vi "SubVgDummi.vi"(0 "Target Voltage, V":dbl=1.0 min=-4.0 max=4.0 step=0.1 format="%.4f", 2 "Sweep rate, V/min":dbl=0.1 min=0.0 max=1.0 step=0.01 format="%.4f", 3 "Custom Folder":string, 5 "optional Bias (V)":dbl=1e-08) -> ()   [LabVIEW 2013]
uses:
  <vilib>/Utility/file.llb/Write To Spreadsheet File (DBL).vi
panel:
  out "Numeric 4":i32
  in  "Commutator":bool
  in  "Commute SorceMeter":enum32{"Radio Selection 1", "Radio Selection 2"}(radio)
  out "Numeric 3":i32
  in  "Channel 2 (Vnano3b)":bool
  in  "Channel 1 (Vnano3)":bool
  out "Numeric":i32
  in  "Capacitance (C) and Loss (L)":bool
  in  "Magnetic Field (B)":bool
  in  "Current (Ik3)":bool
  in  "Voltage (Vk3)":bool
  in  "Current (Ik2)":bool
  in  "Voltage (Vk2)":bool
  in  "Channel 2 (Vnano2b)":bool
  in  "Channel 1 (Vnano2)":bool
  in  "Thermometer 1 (T1)":bool=TRUE
  in  "Channel 2 (Vnano1b)":bool
  in  "Channel 1 (Vnano1)":bool
  in  "Current (Ik1)":bool=TRUE
  in  "Voltage (Vk1)":bool
  out "Numeric Current":dbl
  out "Main Keithly2400 address":string="12"
  out "Delib Time delay":i32
  in  "points at each Vg":i32=1
  out "XY Graph":cluster{dbl[], dbl[]}(graph)={[1.0, 0.8, 0.6000000000000001, 0.4000000000000001, 0.20000000000000007, 5.551115123125783e-17, -0.19999999999999996, -0.39999999999999997, -0.6, -0.8, -1.0], [0.03352775, 0.056811, 0.03911575, 0.04330675, -0.02468015, 0.011641600000000002, 0.10151450000000001, 0.12386675000000001, 0.08288825000000001, -0.00186266, -0.038650000000000004]}
  in  "Time btw \npoints, sec":dbl=1.0 format="%.2f"
  out "Array 2":dbl[][](array[numeric])
  out "array for data":dbl[](array[numeric])
  out "Numeric 2":dbl
  out "Array":string[](array[string])
  in  "Addr 1 lock-in oop":bool
  in  "Ring":u16(ring) caption="Y-axis:" items=["Vg", "I", "R1", "R1oop", "R2", "R2oop", "R3", "R3oop", "Ik1", "T1", "B"]
  out "String":string
  out "Data file:":path
  in  "Set compliance limit, mkA":dbl=0.05 min=0.0 max=1.0 step=0.01 format="%.3f"
  in  "error in (no error)":errorcluster
  in  "Ring 3":u16(ring)=1 items=["1 kOhm", "10 kOhm", "100 kOhm", "1 Mohm", "10 mOhm"]
  in  "Ring 2":u16(ring)=3 items=["1 kOhm", "10 kOhm", "100 kOhm", "1 Mohm", "10 mOhm"]
  in  "Fixed Current mkA":dbl=1.0
  in  "Current is:":T1(radio)
  in  "Ressitance measurements?":bool=TRUE
  in  "Addr 5 lock-in oop":bool
  in  "Addr 4 lock-in oop":bool
  in  "Addr 3 lock-in oop":bool
  in  "Addr 2 lock-in oop":bool
  in  "Addr 5 lock-in":bool
  in  "Addr 4 lock-in":bool
  in  "Addr 3 lock-in":bool=TRUE
  in  "Addr 2 lock-in":bool=TRUE
  in  "Addr 1 lock-in":bool=TRUE
  # "Keithley 2400: address 12"
  # "SourceMeters"
  # "Nanovoltmeters"
  # "Temperature"
  # "Main"
  # "Magnetic Field"
  # "(not recommended, too slow)"
  # "Capacitance & Loss"
  # "(not recommended, too slow)"
  # "(not recommended, too slow)"
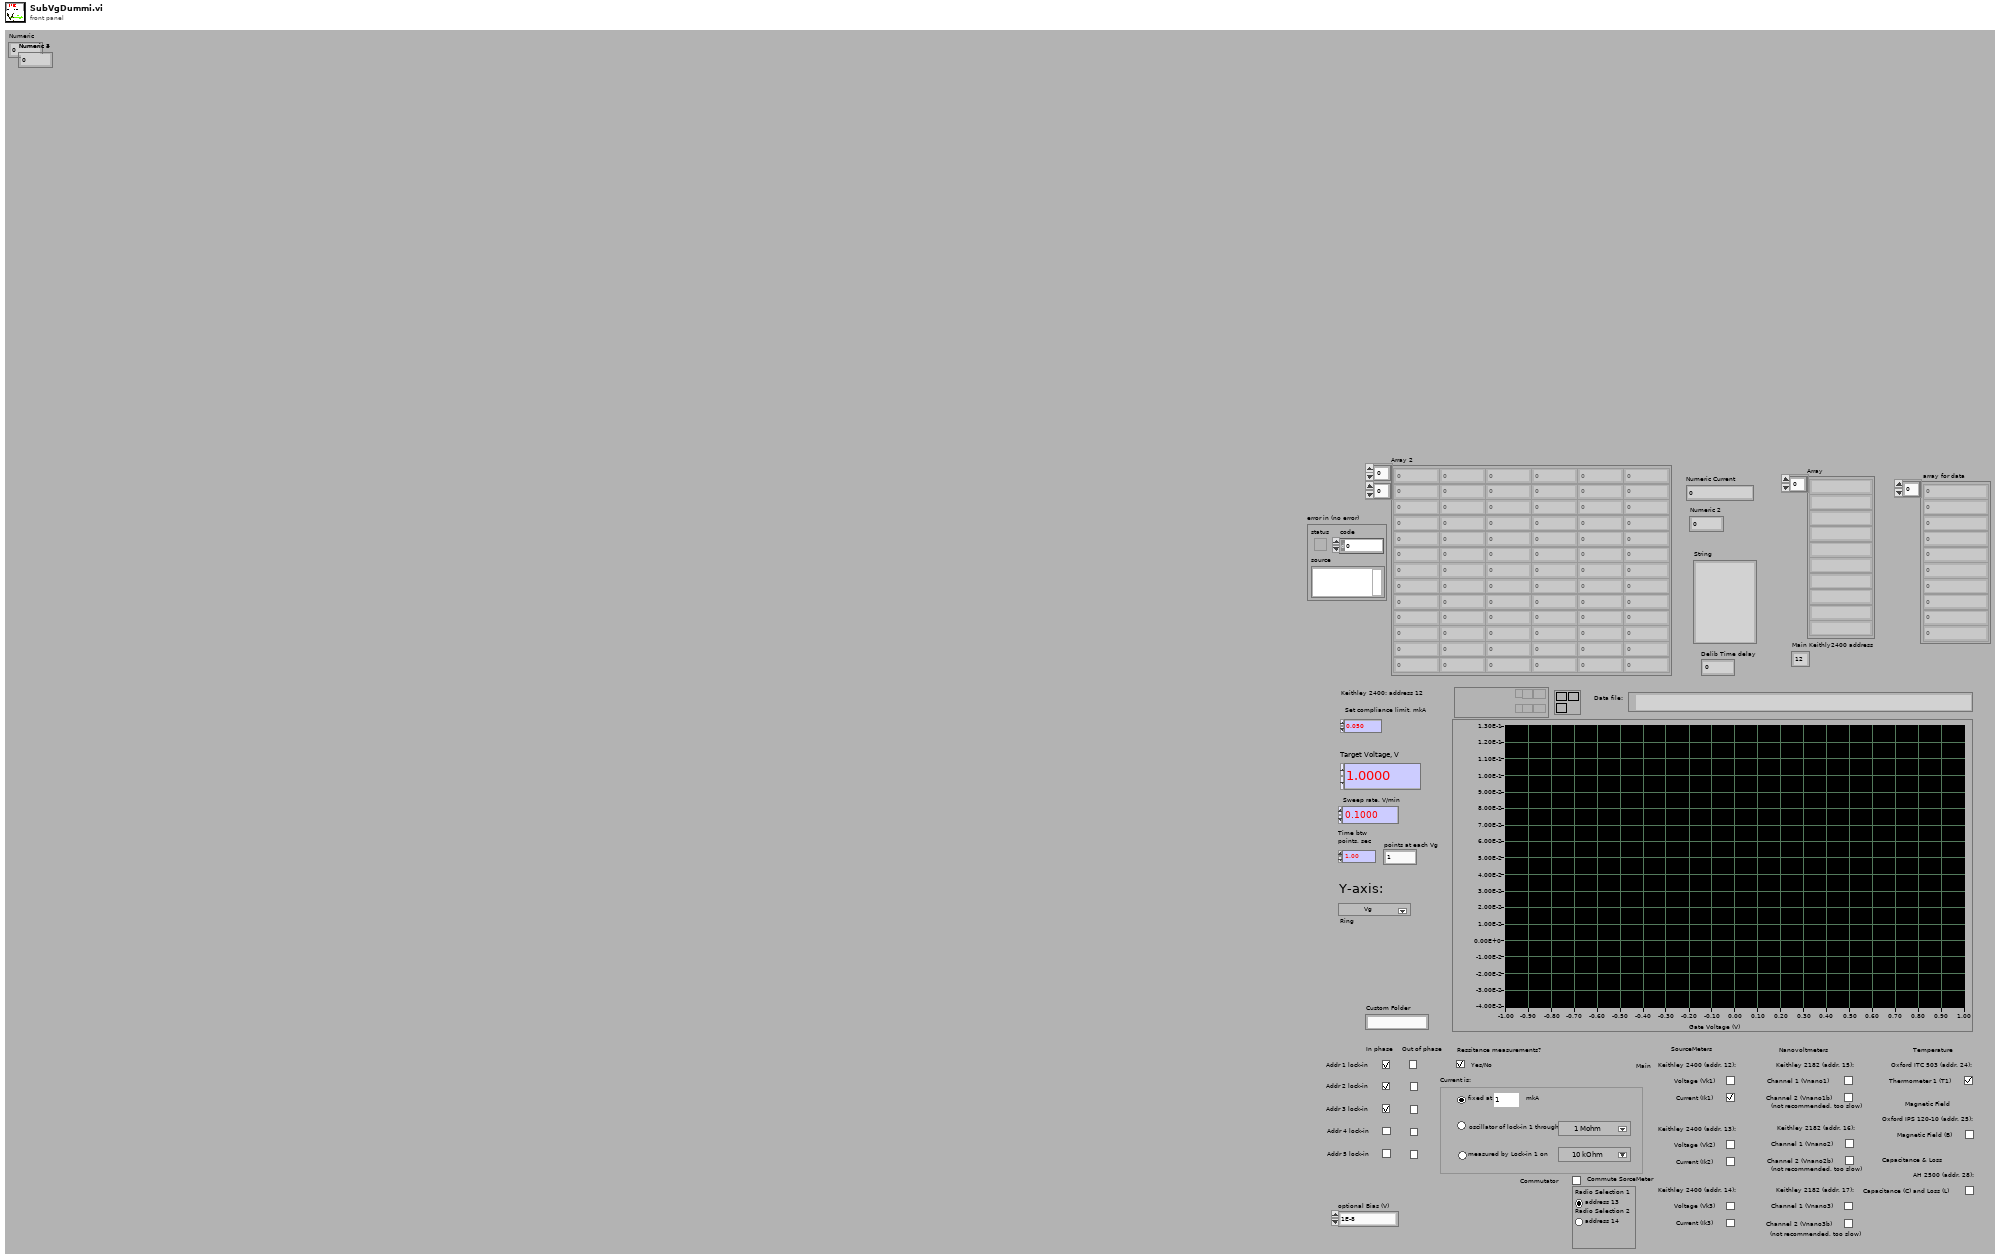
[diagram p1: front panel]
types:
  T1 = enum32{"Radio Selection 1", "Radio Selection 2", "Radio Selection 3"}
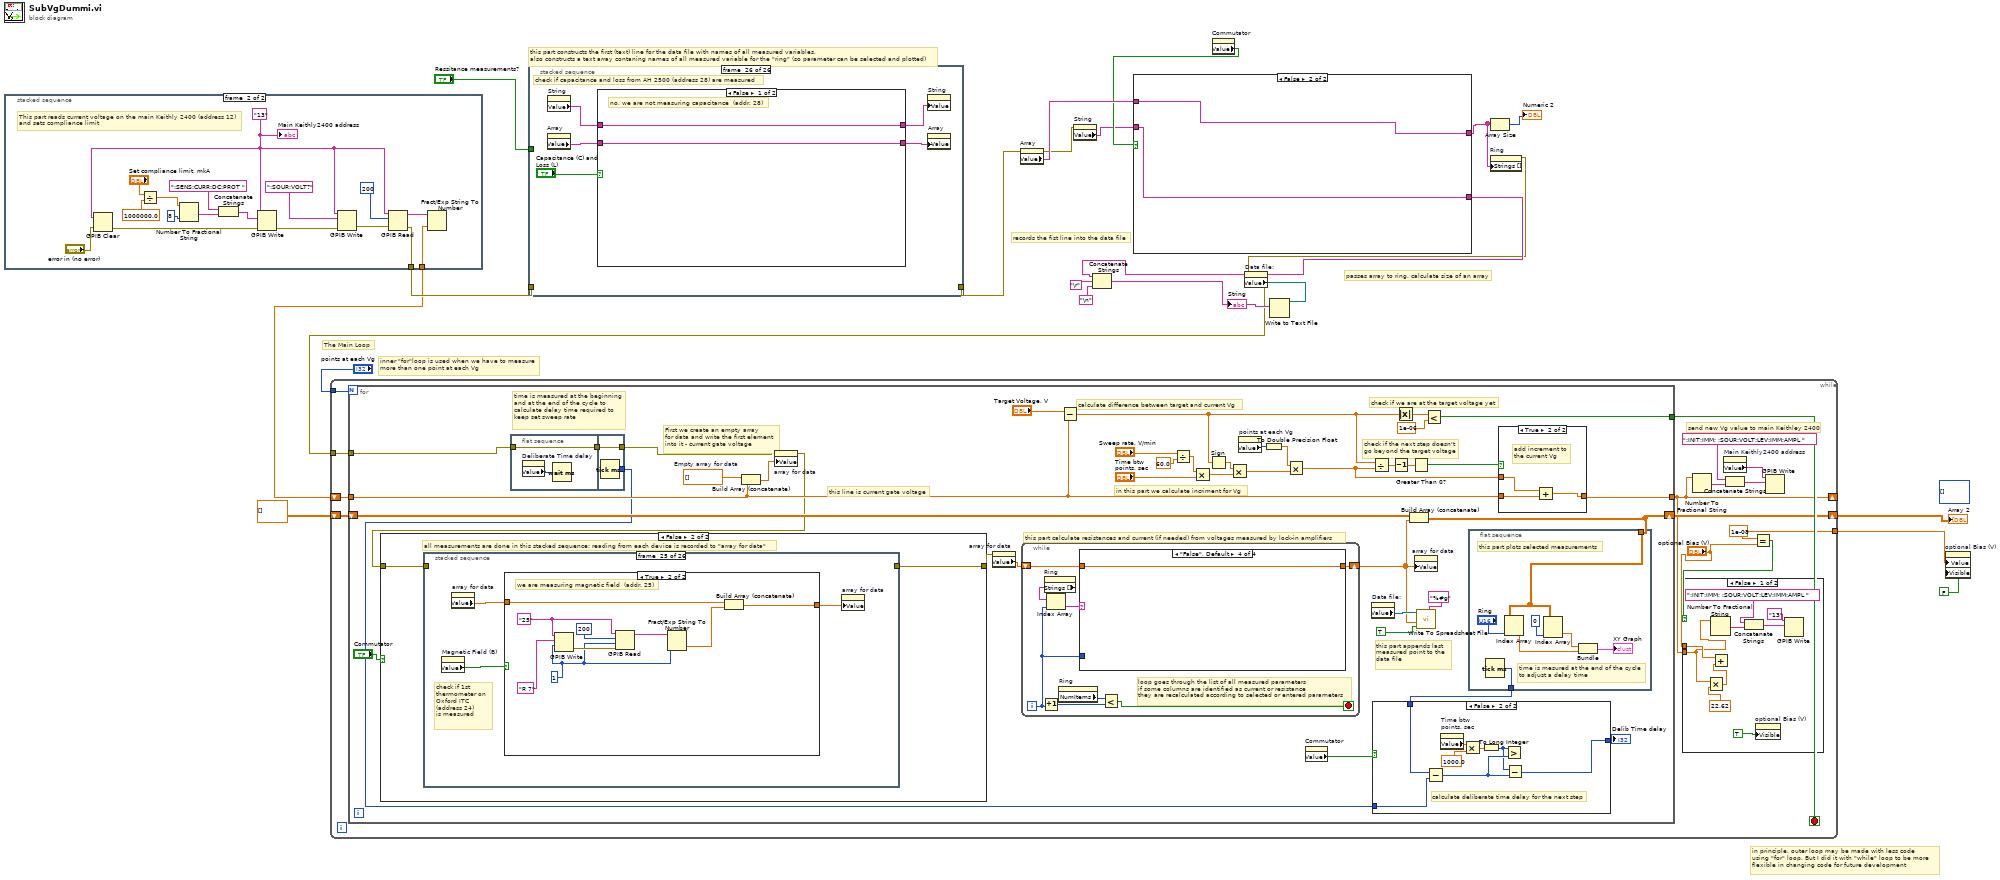
[diagram p0: block diagram]
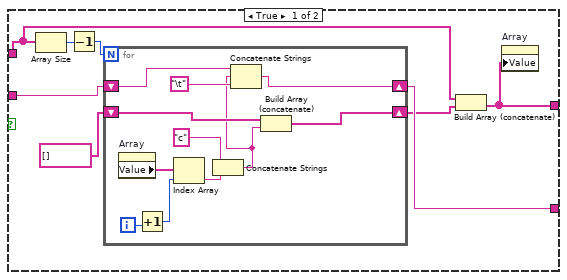
[diagram p2: hidden frame]
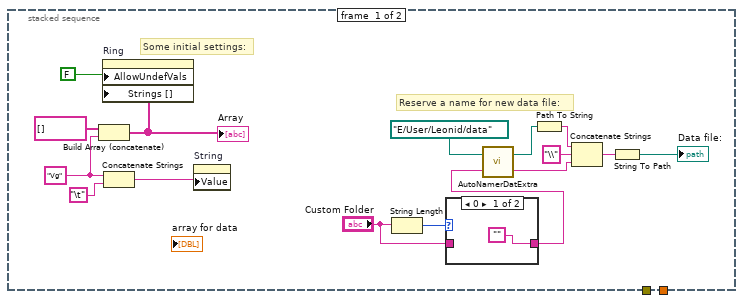
[diagram p3: hidden frame]
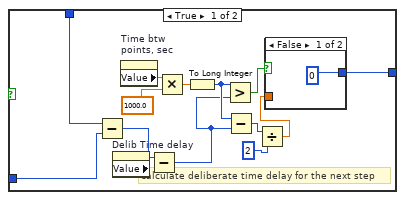
[diagram p6: hidden frame]
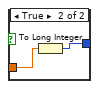
[diagram p7: hidden frame]
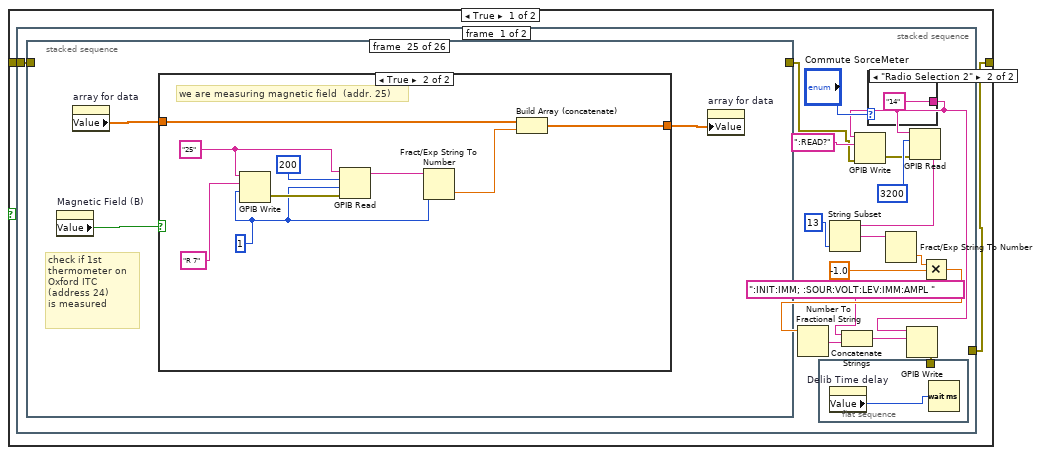
[diagram p8: hidden frame]
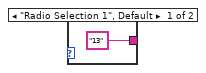
[diagram p9: hidden frame]
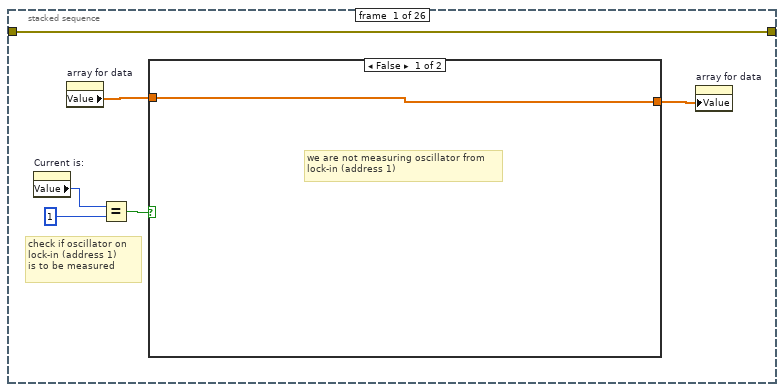
[diagram p10: hidden frame]
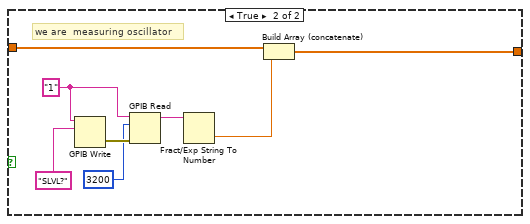
[diagram p11: hidden frame]
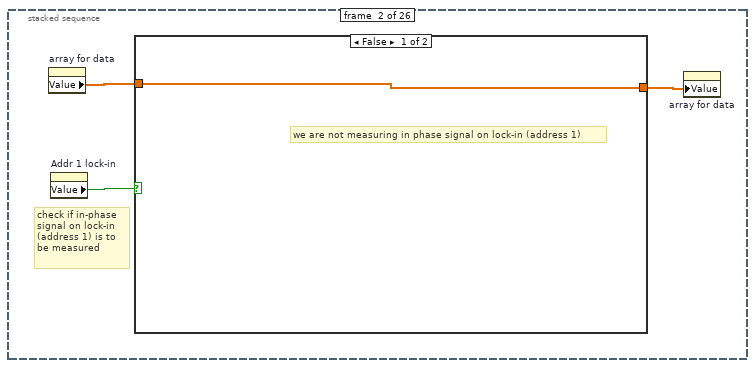
[diagram p12: hidden frame]
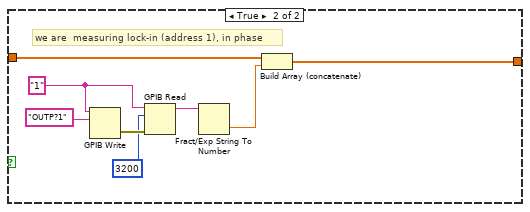
[diagram p13: hidden frame]
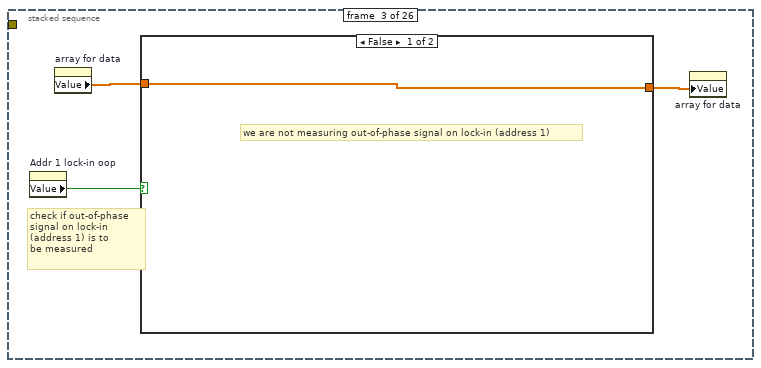
[diagram p14: hidden frame]
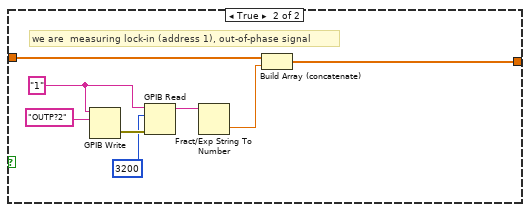
[diagram p15: hidden frame]
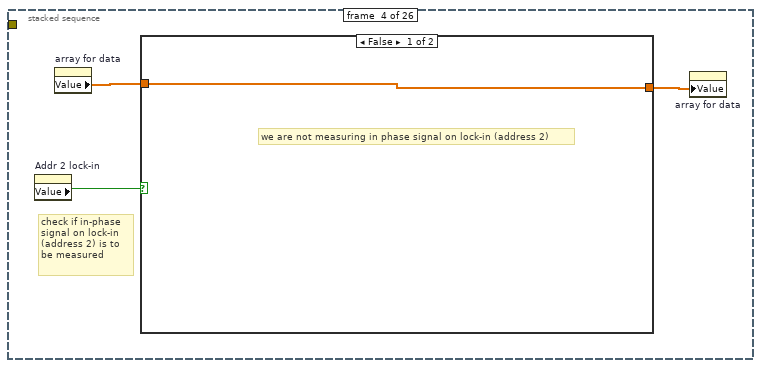
[diagram p16: hidden frame]
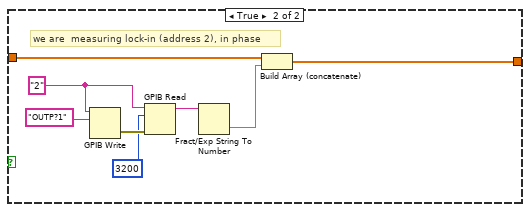
[diagram p17: hidden frame]
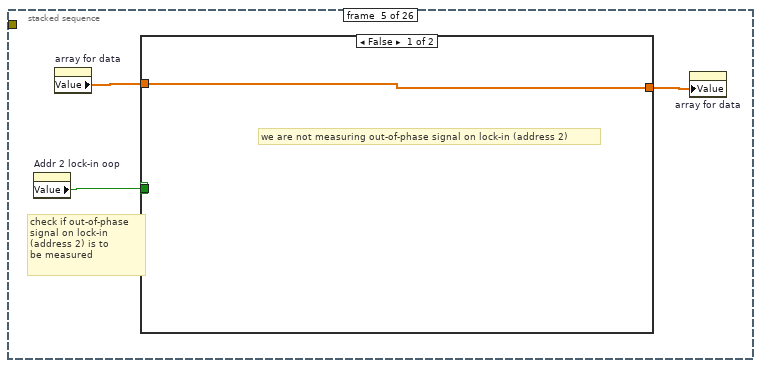
[diagram p18: hidden frame]
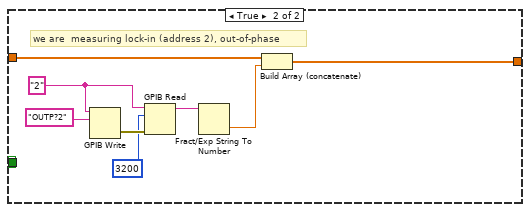
[diagram p19: hidden frame]
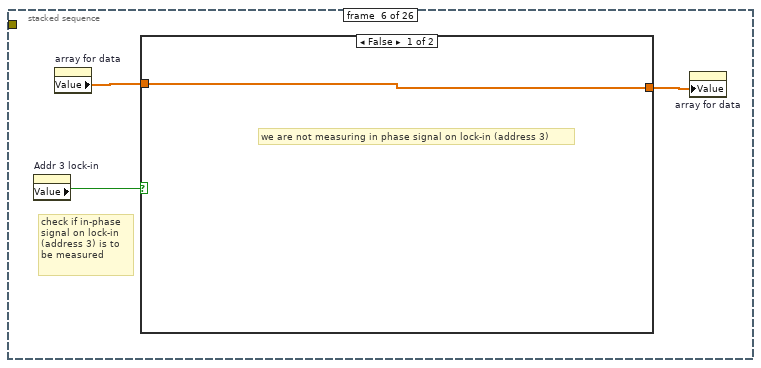
[diagram p20: hidden frame]
diagram:
  (unwired) i32[][] []
  # "passes array to ring, calculate size of an array"
  # "in principle, outer loop may be made with less code\nusing \"for\" loop. But I did it with \"while\" loop to be more \nflexible in changing code for future development"
  # "inner \"for\"loop is used when we have to measure\nmore than one point at each Vg"
  # "The Main Loop"
  # "records the fist line into the data file"
  # "this part constructs the first (text) line for the data file with names of all measured variables,\nalso constructs a text array contaning names of all measured variable for the \"ring\" (so parameter can be selected and plotted)"
  n1 = stacked-sequence {
    tunnel: [_ w43] -> w22
    tunnel: [_ w42] -> w9
    frame #0 {
      w28 = "Vg"
      # "Some initial settings:"
      # "Reserve a name for new data file:"
      n2 = Build Array (concatenate)(string[] [], w28) -> (w30:string[])
      "Array" <- w30
      n3 = property on="Ring" class="Ring (strict)"("AllowUndefVals"=FALSE, "Strings []"=w30) -> ()  [unwired: 2 in, 2 out]
      n4 = Concatenate Strings(w28, "\t") -> (w29:string)
      n5 = property on="String" class="Str"("Value"=w29) -> ()  [unwired: 2 in, 2 out]
      n6 = String Length(string="Custom Folder") -> (length=w25:i32)
      n7 = case shown="0" w25 {
        tunnel: "Custom Folder" -> [_ w40]
        tunnel: ["" w40] -> w23
        frame 0 {
        }
        frame 1, Default {
        }
      }
      n8 = call "AutoNamerDatExtra.vi"("ExtraString"=w23, "Custom User Path"=path "E:/User/Leonid/data") -> ("String"=w38:string, "Path"=w37:path)
      n9 = Path To String(path=w37) -> (string=w32:string)
      n10 = Concatenate Strings(w32, "\\", w38) -> (w34:string)
      n11 = String To Path(string=w34) -> (path=→"Data file:":path)
    }
    frame #1 {
      w41 = "13"
      # "This part reads current voltage on the main Keithly 2400 (address 12)\nand sets compliance limit"
      n12 = GPIB Clear(2:"error in (no error)", 3:w41) -> (0:w50:errorcluster)  [unwired: 1 out]
      n13 = Divide(x="Set compliance limit, mkA", y=1000000.0) -> (x/y=w56:dbl)
      n14 = Number To Fractional String(number=w56, precision (6)=i16 8) -> (F-format string=w52:string)  [unwired: 2 in]
      n15 = Concatenate Strings(":SENS:CURR:DC:PROT " ("data"), w52) -> (w51:string)
      n16 = GPIB Write(0:w41, 1:w51, 3:w50) -> (6:w45:errorcluster)  [unwired: 2 in, 1 out]
      n17 = GPIB Write(0:w41, 1:":SOUR:VOLT?" ("data"), 3:w45) -> (6:w49:errorcluster)  [unwired: 2 in, 1 out]
      n18 = GPIB Read(0:w41, 1:200 ("byte count"), 3:w49) -> (5:w47:string, 7:w43:errorcluster)  [unwired: 2 in, 1 out]
      n19 = Fract/Exp String To Number(string=w47) -> (number=w42:dbl)  [unwired: 3 in, 1 out]
      "Main Keithly2400 address" <- w41
    }
  }
  n20 = stacked-sequence {
    tunnel: "Ressitance measurements?" -> [w65 w80 w104 w127 w145 w163 w181 w199 w217 w235 w253 _ _ _ _ _ _ _ _ _ _ _ _ _ _ _]
    tunnel: w22 -> [_ w77 _ _ _ _ _ _ _ _ _ _ _ _ _ _ _ _ _ _ _ _ _ _ _ _]
    tunnel: [_ w77 _ _ _ _ _ _ _ _ _ _ _ _ _ _ _ _ _ _ _ _ _ _ _ _] -> w19
    frame #0 {
      # "check if oscillator of  lock-in (address 1) is to be measured"
      n21 = property on="Array" class="Arr (strict)"() -> ("Value"=w60:string[])  [unwired: 2 in, 2 out]
      n22 = property on="String" class="Str"() -> ("Value"=w64:string)  [unwired: 2 in, 2 out]
      n23 = Equal?(x="Current is:", y=1) -> (x = y?=w61:bool)
      n24 = case shown="False" w61 {
        tunnel: w65 -> [_ _]
        tunnel: [w67 w68] -> w63
        tunnel: w64 -> [w67 w71]
        tunnel: w60 -> [w66 w70]
        tunnel: [w66 w69] -> w59
        frame False {
          # "we are not measuring oscillator from\nlock-in (address 1)"
        }
        frame True {
          w72 = "I"
          # "we are  measuring oscillator"
          n25 = GPIB Clear(3:"1") -> ()  [unwired: 1 in, 2 out]
          n26 = Concatenate Strings(w71, w72, "\t") -> (w68:string)
          n27 = Build Array (concatenate)(w70, w72) -> (w69:string[])
        }
      }
      n28 = property on="Array" class="Arr (strict)"("Value"=w59) -> ()  [unwired: 2 in, 2 out]
      n29 = property on="String" class="Str"("Value"=w63) -> ()  [unwired: 2 in, 2 out]
    }
    frame #1 {
      # "check if lock-in (address 1) is to be measured"
      n30 = property on="Array" class="Arr (strict)"() -> ("Value"=w76:string[])  [unwired: 2 in, 2 out]
      n31 = property on="String" class="Str"() -> ("Value"=w79:string)  [unwired: 2 in, 2 out]
      n32 = case shown="False" "Addr 1 lock-in" {
        tunnel: w80 -> [_ w91]
        tunnel: [w83 w87] -> w78
        tunnel: w79 -> [w83 w86]
        tunnel: w76 -> [w82 w88]
        tunnel: [w82 w89] -> w75
        frame False {
          # "we are not measuring in phase signal from\nlock-in (address 1)"
        }
        frame True {
          # "are we measuring resistance?"
          n33 = GPIB Clear(3:"1") -> ()  [unwired: 1 in, 2 out]
          n34 = case shown="True" w91 {
            tunnel: ["V1" w93] -> w84
            frame False {
              # "no, we are not measuring resistanse;\nall lock-ins are measuring voltage"
            }
            frame True {
              # "are we measuring current as well?"
              n35 = property on="Current is:" class="RadioBtnsControl (strict)"() -> ("Value"=w95:T1)  [unwired: 2 in, 2 out]
              n36 = Equal?(x=w95, y=2) -> (x = y?=w96:bool)
              n37 = case shown="False" w96 {
                tunnel: ["R1" "I"] -> w93
                frame False {
                  # "no, we are not \nmeasuring current\nby lock-in \n(address 1); \nso this lock-in is \nmeasuring resistance"
                }
                frame True {
                  # "yes, we are measuring \ncurrent by lock-in \n(address 1) as \nvoltage drop on \nknown resistance"
                }
              }
            }
          }
          n38 = Concatenate Strings(w86, w84, "\t") -> (w87:string)
          n39 = Build Array (concatenate)(w88, w84) -> (w89:string[])
        }
      }
      n40 = property on="Array" class="Arr (strict)"("Value"=w75) -> ()  [unwired: 2 in, 2 out]
      n41 = property on="String" class="Str"("Value"=w78) -> ()  [unwired: 2 in, 2 out]
    }
    frame #2 {
      # "check if out-of-phase signal on  lock-in (address 1) is to be measured"
      n42 = property on="Array" class="Arr (strict)"() -> ("Value"=w101:string[])  [unwired: 2 in, 2 out]
      n43 = property on="String" class="Str"() -> ("Value"=w103:string)  [unwired: 2 in, 2 out]
      n44 = case shown="False" "Addr 1 lock-in oop" {
        tunnel: w104 -> [_ w114]
        tunnel: [w106 w110] -> w102
        tunnel: w103 -> [w106 w109]
        tunnel: w101 -> [w105 w111]
        tunnel: [w105 w112] -> w100
        frame False {
          # "we are not measuring iout-of-phase signal from\nlock-in (address 1)"
        }
        frame True {
          # "are we measuring resistance?"
          n45 = GPIB Clear(3:"1") -> ()  [unwired: 1 in, 2 out]
          n46 = case shown="True" w114 {
            tunnel: ["V1oop" w116] -> w107
            frame False {
              # "no, we are not measuring resistance;\nall lock-ins are measuring voltage"
            }
            frame True {
              # "are we measuring out-of-phase current as well?"
              n47 = property on="Current is:" class="RadioBtnsControl (strict)"() -> ("Value"=w118:T1)  [unwired: 2 in, 2 out]
              n48 = Equal?(x=w118, y=2) -> (x = y?=w119:bool)
              n49 = case shown="False" w119 {
                tunnel: ["R1oop" "Ioop"] -> w116
                frame False {
                  # "no, we are not \nmeasuring current\nby lock-in \n(address 1); so this \nlock-in is measuring\nout-of-phase resistance"
                }
                frame True {
                  # "yes, we are measuring \nout-of phase current \nby lock-in (address 1) \nas voltage drop on \nknown resistance"
                }
              }
            }
          }
          n50 = Concatenate Strings(w109, w107, "\t") -> (w110:string)
          n51 = Build Array (concatenate)(w111, w107) -> (w112:string[])
        }
      }
      n52 = property on="Array" class="Arr (strict)"("Value"=w100) -> ()  [unwired: 2 in, 2 out]
      n53 = property on="String" class="Str"("Value"=w102) -> ()  [unwired: 2 in, 2 out]
    }
    frame #3 {
      # "check if in-phase signal on  lock-in (address 2) is to be measured"
      n54 = property on="Array" class="Arr (strict)"() -> ("Value"=w124:string[])  [unwired: 2 in, 2 out]
      n55 = property on="String" class="Str"() -> ("Value"=w126:string)  [unwired: 2 in, 2 out]
      n56 = case shown="False" "Addr 2 lock-in" {
        tunnel: w127 -> [_ w137]
        tunnel: [w129 w133] -> w125
        tunnel: w126 -> [w129 w132]
        tunnel: w124 -> [w128 w134]
        tunnel: [w128 w135] -> w123
        frame False {
          # "we are not measuring in-phase signal from\nlock-in (address 2)"
        }
        frame True {
          # "are we measuring resistance?"
          n57 = GPIB Clear(3:"2") -> ()  [unwired: 1 in, 2 out]
          n58 = case shown="True" w137 {
            tunnel: ["R2" "V2"] -> w130
            frame True {
              # "we are measuring \nresistance by lock-in \n(address 2)"
            }
            frame False, Default {
              # "no, we are not measuring resistance;\nall lock-ins are measuring voltage"
            }
          }
          n59 = Concatenate Strings(w132, w130, "\t") -> (w133:string)
          n60 = Build Array (concatenate)(w134, w130) -> (w135:string[])
        }
      }
      n61 = property on="Array" class="Arr (strict)"("Value"=w123) -> ()  [unwired: 2 in, 2 out]
      n62 = property on="String" class="Str"("Value"=w125) -> ()  [unwired: 2 in, 2 out]
    }
    frame #4 {
      # "check if out-of-phase signal on  lock-in (address 2) is to be measured"
      n63 = property on="Array" class="Arr (strict)"() -> ("Value"=w142:string[])  [unwired: 2 in, 2 out]
      n64 = property on="String" class="Str"() -> ("Value"=w144:string)  [unwired: 2 in, 2 out]
      n65 = case shown="False" "Addr 2 lock-in oop" {
        tunnel: w145 -> [_ w155]
        tunnel: [w147 w151] -> w143
        tunnel: w144 -> [w147 w150]
        tunnel: w142 -> [w146 w152]
        tunnel: [w146 w153] -> w141
        frame False {
          # "we are not measuring out-of-phase signal from\nlock-in (address 2)"
        }
        frame True {
          # "are we measuring resistance?"
          n66 = GPIB Clear(3:"2") -> ()  [unwired: 1 in, 2 out]
          n67 = case shown="True" w155 {
            tunnel: ["R2oop" "V2oop"] -> w148
            frame True {
              # "we are measuring out-of-phase resistance by lock-in (address 2)\n(address 2)"
            }
            frame False, Default {
              # "no, we are not measuring resistance;\nall lock-ins are measuring voltage"
            }
          }
          n68 = Concatenate Strings(w150, w148, "\t") -> (w151:string)
          n69 = Build Array (concatenate)(w152, w148) -> (w153:string[])
        }
      }
      n70 = property on="Array" class="Arr (strict)"("Value"=w141) -> ()  [unwired: 2 in, 2 out]
      n71 = property on="String" class="Str"("Value"=w143) -> ()  [unwired: 2 in, 2 out]
    }
    frame #5 {
      # "check if in-phase signal on  lock-in (address 3) is to be measured"
      n72 = property on="Array" class="Arr (strict)"() -> ("Value"=w160:string[])  [unwired: 2 in, 2 out]
      n73 = property on="String" class="Str"() -> ("Value"=w162:string)  [unwired: 2 in, 2 out]
      n74 = case shown="False" "Addr 3 lock-in" {
        tunnel: w163 -> [_ w173]
        tunnel: [w165 w169] -> w161
        tunnel: w162 -> [w165 w168]
        tunnel: w160 -> [w164 w170]
        tunnel: [w164 w171] -> w159
        frame False {
          # "we are not measuring in-phase signal from\nlock-in (address 3)"
        }
        frame True {
          # "are we measuring resistance?"
          n75 = GPIB Clear(3:"3") -> ()  [unwired: 1 in, 2 out]
          n76 = case shown="True" w173 {
            tunnel: ["R3" "V3"] -> w166
            frame True {
              # "we are measuring \nresistance by lock-in \n(address 3)"
            }
            frame False, Default {
              # "no, we are not measuring resistance;\nall lock-ins are measuring voltage"
            }
          }
          n77 = Concatenate Strings(w168, w166, "\t") -> (w169:string)
          n78 = Build Array (concatenate)(w170, w166) -> (w171:string[])
        }
      }
      n79 = property on="Array" class="Arr (strict)"("Value"=w159) -> ()  [unwired: 2 in, 2 out]
      n80 = property on="String" class="Str"("Value"=w161) -> ()  [unwired: 2 in, 2 out]
    }
    frame #6 {
      # "check if out-of-phase signal on  lock-in (address 3) is to be measured"
      n81 = property on="Array" class="Arr (strict)"() -> ("Value"=w178:string[])  [unwired: 2 in, 2 out]
      n82 = property on="String" class="Str"() -> ("Value"=w180:string)  [unwired: 2 in, 2 out]
      n83 = case shown="False" "Addr 3 lock-in oop" {
        tunnel: w181 -> [_ w191]
        tunnel: [w183 w187] -> w179
        tunnel: w180 -> [w183 w186]
        tunnel: w178 -> [w182 w188]
        tunnel: [w182 w189] -> w177
        frame False {
          # "we are not measuring out-of-phase signal from\nlock-in (address 3)"
        }
        frame True {
          # "are we measuring resistance?"
          n84 = GPIB Clear(3:"3") -> ()  [unwired: 1 in, 2 out]
          n85 = case shown="True" w191 {
            tunnel: ["R3oop" "V3oop"] -> w184
            frame True {
              # "we are measuring out-of-phase resistance by lock-in (address 3)\n(address 2)"
            }
            frame False, Default {
              # "no, we are not measuring resistance;\nall lock-ins are measuring voltage"
            }
          }
          n86 = Concatenate Strings(w186, w184, "\t") -> (w187:string)
          n87 = Build Array (concatenate)(w188, w184) -> (w189:string[])
        }
      }
      n88 = property on="Array" class="Arr (strict)"("Value"=w177) -> ()  [unwired: 2 in, 2 out]
      n89 = property on="String" class="Str"("Value"=w179) -> ()  [unwired: 2 in, 2 out]
    }
    frame #7 {
      # "check if in-phase signal on  lock-in (address 4) is to be measured"
      n90 = property on="Array" class="Arr (strict)"() -> ("Value"=w196:string[])  [unwired: 2 in, 2 out]
      n91 = property on="String" class="Str"() -> ("Value"=w198:string)  [unwired: 2 in, 2 out]
      n92 = case shown="False" "Addr 4 lock-in" {
        tunnel: w199 -> [_ w209]
        tunnel: [w201 w205] -> w197
        tunnel: w198 -> [w201 w204]
        tunnel: w196 -> [w200 w206]
        tunnel: [w200 w207] -> w195
        frame False {
          # "we are not measuring in-phase signal from\nlock-in (address 4)"
        }
        frame True {
          # "are we measuring resistance?"
          n93 = GPIB Clear(3:"4") -> ()  [unwired: 1 in, 2 out]
          n94 = case shown="True" w209 {
            tunnel: ["R4" "V4"] -> w202
            frame True {
              # "we are measuring \nresistance by lock-in \n(address 4)"
            }
            frame False, Default {
              # "no, we are not measuring resistance;\nall lock-ins are measuring voltage"
            }
          }
          n95 = Concatenate Strings(w204, w202, "\t") -> (w205:string)
          n96 = Build Array (concatenate)(w206, w202) -> (w207:string[])
        }
      }
      n97 = property on="Array" class="Arr (strict)"("Value"=w195) -> ()  [unwired: 2 in, 2 out]
      n98 = property on="String" class="Str"("Value"=w197) -> ()  [unwired: 2 in, 2 out]
    }
    frame #8 {
      # "check if out-of-phase signal on  lock-in (address 4) is to be measured"
      n99 = property on="Array" class="Arr (strict)"() -> ("Value"=w214:string[])  [unwired: 2 in, 2 out]
      n100 = property on="String" class="Str"() -> ("Value"=w216:string)  [unwired: 2 in, 2 out]
      n101 = case shown="False" "Addr 4 lock-in oop" {
        tunnel: w217 -> [_ w227]
        tunnel: [w219 w223] -> w215
        tunnel: w216 -> [w219 w222]
        tunnel: w214 -> [w218 w224]
        tunnel: [w218 w225] -> w213
        frame False {
          # "we are not measuring out-of-phase signal from\nlock-in (address 4)"
        }
        frame True {
          # "are we measuring resistance?"
          n102 = GPIB Clear(3:"4") -> ()  [unwired: 1 in, 2 out]
          n103 = case shown="True" w227 {
            tunnel: ["R4oop" "V4oop"] -> w220
            frame True {
              # "we are measuring out-of-phase resistance by lock-in (address 4)\n(address 2)"
            }
            frame False, Default {
              # "no, we are not measuring resistance;\nall lock-ins are measuring voltage"
            }
          }
          n104 = Concatenate Strings(w222, w220, "\t") -> (w223:string)
          n105 = Build Array (concatenate)(w224, w220) -> (w225:string[])
        }
      }
      n106 = property on="Array" class="Arr (strict)"("Value"=w213) -> ()  [unwired: 2 in, 2 out]
      n107 = property on="String" class="Str"("Value"=w215) -> ()  [unwired: 2 in, 2 out]
    }
    frame #9 {
      # "check if in-phase signal on  lock-in (address 5) is to be measured"
      n108 = property on="Array" class="Arr (strict)"() -> ("Value"=w232:string[])  [unwired: 2 in, 2 out]
      n109 = property on="String" class="Str"() -> ("Value"=w234:string)  [unwired: 2 in, 2 out]
      n110 = case shown="False" "Addr 5 lock-in" {
        tunnel: w235 -> [_ w245]
        tunnel: [w237 w241] -> w233
        tunnel: w234 -> [w237 w240]
        tunnel: w232 -> [w236 w242]
        tunnel: [w236 w243] -> w231
        frame False {
          # "we are not measuring in-phase signal from\nlock-in (address 5)"
        }
        frame True {
          # "are we measuring resistance?"
          n111 = GPIB Clear(3:"5") -> ()  [unwired: 1 in, 2 out]
          n112 = case shown="True" w245 {
            tunnel: ["R5" "V5"] -> w238
            frame True {
              # "we are measuring \nresistance by lock-in \n(address 5)"
            }
            frame False, Default {
              # "no, we are not measuring resistance;\nall lock-ins are measuring voltage"
            }
          }
          n113 = Concatenate Strings(w240, w238, "\t") -> (w241:string)
          n114 = Build Array (concatenate)(w242, w238) -> (w243:string[])
        }
      }
      n115 = property on="Array" class="Arr (strict)"("Value"=w231) -> ()  [unwired: 2 in, 2 out]
      n116 = property on="String" class="Str"("Value"=w233) -> ()  [unwired: 2 in, 2 out]
    }
    frame #10 {
      # "check if out-of-phase signal on  lock-in (address 5) is to be measured"
      n117 = property on="Array" class="Arr (strict)"() -> ("Value"=w250:string[])  [unwired: 2 in, 2 out]
      n118 = property on="String" class="Str"() -> ("Value"=w252:string)  [unwired: 2 in, 2 out]
      n119 = case shown="False" "Addr 5 lock-in oop" {
        tunnel: w253 -> [_ w263]
        tunnel: [w255 w259] -> w251
        tunnel: w252 -> [w255 w258]
        tunnel: w250 -> [w254 w260]
        tunnel: [w254 w261] -> w249
        frame False {
          # "we are not measuring out-of-phase signal from\nlock-in (address 5)"
        }
        frame True {
          # "are we measuring resistance?"
          n120 = GPIB Clear(3:"5") -> ()  [unwired: 1 in, 2 out]
          n121 = case shown="True" w263 {
            tunnel: ["R5oop" "V5oop"] -> w256
            frame True {
              # "we are measuring out-of-phase resistance by lock-in (address 5)\n(address 2)"
            }
            frame False, Default {
              # "no, we are not measuring resistance;\nall lock-ins are measuring voltage"
            }
          }
          n122 = Concatenate Strings(w258, w256, "\t") -> (w259:string)
          n123 = Build Array (concatenate)(w260, w256) -> (w261:string[])
        }
      }
      n124 = property on="Array" class="Arr (strict)"("Value"=w249) -> ()  [unwired: 2 in, 2 out]
      n125 = property on="String" class="Str"("Value"=w251) -> ()  [unwired: 2 in, 2 out]
    }
    frame #11 {
      # "check if voltage on main Keithley 2400 (addr. 12) is measured"
      n126 = property on="Array" class="Arr (strict)"() -> ("Value"=w268:string[])  [unwired: 2 in, 2 out]
      n127 = property on="String" class="Str"() -> ("Value"=w270:string)  [unwired: 2 in, 2 out]
      n128 = case shown="False" "Voltage (Vk1)" {
        tunnel: [w272 w276] -> w269
        tunnel: w270 -> [w272 w275]
        tunnel: w268 -> [w271 w277]
        tunnel: [w271 w278] -> w267
        frame False {
          # "no , we aren't measuring voltage \non main Keithley 2400 (addr. 12)"
        }
        frame True {
          w273 = "Vk1"
          # "yes , we are measuring voltage \non main Keithley 2400 (addr. 12)"
          n129 = GPIB Clear(3:"12") -> ()  [unwired: 1 in, 2 out]
          n130 = Concatenate Strings(w275, w273, "\t") -> (w276:string)
          n131 = Build Array (concatenate)(w277, w273) -> (w278:string[])
        }
      }
      n132 = property on="String" class="Str"("Value"=w269) -> ()  [unwired: 2 in, 2 out]
      n133 = property on="Array" class="Arr (strict)"("Value"=w267) -> ()  [unwired: 2 in, 2 out]
    }
    frame #12 {
      # "check if current on main Keithley 2400 (addr. 12) is measured"
      n134 = property on="Array" class="Arr (strict)"() -> ("Value"=w282:string[])  [unwired: 2 in, 2 out]
      n135 = property on="String" class="Str"() -> ("Value"=w284:string)  [unwired: 2 in, 2 out]
      n136 = case shown="True" "Current (Ik1)" {
        tunnel: [w286 w290] -> w283
        tunnel: w284 -> [w286 w289]
        tunnel: w282 -> [w285 w291]
        tunnel: [w285 w292] -> w281
        frame False {
          # "no , we aren't measuring current\non main Keithley 2400 (addr. 12)"
        }
        frame True {
          w287 = "Ik1"
          # "yes , we are measuring current \non main Keithley 2400 (addr. 12)"
          n137 = GPIB Clear(3:"12") -> ()  [unwired: 1 in, 2 out]
          n138 = Concatenate Strings(w289, w287, "\t") -> (w290:string)
          n139 = Build Array (concatenate)(w291, w287) -> (w292:string[])
        }
      }
      n140 = property on="String" class="Str"("Value"=w283) -> ()  [unwired: 2 in, 2 out]
      n141 = property on="Array" class="Arr (strict)"("Value"=w281) -> ()  [unwired: 2 in, 2 out]
    }
    frame #13 {
      # "check if voltage on additional Keithley 2400 (addr. 13) is measured"
      n142 = property on="Array" class="Arr (strict)"() -> ("Value"=w296:string[])  [unwired: 2 in, 2 out]
      n143 = property on="String" class="Str"() -> ("Value"=w298:string)  [unwired: 2 in, 2 out]
      n144 = case shown="False" "Voltage (Vk2)" {
        tunnel: [w300 w304] -> w297
        tunnel: w298 -> [w300 w303]
        tunnel: w296 -> [w299 w305]
        tunnel: [w299 w306] -> w295
        frame False {
          # "no , we aren't measuring voltage \non Keithley 2400 (addr. 13)"
        }
        frame True {
          w301 = "Vk2"
          # "yes , we are measuring voltage \non Keithley 2400 (addr. 13)"
          n145 = GPIB Clear(3:"13") -> ()  [unwired: 1 in, 2 out]
          n146 = Concatenate Strings(w303, w301, "\t") -> (w304:string)
          n147 = Build Array (concatenate)(w305, w301) -> (w306:string[])
        }
      }
      n148 = property on="String" class="Str"("Value"=w297) -> ()  [unwired: 2 in, 2 out]
      n149 = property on="Array" class="Arr (strict)"("Value"=w295) -> ()  [unwired: 2 in, 2 out]
    }
    frame #14 {
      # "check if current on additional Keithley 2400 (addr. 13) is measured"
      n150 = property on="Array" class="Arr (strict)"() -> ("Value"=w310:string[])  [unwired: 2 in, 2 out]
      n151 = property on="String" class="Str"() -> ("Value"=w312:string)  [unwired: 2 in, 2 out]
      n152 = case shown="False" "Current (Ik2)" {
        tunnel: [w314 w318] -> w311
        tunnel: w312 -> [w314 w317]
        tunnel: w310 -> [w313 w319]
        tunnel: [w313 w320] -> w309
        frame False {
          # "no , we aren't measuring current\non Keithley 2400 (addr. 13)"
        }
        frame True {
          w315 = "Ik2"
          # "yes , we are measuring current \non Keithley 2400 (addr. 13)"
          n153 = GPIB Clear(3:"13") -> ()  [unwired: 1 in, 2 out]
          n154 = Concatenate Strings(w317, w315, "\t") -> (w318:string)
          n155 = Build Array (concatenate)(w319, w315) -> (w320:string[])
        }
      }
      n156 = property on="String" class="Str"("Value"=w311) -> ()  [unwired: 2 in, 2 out]
      n157 = property on="Array" class="Arr (strict)"("Value"=w309) -> ()  [unwired: 2 in, 2 out]
    }
    frame #15 {
      # "check if voltage on additional Keithley 2400 (addr. 14) is measured"
      n158 = property on="Array" class="Arr (strict)"() -> ("Value"=w324:string[])  [unwired: 2 in, 2 out]
      n159 = property on="String" class="Str"() -> ("Value"=w326:string)  [unwired: 2 in, 2 out]
      n160 = case shown="False" "Voltage (Vk3)" {
        tunnel: [w328 w332] -> w325
        tunnel: w326 -> [w328 w331]
        tunnel: w324 -> [w327 w333]
        tunnel: [w327 w334] -> w323
        frame False {
          # "no , we aren't measuring voltage \non Keithley 2400 (addr. 14)"
        }
        frame True {
          w329 = "Vk3"
          # "yes , we are measuring voltage \non Keithley 2400 (addr. 14)"
          n161 = GPIB Clear(3:"14") -> ()  [unwired: 1 in, 2 out]
          n162 = Concatenate Strings(w331, w329, "\t") -> (w332:string)
          n163 = Build Array (concatenate)(w333, w329) -> (w334:string[])
        }
      }
      n164 = property on="String" class="Str"("Value"=w325) -> ()  [unwired: 2 in, 2 out]
      n165 = property on="Array" class="Arr (strict)"("Value"=w323) -> ()  [unwired: 2 in, 2 out]
    }
    frame #16 {
      # "check if current on additional Keithley 2400 (addr. 14) is measured"
      n166 = property on="Array" class="Arr (strict)"() -> ("Value"=w338:string[])  [unwired: 2 in, 2 out]
      n167 = property on="String" class="Str"() -> ("Value"=w340:string)  [unwired: 2 in, 2 out]
      n168 = case shown="False" "Current (Ik3)" {
        tunnel: [w342 w346] -> w339
        tunnel: w340 -> [w342 w345]
        tunnel: w338 -> [w341 w347]
        tunnel: [w341 w348] -> w337
        frame False {
          # "no , we aren't measuring current\non Keithley 2400 (addr. 14)"
        }
        frame True {
          w343 = "Ik3"
          # "yes , we are measuring current \non Keithley 2400 (addr. 14)"
          n169 = GPIB Clear(3:"14") -> ()  [unwired: 1 in, 2 out]
          n170 = Concatenate Strings(w345, w343, "\t") -> (w346:string)
          n171 = Build Array (concatenate)(w347, w343) -> (w348:string[])
        }
      }
      n172 = property on="String" class="Str"("Value"=w339) -> ()  [unwired: 2 in, 2 out]
      n173 = property on="Array" class="Arr (strict)"("Value"=w337) -> ()  [unwired: 2 in, 2 out]
    }
    frame #17 {
      # "check if 1st channel of nanovoltmeter Keithley 2182 (addr. 15) is measured"
      n174 = property on="Array" class="Arr (strict)"() -> ("Value"=w352:string[])  [unwired: 2 in, 2 out]
      n175 = property on="String" class="Str"() -> ("Value"=w354:string)  [unwired: 2 in, 2 out]
      n176 = case shown="True" "Channel 1 (Vnano1)" {
        tunnel: [w356 w361] -> w353
        tunnel: w354 -> [w356 w360]
        tunnel: w352 -> [w355 w362]
        tunnel: [w355 w363] -> w351
        frame False {
          # "no , we are not measuring 1st channel\non Keithley 2182 (addr. 15)"
        }
        frame True {
          w358 = "Vnano1"
          # "yes , we are measuring 1st channel\non Keithley 2182 (addr. 15)"
          n177 = GPIB Clear(3:"15") -> ()  [unwired: 1 in, 2 out]
          n178 = Concatenate Strings(w360, w358, "\t") -> (w361:string)
          n179 = Build Array (concatenate)(w362, w358) -> (w363:string[])
        }
      }
      n180 = property on="String" class="Str"("Value"=w353) -> ()  [unwired: 2 in, 2 out]
      n181 = property on="Array" class="Arr (strict)"("Value"=w351) -> ()  [unwired: 2 in, 2 out]
    }
    frame #18 {
      # "check if 2nd channel of nanovoltmeter Keithley 2182 (addr. 15) is measured"
      n182 = property on="Array" class="Arr (strict)"() -> ("Value"=w366:string[])  [unwired: 2 in, 2 out]
      n183 = property on="String" class="Str"() -> ("Value"=w368:string)  [unwired: 2 in, 2 out]
      n184 = case shown="False" "Channel 2 (Vnano1b)" {
        tunnel: [w370 w374] -> w367
        tunnel: w368 -> [w370 w373]
        tunnel: w366 -> [w369 w375]
        tunnel: [w369 w376] -> w365
        frame False {
          # "no , we are not measuring 2nd channel\non Keithley 2182 (addr. 15)"
        }
        frame True {
          w371 = "Vnano1b"
          # "yes , we are measuring 2nd channel\non Keithley 2182 (addr. 15)"
          n185 = GPIB Clear(3:"15") -> ()  [unwired: 1 in, 2 out]
          n186 = Concatenate Strings(w373, w371, "\t") -> (w374:string)
          n187 = Build Array (concatenate)(w375, w371) -> (w376:string[])
        }
      }
      n188 = property on="String" class="Str"("Value"=w367) -> ()  [unwired: 2 in, 2 out]
      n189 = property on="Array" class="Arr (strict)"("Value"=w365) -> ()  [unwired: 2 in, 2 out]
    }
    frame #19 {
      # "check if 1st channel of nanovoltmeter Keithley 2182 (addr. 16) is measured"
      n190 = property on="Array" class="Arr (strict)"() -> ("Value"=w380:string[])  [unwired: 2 in, 2 out]
      n191 = property on="String" class="Str"() -> ("Value"=w382:string)  [unwired: 2 in, 2 out]
      n192 = case shown="True" "Channel 1 (Vnano2)" {
        tunnel: [w384 w389] -> w381
        tunnel: w382 -> [w384 w388]
        tunnel: w380 -> [w383 w390]
        tunnel: [w383 w391] -> w379
        frame False {
          # "no , we are not measuring 1st channel\non Keithley 2182 (addr. 16)"
        }
        frame True {
          w386 = "Vnano2"
          # "yes , we are measuring 1st channel\non Keithley 2182 (addr. 16)"
          n193 = GPIB Clear(3:"16") -> ()  [unwired: 1 in, 2 out]
          n194 = Concatenate Strings(w388, w386, "\t") -> (w389:string)
          n195 = Build Array (concatenate)(w390, w386) -> (w391:string[])
        }
      }
      n196 = property on="String" class="Str"("Value"=w381) -> ()  [unwired: 2 in, 2 out]
      n197 = property on="Array" class="Arr (strict)"("Value"=w379) -> ()  [unwired: 2 in, 2 out]
    }
    frame #20 {
      # "check if 2nd channel of nanovoltmeter Keithley 2182 (addr. 16) is measured"
      n198 = property on="Array" class="Arr (strict)"() -> ("Value"=w394:string[])  [unwired: 2 in, 2 out]
      n199 = property on="String" class="Str"() -> ("Value"=w396:string)  [unwired: 2 in, 2 out]
      n200 = case shown="False" "Channel 2 (Vnano2b)" {
        tunnel: [w398 w402] -> w395
        tunnel: w396 -> [w398 w401]
        tunnel: w394 -> [w397 w403]
        tunnel: [w397 w404] -> w393
        frame False {
          # "no , we are not measuring 2nd channel\non Keithley 2182 (addr. 16)"
        }
        frame True {
          w399 = "Vnano2b"
          # "yes , we are measuring 2nd channel\non Keithley 2182 (addr. 16)"
          n201 = GPIB Clear(3:"16") -> ()  [unwired: 1 in, 2 out]
          n202 = Concatenate Strings(w401, w399, "\t") -> (w402:string)
          n203 = Build Array (concatenate)(w403, w399) -> (w404:string[])
        }
      }
      n204 = property on="String" class="Str"("Value"=w395) -> ()  [unwired: 2 in, 2 out]
      n205 = property on="Array" class="Arr (strict)"("Value"=w393) -> ()  [unwired: 2 in, 2 out]
    }
    frame #21 {
      # "check if 1st channel of nanovoltmeter Keithley 2182 (addr. 17) is measured"
      n206 = property on="Array" class="Arr (strict)"() -> ("Value"=w408:string[])  [unwired: 2 in, 2 out]
      n207 = property on="String" class="Str"() -> ("Value"=w410:string)  [unwired: 2 in, 2 out]
      n208 = case shown="False" "Channel 1 (Vnano3)" {
        tunnel: [w412 w416] -> w409
        tunnel: w410 -> [w412 w415]
        tunnel: w408 -> [w411 w417]
        tunnel: [w411 w418] -> w407
        frame False {
          # "no , we are not measuring 1st channel\non Keithley 2182 (addr. 17)"
        }
        frame True {
          w413 = "Vnano3"
          # "yes , we are measuring 1st channel\non Keithley 2182 (addr. 17)"
          n209 = GPIB Clear(3:"17") -> ()  [unwired: 1 in, 2 out]
          n210 = Concatenate Strings(w415, w413, "\t") -> (w416:string)
          n211 = Build Array (concatenate)(w417, w413) -> (w418:string[])
        }
      }
      n212 = property on="String" class="Str"("Value"=w409) -> ()  [unwired: 2 in, 2 out]
      n213 = property on="Array" class="Arr (strict)"("Value"=w407) -> ()  [unwired: 2 in, 2 out]
    }
    frame #22 {
      # "check if 2nd channel of nanovoltmeter Keithley 2182 (addr. 16) is measured"
      n214 = property on="Array" class="Arr (strict)"() -> ("Value"=w422:string[])  [unwired: 2 in, 2 out]
      n215 = property on="String" class="Str"() -> ("Value"=w424:string)  [unwired: 2 in, 2 out]
      n216 = case shown="False" "Channel 2 (Vnano3b)" {
        tunnel: [w426 w430] -> w423
        tunnel: w424 -> [w426 w429]
        tunnel: w422 -> [w425 w431]
        tunnel: [w425 w432] -> w421
        frame False {
          # "no , we are not measuring 2nd channel\non Keithley 2182 (addr. 17)"
        }
        frame True {
          w427 = "Vnano3b"
          # "yes , we are measuring 2nd channel\non Keithley 2182 (addr. 17)"
          n217 = GPIB Clear(3:"17") -> ()  [unwired: 1 in, 2 out]
          n218 = Concatenate Strings(w429, w427, "\t") -> (w430:string)
          n219 = Build Array (concatenate)(w431, w427) -> (w432:string[])
        }
      }
      n220 = property on="String" class="Str"("Value"=w423) -> ()  [unwired: 2 in, 2 out]
      n221 = property on="Array" class="Arr (strict)"("Value"=w421) -> ()  [unwired: 2 in, 2 out]
    }
    frame #23 {
      # "check if 1st thermometer on Oxford ITC (address 24) is measured"
      n222 = property on="Array" class="Arr (strict)"() -> ("Value"=w436:string[])  [unwired: 2 in, 2 out]
      n223 = property on="String" class="Str"() -> ("Value"=w438:string)  [unwired: 2 in, 2 out]
      n224 = case shown="True" "Thermometer 1 (T1)" {
        tunnel: [w440 w444] -> w437
        tunnel: w438 -> [w440 w443]
        tunnel: w436 -> [w439 w445]
        tunnel: [w439 w446] -> w435
        frame False {
          # "no, we are not measuring temperature\non thermometer 1 (addr. 24)"
        }
        frame True {
          w441 = "T1"
          # "yes, we are measuring temperature,\nthermometer 1 (addr. 24)"
          n225 = GPIB Clear(3:"24") -> ()  [unwired: 1 in, 2 out]
          n226 = Concatenate Strings(w443, w441, "\t") -> (w444:string)
          n227 = Build Array (concatenate)(w445, w441) -> (w446:string[])
        }
      }
      n228 = property on="String" class="Str"("Value"=w437) -> ()  [unwired: 2 in, 2 out]
      n229 = property on="Array" class="Arr (strict)"("Value"=w435) -> ()  [unwired: 2 in, 2 out]
    }
    frame #24 {
      # "check if magnetic field from Oxford IPS 120 (address 25) is measured"
      n230 = property on="Array" class="Arr (strict)"() -> ("Value"=w450:string[])  [unwired: 2 in, 2 out]
      n231 = property on="String" class="Str"() -> ("Value"=w452:string)  [unwired: 2 in, 2 out]
      n232 = case shown="True" "Magnetic Field (B)" {
        tunnel: [w454 w458] -> w451
        tunnel: w452 -> [w454 w457]
        tunnel: w450 -> [w453 w459]
        tunnel: [w453 w460] -> w449
        frame False {
          # "no, we are not measuring magnetic field  (addr. 25)"
        }
        frame True {
          w455 = "B"
          # "yes, we are measuring magnetic field  (addr. 25)"
          n233 = GPIB Clear(3:"25") -> ()  [unwired: 1 in, 2 out]
          n234 = Concatenate Strings(w457, w455, "\t") -> (w458:string)
          n235 = Build Array (concatenate)(w459, w455) -> (w460:string[])
        }
      }
      n236 = property on="String" class="Str"("Value"=w451) -> ()  [unwired: 2 in, 2 out]
      n237 = property on="Array" class="Arr (strict)"("Value"=w449) -> ()  [unwired: 2 in, 2 out]
    }
    frame #25 {
      # "check if capacitance and loss from AH 2500 (address 28) are measured"
      n238 = property on="Array" class="Arr (strict)"() -> ("Value"=w464:string[])  [unwired: 2 in, 2 out]
      n239 = property on="String" class="Str"() -> ("Value"=w466:string)  [unwired: 2 in, 2 out]
      n240 = case shown="False" "Capacitance (C) and Loss (L)" {
        tunnel: [w468 w477] -> w465
        tunnel: w466 -> [w468 w470]
        tunnel: w464 -> [w467 w472]
        tunnel: [w467 w478] -> w463
        frame False {
          # "no, we are not measuring capacitance  (addr. 28)"
        }
        frame True {
          w473 = "C"
          w475 = "L"
          # "yes, we are measuring capacitance and loss  (addr. 28)"
          n241 = GPIB Clear(3:"28") -> ()  [unwired: 1 in, 2 out]
          n242 = Concatenate Strings(w470, w473, "\t") -> (w469:string)
          n243 = Build Array (concatenate)(w472, w473) -> (w471:string[])
          n244 = Concatenate Strings(w469, w475, "\t") -> (w477:string)
          n245 = Build Array (concatenate)(w471, w475) -> (w478:string[])
        }
      }
      n246 = property on="String" class="Str"("Value"=w465) -> ()  [unwired: 2 in, 2 out]
      n247 = property on="Array" class="Arr (strict)"("Value"=w463) -> ()  [unwired: 2 in, 2 out]
    }
  }
  n248 = property on="Array" class="Arr (strict)"(error in=w19) -> (error out=w1:errorcluster, "Value"=w8:string[])  [unwired: 1 in, 1 out]
  n249 = property on="String" class="Str"(error in=w1) -> ("Value"=w4:string)  [unwired: 1 in, 2 out]
  n250 = property on="Commutator" class="Bool (strict)"() -> ("Value"=w7:bool)  [unwired: 2 in, 2 out]
  n251 = case shown="False" w7 {
    tunnel: w8 -> [w482 w500]
    tunnel: [w480 w500] -> w5
    tunnel: w4 -> [w484 w499]
    tunnel: [w483 w499] -> w3
    frame True {
      n252 = Array Size(array=w482) -> (size(s)=w486:i32)
      n253 = Decrement(x=w486) -> (x-1=w485:i32)
      n254 = for {
        N: w485 -> [_]
        shift-right: [w497] -> w481
        shift-left: string[] [] -> [w498]
        shift-right: [w489] -> w483
        shift-left: w484 -> [w490]
        i -> [w494]
        n255 = property on="Array" class="Arr (strict)"() -> ("Value"=w492:string[])  [unwired: 2 in, 2 out]
        n256 = Increment(x=w494) -> (x+1=w493:i32)
        n257 = Index Array(array=w492, index=w493) -> (element=w496:string)
        n258 = Concatenate Strings("c", w496) -> (w488:string)
        n259 = Concatenate Strings(w490, w488, "\t") -> (w489:string)
        n260 = Build Array (concatenate)(w498, w488) -> (w497:string[])
      }
      n261 = Build Array (concatenate)(w482, w481) -> (w480:string[])
      n262 = property on="Array" class="Arr (strict)"("Value"=w480) -> ()  [unwired: 2 in, 2 out]
    }
    frame False {
    }
  }
  n263 = Concatenate Strings(w3, "\r", "\n") -> (w15:string)
  "String" <- w15
  n264 = property on="Ring" class="Ring (strict)"("Strings []"=w5) -> (error out=w2:errorcluster)  [unwired: 2 in, 1 out]
  n265 = property on="Data file:" class="Path"(error in=w2) -> (error out=w14:errorcluster, "Value"=w16:path)  [unwired: 1 in, 1 out]
  n266 = while {
    tunnel: w14 -> [w514]
    shift-right: [w511] -> w13
    shift-left: dbl[][] [] -> [w513]
    shift-right: [w503] -> _
    shift-left: w9 -> [w510]
    tunnel: "points at each Vg" -> [w505]
    tunnel: [w501] -> w11
    stop <- w512 stop-if-true
    w501 = 1e-08
    # "send new Vg value to main Keithley 2400"
    n267 = for {
      N: w505 -> [_]
      tunnel: w514 -> [w530]
      tunnel: [w548] -> w512
      shift-right: [w535] -> w511
      shift-left: w513 -> [w561]
      tunnel: w510 -> [w546]
      tunnel: [w553] -> w503
      w547 = dbl[] []  # Empty array for data
      # "this part appends last\nmeasured point to the \ndata file"
      # "this line is current gate voltage"
      # "First we create an empty array \nfor data and write the first element \ninto it - current gate voltage"
      # "time is measured at the beginning\nand at the end of the cycle to\ncalculate delay time required to\nkeep set sweep rate"
      # "this part calculate resistances and current (if needed) from voltages measured by lock-in amplifiers"
      # "check if the next step doesn't\ngo beyond the target voltage"
      # "calculate difference between target and current Vg"
      # "check if we are at the target voltage yet"
      # "in this part we calculate incriment for Vg"
      n268 = flat-sequence {
        tunnel: w530 -> [w1739]
        tunnel: [w1739] -> w528
        tunnel: [w1741] -> w529
        tunnel: w528 -> [w1741]
        tunnel: [w1740] -> w527
        frame #0 {
          n269 = property on="Deliberate Time delay" class="DigNum (strict)"() -> ("Value"=w1738:i32)  [unwired: 2 in, 2 out]
          n270 = Wait (ms)(milliseconds to wait=w1738) -> ()  [unwired: 1 out]
        }
        frame #1 {
          n271 = Tick Count (ms)() -> (millisecond timer value=w1740:u32)
        }
      }
      n272 = Build Array (concatenate)(w547, w546) -> (w545:dbl[])
      n273 = property on="array for data" class="Arr (strict)"(error in=w529, "Value"=w545) -> (error out=w544:errorcluster)  [unwired: 1 in, 1 out]
      n274 = case shown="False" "Commutator" {
        tunnel: [w588 w1368] -> w562
        tunnel: w544 -> [w589 w1367]
        frame True {
          n275 = stacked-sequence {
            tunnel: w589 -> [w606 w995]
            tunnel: [_ w980] -> w588
            frame #0 {
              n276 = stacked-sequence {
                tunnel: w606 -> [w610 _ _ _ _ _ _ _ _ _ _ _ _ _ _ _ _ _ _ _ _ _ _ _ _ _]
                tunnel: [w610 _ _ _ _ _ _ _ _ _ _ _ _ _ _ _ _ _ _ _ _ _ _ _ _ _] -> w590
                frame #0 {
                  # "check if oscillator on \nlock-in (address 1)\nis to be measured"
                  n277 = property on="Current is:" class="RadioBtnsControl (strict)"() -> ("Value"=w613:T1)  [unwired: 2 in, 2 out]
                  n278 = property on="array for data" class="Arr (strict)"() -> ("Value"=w612:dbl[])  [unwired: 2 in, 2 out]
                  n279 = Equal?(x=w613, y=1) -> (x = y?=w614:bool)
                  n280 = case shown="False" w614 {
                    tunnel: w612 -> [w616 w624]
                    tunnel: [w616 w623] -> w611
                    frame False {
                      # "we are not measuring oscillator from\nlock-in (address 1)"
                    }
                    frame True {
                      w620 = "1"
                      # "we are  measuring oscillator"
                      n281 = GPIB Write(0:w620, 1:"SLVL?") -> (6:w621:errorcluster)  [unwired: 3 in, 1 out]
                      n282 = GPIB Read(0:w620, 1:3200, 3:w621) -> (5:w618:string)  [unwired: 2 in, 2 out]
                      n283 = Fract/Exp String To Number(string=w618) -> (number=w617:dbl)  [unwired: 3 in, 1 out]
                      n284 = Build Array (concatenate)(w624, w617) -> (w623:dbl[])
                    }
                  }
                  n285 = property on="array for data" class="Arr (strict)"("Value"=w611) -> ()  [unwired: 2 in, 2 out]
                }
                frame #1 {
                  # "check if in-phase\nsignal on lock-in \n(address 1) is to\nbe measured"
                  n286 = property on="array for data" class="Arr (strict)"() -> ("Value"=w627:dbl[])  [unwired: 2 in, 2 out]
                  n287 = property on="Addr 1 lock-in" class="Bool (strict)"() -> ("Value"=w625:bool)  [unwired: 2 in, 2 out]
                  n288 = case shown="False" w625 {
                    tunnel: w627 -> [w628 w636]
                    tunnel: [w628 w635] -> w626
                    frame False {
                      # "we are not measuring in phase signal on lock-in (address 1)"
                    }
                    frame True {
                      w633 = "1"
                      # "we are  measuring lock-in (address 1), in phase"
                      n289 = GPIB Write(0:w633, 1:"OUTP?1") -> (6:w634:errorcluster)  [unwired: 3 in, 1 out]
                      n290 = GPIB Read(0:w633, 1:3200, 3:w634) -> (5:w631:string)  [unwired: 2 in, 2 out]
                      n291 = Fract/Exp String To Number(string=w631) -> (number=w630:dbl)  [unwired: 3 in, 1 out]
                      n292 = Build Array (concatenate)(w636, w630) -> (w635:dbl[])
                    }
                  }
                  n293 = property on="array for data" class="Arr (strict)"("Value"=w626) -> ()  [unwired: 2 in, 2 out]
                }
                frame #2 {
                  # "check if out-of-phase\nsignal on lock-in \n(address 1) is to\nbe measured"
                  n294 = property on="Addr 1 lock-in oop" class="Bool (strict)"() -> ("Value"=w637:bool)  [unwired: 2 in, 2 out]
                  n295 = property on="array for data" class="Arr (strict)"() -> ("Value"=w639:dbl[])  [unwired: 2 in, 2 out]
                  n296 = case shown="False" w637 {
                    tunnel: w639 -> [w640 w648]
                    tunnel: [w640 w647] -> w638
                    frame False {
                      # "we are not measuring out-of-phase signal on lock-in (address 1)"
                    }
                    frame True {
                      w645 = "1"
                      # "we are  measuring lock-in (address 1), out-of-phase signal"
                      n297 = GPIB Write(0:w645, 1:"OUTP?2") -> (6:w646:errorcluster)  [unwired: 3 in, 1 out]
                      n298 = GPIB Read(0:w645, 1:3200, 3:w646) -> (5:w643:string)  [unwired: 2 in, 2 out]
                      n299 = Fract/Exp String To Number(string=w643) -> (number=w642:dbl)  [unwired: 3 in, 1 out]
                      n300 = Build Array (concatenate)(w648, w642) -> (w647:dbl[])
                    }
                  }
                  n301 = property on="array for data" class="Arr (strict)"("Value"=w638) -> ()  [unwired: 2 in, 2 out]
                }
                frame #3 {
                  # "check if in-phase\nsignal on lock-in \n(address 2) is to\nbe measured"
                  n302 = property on="Addr 2 lock-in" class="Bool (strict)"() -> ("Value"=w649:bool)  [unwired: 2 in, 2 out]
                  n303 = property on="array for data" class="Arr (strict)"() -> ("Value"=w651:dbl[])  [unwired: 2 in, 2 out]
                  n304 = case shown="False" w649 {
                    tunnel: w651 -> [w652 w660]
                    tunnel: [w652 w659] -> w650
                    frame False {
                      # "we are not measuring in phase signal on lock-in (address 2)"
                    }
                    frame True {
                      w657 = "2"
                      # "we are  measuring lock-in (address 2), in phase"
                      n305 = GPIB Write(0:w657, 1:"OUTP?1") -> (6:w658:errorcluster)  [unwired: 3 in, 1 out]
                      n306 = GPIB Read(0:w657, 1:3200, 3:w658) -> (5:w655:string)  [unwired: 2 in, 2 out]
                      n307 = Fract/Exp String To Number(string=w655) -> (number=w654:dbl)  [unwired: 3 in, 1 out]
                      n308 = Build Array (concatenate)(w660, w654) -> (w659:dbl[])
                    }
                  }
                  n309 = property on="array for data" class="Arr (strict)"("Value"=w650) -> ()  [unwired: 2 in, 2 out]
                }
                frame #4 {
                  # "check if out-of-phase\nsignal on lock-in \n(address 2) is to\nbe measured"
                  n310 = property on="Addr 2 lock-in oop" class="Bool (strict)"() -> ("Value"=w661:bool)  [unwired: 2 in, 2 out]
                  n311 = property on="array for data" class="Arr (strict)"() -> ("Value"=w663:dbl[])  [unwired: 2 in, 2 out]
                  n312 = case shown="False" w661 {
                    tunnel: w663 -> [w664 w672]
                    tunnel: [w664 w671] -> w662
                    tunnel: w661 -> [_ _]
                    frame False {
                      # "we are not measuring out-of-phase signal on lock-in (address 2)"
                    }
                    frame True {
                      w669 = "2"
                      # "we are  measuring lock-in (address 2), out-of-phase"
                      n313 = GPIB Write(0:w669, 1:"OUTP?2") -> (6:w670:errorcluster)  [unwired: 3 in, 1 out]
                      n314 = GPIB Read(0:w669, 1:3200, 3:w670) -> (5:w667:string)  [unwired: 2 in, 2 out]
                      n315 = Fract/Exp String To Number(string=w667) -> (number=w666:dbl)  [unwired: 3 in, 1 out]
                      n316 = Build Array (concatenate)(w672, w666) -> (w671:dbl[])
                    }
                  }
                  n317 = property on="array for data" class="Arr (strict)"("Value"=w662) -> ()  [unwired: 2 in, 2 out]
                }
                frame #5 {
                  # "check if in-phase\nsignal on lock-in \n(address 3) is to\nbe measured"
                  n318 = property on="Addr 3 lock-in" class="Bool (strict)"() -> ("Value"=w673:bool)  [unwired: 2 in, 2 out]
                  n319 = property on="array for data" class="Arr (strict)"() -> ("Value"=w675:dbl[])  [unwired: 2 in, 2 out]
                  n320 = case shown="False" w673 {
                    tunnel: w675 -> [w676 w684]
                    tunnel: [w676 w683] -> w674
                    frame False {
                      # "we are not measuring in phase signal on lock-in (address 3)"
                    }
                    frame True {
                      w681 = "3"
                      # "we are  measuring lock-in (address 3), in phase"
                      n321 = GPIB Write(0:w681, 1:"OUTP?1") -> (6:w682:errorcluster)  [unwired: 3 in, 1 out]
                      n322 = GPIB Read(0:w681, 1:3200, 3:w682) -> (5:w679:string)  [unwired: 2 in, 2 out]
                      n323 = Fract/Exp String To Number(string=w679) -> (number=w678:dbl)  [unwired: 3 in, 1 out]
                      n324 = Build Array (concatenate)(w684, w678) -> (w683:dbl[])
                    }
                  }
                  n325 = property on="array for data" class="Arr (strict)"("Value"=w674) -> ()  [unwired: 2 in, 2 out]
                }
                frame #6 {
                  # "check if out-of-phase\nsignal on lock-in \n(address 3) is to\nbe measured"
                  n326 = property on="Addr 3 lock-in oop" class="Bool (strict)"() -> ("Value"=w685:bool)  [unwired: 2 in, 2 out]
                  n327 = property on="array for data" class="Arr (strict)"() -> ("Value"=w687:dbl[])  [unwired: 2 in, 2 out]
                  n328 = case shown="False" w685 {
                    tunnel: w687 -> [w688 w696]
                    tunnel: [w688 w695] -> w686
                    frame False {
                      # "we are not measuring out-of-phase signal on lock-in (address 3)"
                    }
                    frame True {
                      w693 = "3"
                      # "we are  measuring lock-in (address 3), out-of-phase"
                      n329 = GPIB Write(0:w693, 1:"OUTP?2") -> (6:w694:errorcluster)  [unwired: 3 in, 1 out]
                      n330 = GPIB Read(0:w693, 1:3200, 3:w694) -> (5:w691:string)  [unwired: 2 in, 2 out]
                      n331 = Fract/Exp String To Number(string=w691) -> (number=w690:dbl)  [unwired: 3 in, 1 out]
                      n332 = Build Array (concatenate)(w696, w690) -> (w695:dbl[])
                    }
                  }
                  n333 = property on="array for data" class="Arr (strict)"("Value"=w686) -> ()  [unwired: 2 in, 2 out]
                }
                frame #7 {
                  # "check if in-phase\nsignal on lock-in \n(address 4) is to\nbe measured"
                  n334 = property on="Addr 4 lock-in" class="Bool (strict)"() -> ("Value"=w697:bool)  [unwired: 2 in, 2 out]
                  n335 = property on="array for data" class="Arr (strict)"() -> ("Value"=w699:dbl[])  [unwired: 2 in, 2 out]
                  n336 = case shown="False" w697 {
                    tunnel: w699 -> [w700 w708]
                    tunnel: [w700 w707] -> w698
                    frame False {
                      # "we are not measuring in phase signal on lock-in (address 4)"
                    }
                    frame True {
                      w705 = "4"
                      # "we are  measuring lock-in (address 4), in phase"
                      n337 = GPIB Write(0:w705, 1:"OUTP?1") -> (6:w706:errorcluster)  [unwired: 3 in, 1 out]
                      n338 = GPIB Read(0:w705, 1:3200, 3:w706) -> (5:w703:string)  [unwired: 2 in, 2 out]
                      n339 = Fract/Exp String To Number(string=w703) -> (number=w702:dbl)  [unwired: 3 in, 1 out]
                      n340 = Build Array (concatenate)(w708, w702) -> (w707:dbl[])
                    }
                  }
                  n341 = property on="array for data" class="Arr (strict)"("Value"=w698) -> ()  [unwired: 2 in, 2 out]
                }
                frame #8 {
                  # "check if out-of-phase\nsignal on lock-in \n(address 4) is to\nbe measured"
                  n342 = property on="Addr 4 lock-in oop" class="Bool (strict)"() -> ("Value"=w709:bool)  [unwired: 2 in, 2 out]
                  n343 = property on="array for data" class="Arr (strict)"() -> ("Value"=w711:dbl[])  [unwired: 2 in, 2 out]
                  n344 = case shown="False" w709 {
                    tunnel: w711 -> [w712 w720]
                    tunnel: [w712 w719] -> w710
                    frame False {
                      # "we are not measuring out-of-phase signal on lock-in (address 4)"
                    }
                    frame True {
                      w717 = "4"
                      # "we are  measuring lock-in (address 4), out-of-phase"
                      n345 = GPIB Write(0:w717, 1:"OUTP?2") -> (6:w718:errorcluster)  [unwired: 3 in, 1 out]
                      n346 = GPIB Read(0:w717, 1:3200, 3:w718) -> (5:w715:string)  [unwired: 2 in, 2 out]
                      n347 = Fract/Exp String To Number(string=w715) -> (number=w714:dbl)  [unwired: 3 in, 1 out]
                      n348 = Build Array (concatenate)(w720, w714) -> (w719:dbl[])
                    }
                  }
                  n349 = property on="array for data" class="Arr (strict)"("Value"=w710) -> ()  [unwired: 2 in, 2 out]
                }
                frame #9 {
                  # "check if in-phase\nsignal on lock-in \n(address 5) is to\nbe measured"
                  n350 = property on="Addr 5 lock-in" class="Bool (strict)"() -> ("Value"=w721:bool)  [unwired: 2 in, 2 out]
                  n351 = property on="array for data" class="Arr (strict)"() -> ("Value"=w723:dbl[])  [unwired: 2 in, 2 out]
                  n352 = case shown="False" w721 {
                    tunnel: w723 -> [w724 w732]
                    tunnel: [w724 w731] -> w722
                    frame False {
                      # "we are not measuring in phase signal on lock-in (address 5)"
                    }
                    frame True {
                      w729 = "5"
                      # "we are  measuring lock-in (address 5), in phase"
                      n353 = GPIB Write(0:w729, 1:"OUTP?1") -> (6:w730:errorcluster)  [unwired: 3 in, 1 out]
                      n354 = GPIB Read(0:w729, 1:3200, 3:w730) -> (5:w727:string)  [unwired: 2 in, 2 out]
                      n355 = Fract/Exp String To Number(string=w727) -> (number=w726:dbl)  [unwired: 3 in, 1 out]
                      n356 = Build Array (concatenate)(w732, w726) -> (w731:dbl[])
                    }
                  }
                  n357 = property on="array for data" class="Arr (strict)"("Value"=w722) -> ()  [unwired: 2 in, 2 out]
                }
                frame #10 {
                  # "check if out-of-phase\nsignal on lock-in \n(address 5) is to\nbe measured"
                  n358 = property on="Addr 5 lock-in oop" class="Bool (strict)"() -> ("Value"=w733:bool)  [unwired: 2 in, 2 out]
                  n359 = property on="array for data" class="Arr (strict)"() -> ("Value"=w735:dbl[])  [unwired: 2 in, 2 out]
                  n360 = case shown="False" w733 {
                    tunnel: w735 -> [w736 w744]
                    tunnel: [w736 w743] -> w734
                    frame False {
                      # "we are not measuring out-of-phase signal on lock-in (address 5)"
                    }
                    frame True {
                      w741 = "5"
                      # "we are  measuring lock-in (address 5), out-of-phase"
                      n361 = GPIB Write(0:w741, 1:"OUTP?2") -> (6:w742:errorcluster)  [unwired: 3 in, 1 out]
                      n362 = GPIB Read(0:w741, 1:3200, 3:w742) -> (5:w739:string)  [unwired: 2 in, 2 out]
                      n363 = Fract/Exp String To Number(string=w739) -> (number=w738:dbl)  [unwired: 3 in, 1 out]
                      n364 = Build Array (concatenate)(w744, w738) -> (w743:dbl[])
                    }
                  }
                  n365 = property on="array for data" class="Arr (strict)"("Value"=w734) -> ()  [unwired: 2 in, 2 out]
                }
                frame #11 {
                  # "check if voltage on \nmain Keithley 2400 \n(addr. 12) is to\nbe measured"
                  n366 = property on="Voltage (Vk1)" class="Bool (strict)"() -> ("Value"=w745:bool)  [unwired: 2 in, 2 out]
                  n367 = property on="array for data" class="Arr (strict)"() -> ("Value"=w747:dbl[])  [unwired: 2 in, 2 out]
                  n368 = case shown="False" w745 {
                    tunnel: w747 -> [w748 w758]
                    tunnel: [w748 w757] -> w746
                    frame False {
                      # "we aren't measuring voltage \non main Keithley 2400 (addr. 12)"
                    }
                    frame True {
                      w755 = "12"
                      # "we are measuring voltage \non main Keithley 2400 (addr. 12)"
                      n369 = GPIB Write(0:w755, 1:":READ?") -> (6:w756:errorcluster)  [unwired: 3 in, 1 out]
                      n370 = GPIB Read(0:w755, 1:3200, 3:w756) -> (5:w751:string)  [unwired: 2 in, 2 out]
                      n371 = String Subset(string=w751, length (rest)=13) -> (substring=w750:string)  [unwired: 1 in]
                      n372 = Fract/Exp String To Number(string=w750) -> (number=w753:dbl)  [unwired: 3 in, 1 out]
                      n373 = Build Array (concatenate)(w758, w753) -> (w757:dbl[])
                    }
                  }
                  n374 = property on="array for data" class="Arr (strict)"("Value"=w746) -> ()  [unwired: 2 in, 2 out]
                }
                frame #12 {
                  # "check if  current on \nmain Keithley 2400 \n(addr. 12) is to\nbe measured"
                  n375 = property on="Current (Ik1)" class="Bool (strict)"() -> ("Value"=w759:bool)  [unwired: 2 in, 2 out]
                  n376 = property on="array for data" class="Arr (strict)"() -> ("Value"=w761:dbl[])  [unwired: 2 in, 2 out]
                  n377 = case shown="True" w759 {
                    tunnel: w761 -> [w762 w773]
                    tunnel: [w762 w772] -> w760
                    frame False {
                      # "we aren't measuring current \non main Keithley 2400 (addr. 12)"
                    }
                    frame True {
                      w770 = "12"
                      # "we are measuring current\non main Keithley 2400 (addr. 12)"
                      n378 = GPIB Write(0:w770, 1:":READ?") -> (6:w771:errorcluster)  [unwired: 3 in, 1 out]
                      n379 = GPIB Read(0:w770, 1:3200, 3:w771) -> (5:w766:string)  [unwired: 2 in, 2 out]
                      n380 = String Subset(string=w766, offset (0)=14, length (rest)=13) -> (substring=w765:string)
                      n381 = Fract/Exp String To Number(string=w765) -> (number=w768:dbl)  [unwired: 3 in, 1 out]
                      n382 = Build Array (concatenate)(w773, w768) -> (w772:dbl[])
                    }
                  }
                  n383 = property on="array for data" class="Arr (strict)"("Value"=w760) -> ()  [unwired: 2 in, 2 out]
                }
                frame #13 {
                  # "check if voltage on \nadd. Keithley 2400 \n(addr. 13) is to\nbe measured"
                  n384 = property on="Voltage (Vk2)" class="Bool (strict)"() -> ("Value"=w774:bool)  [unwired: 2 in, 2 out]
                  n385 = property on="array for data" class="Arr (strict)"() -> ("Value"=w776:dbl[])  [unwired: 2 in, 2 out]
                  n386 = case shown="True" w774 {
                    tunnel: w776 -> [w777 w787]
                    tunnel: [w777 w786] -> w775
                    frame False {
                      # "we aren't measuring voltage \non additional Keithley 2400 (addr. 13)"
                    }
                    frame True {
                      w784 = "13"
                      # "we are measuring voltage \non additional Keithley 2400 (addr. 13)"
                      n387 = GPIB Write(0:w784, 1:":READ?") -> (6:w785:errorcluster)  [unwired: 3 in, 1 out]
                      n388 = GPIB Read(0:w784, 1:3200, 3:w785) -> (5:w780:string)  [unwired: 2 in, 2 out]
                      n389 = String Subset(string=w780, length (rest)=13) -> (substring=w779:string)  [unwired: 1 in]
                      n390 = Fract/Exp String To Number(string=w779) -> (number=w782:dbl)  [unwired: 3 in, 1 out]
                      n391 = Build Array (concatenate)(w787, w782) -> (w786:dbl[])
                    }
                  }
                  n392 = property on="array for data" class="Arr (strict)"("Value"=w775) -> ()  [unwired: 2 in, 2 out]
                }
                frame #14 {
                  # "check if  current on \nadd. Keithley 2400 \n(addr. 13) is to\nbe measured"
                  n393 = property on="Current (Ik2)" class="Bool (strict)"() -> ("Value"=w788:bool)  [unwired: 2 in, 2 out]
                  n394 = property on="array for data" class="Arr (strict)"() -> ("Value"=w790:dbl[])  [unwired: 2 in, 2 out]
                  n395 = case shown="True" w788 {
                    tunnel: w790 -> [w791 w802]
                    tunnel: [w791 w801] -> w789
                    frame False {
                      # "we aren't measuring current \non additional Keithley 2400 (addr. 13)"
                    }
                    frame True {
                      w799 = "13"
                      # "we are measuring current\non additional Keithley 2400 (addr. 13)"
                      n396 = GPIB Write(0:w799, 1:":READ?") -> (6:w800:errorcluster)  [unwired: 3 in, 1 out]
                      n397 = GPIB Read(0:w799, 1:3200, 3:w800) -> (5:w795:string)  [unwired: 2 in, 2 out]
                      n398 = String Subset(string=w795, offset (0)=14, length (rest)=13) -> (substring=w794:string)
                      n399 = Fract/Exp String To Number(string=w794) -> (number=w797:dbl)  [unwired: 3 in, 1 out]
                      n400 = Build Array (concatenate)(w802, w797) -> (w801:dbl[])
                    }
                  }
                  n401 = property on="array for data" class="Arr (strict)"("Value"=w789) -> ()  [unwired: 2 in, 2 out]
                }
                frame #15 {
                  # "check if voltage on \nadd. Keithley 2400 \n(addr. 14) is to\nbe measured"
                  n402 = property on="Voltage (Vk3)" class="Bool (strict)"() -> ("Value"=w803:bool)  [unwired: 2 in, 2 out]
                  n403 = property on="array for data" class="Arr (strict)"() -> ("Value"=w805:dbl[])  [unwired: 2 in, 2 out]
                  n404 = case shown="True" w803 {
                    tunnel: w805 -> [w806 w816]
                    tunnel: [w806 w815] -> w804
                    frame False {
                      # "we aren't measuring voltage \non additional Keithley 2400 (addr. 14)"
                    }
                    frame True {
                      w813 = "14"
                      # "we are measuring voltage \non additional Keithley 2400 (addr. 14)"
                      n405 = GPIB Write(0:w813, 1:":READ?") -> (6:w814:errorcluster)  [unwired: 3 in, 1 out]
                      n406 = GPIB Read(0:w813, 1:3200, 3:w814) -> (5:w809:string)  [unwired: 2 in, 2 out]
                      n407 = String Subset(string=w809, length (rest)=13) -> (substring=w808:string)  [unwired: 1 in]
                      n408 = Fract/Exp String To Number(string=w808) -> (number=w811:dbl)  [unwired: 3 in, 1 out]
                      n409 = Build Array (concatenate)(w816, w811) -> (w815:dbl[])
                    }
                  }
                  n410 = property on="array for data" class="Arr (strict)"("Value"=w804) -> ()  [unwired: 2 in, 2 out]
                }
                frame #16 {
                  # "check if  current on \nadd. Keithley 2400 \n(addr. 14) is to\nbe measured"
                  n411 = property on="Current (Ik3)" class="Bool (strict)"() -> ("Value"=w817:bool)  [unwired: 2 in, 2 out]
                  n412 = property on="array for data" class="Arr (strict)"() -> ("Value"=w819:dbl[])  [unwired: 2 in, 2 out]
                  n413 = case shown="True" w817 {
                    tunnel: w819 -> [w820 w831]
                    tunnel: [w820 w830] -> w818
                    frame False {
                      # "we aren't measuring current \non additional Keithley 2400 (addr. 14)"
                    }
                    frame True {
                      w828 = "14"
                      # "we are measuring current\non additional Keithley 2400 (addr. 14)"
                      n414 = GPIB Write(0:w828, 1:":READ?") -> (6:w829:errorcluster)  [unwired: 3 in, 1 out]
                      n415 = GPIB Read(0:w828, 1:3200, 3:w829) -> (5:w824:string)  [unwired: 2 in, 2 out]
                      n416 = String Subset(string=w824, offset (0)=14, length (rest)=13) -> (substring=w823:string)
                      n417 = Fract/Exp String To Number(string=w823) -> (number=w826:dbl)  [unwired: 3 in, 1 out]
                      n418 = Build Array (concatenate)(w831, w826) -> (w830:dbl[])
                    }
                  }
                  n419 = property on="array for data" class="Arr (strict)"("Value"=w818) -> ()  [unwired: 2 in, 2 out]
                }
                frame #17 {
                  # "check if 1st channel\non Keithley 2182 \n(addr. 15) is to\nbe measured"
                  n420 = property on="Channel 1 (Vnano1)" class="Bool (strict)"() -> ("Value"=w832:bool)  [unwired: 2 in, 2 out]
                  n421 = property on="array for data" class="Arr (strict)"() -> ("Value"=w834:dbl[])  [unwired: 2 in, 2 out]
                  n422 = case shown="True" w832 {
                    tunnel: w834 -> [w835 w843]
                    tunnel: [w835 w842] -> w833
                    frame False {
                      # "we are not measuring 1st channel\non Keithley 2182 (addr. 15)"
                    }
                    frame True {
                      w840 = "15"
                      # "we are measuring 1st channel\non Keithley 2182 (addr. 15)"
                      n423 = GPIB Write(0:w840, 1:":SENSe:DATA:FRES?") -> (6:w841:errorcluster)  [unwired: 3 in, 1 out]
                      n424 = GPIB Read(0:w840, 1:200, 3:w841) -> (5:w836:string)  [unwired: 2 in, 2 out]
                      n425 = Fract/Exp String To Number(string=w836) -> (number=w838:dbl)  [unwired: 3 in, 1 out]
                      n426 = Build Array (concatenate)(w843, w838) -> (w842:dbl[])
                    }
                  }
                  n427 = property on="array for data" class="Arr (strict)"("Value"=w833) -> ()  [unwired: 2 in, 2 out]
                }
                frame #18 {
                  # "check if 2nd channel\non Keithley 2182 \n(addr. 15) is to\nbe measured"
                  n428 = property on="Channel 2 (Vnano1b)" class="Bool (strict)"() -> ("Value"=w844:bool)  [unwired: 2 in, 2 out]
                  n429 = property on="array for data" class="Arr (strict)"() -> ("Value"=w846:dbl[])  [unwired: 2 in, 2 out]
                  n430 = case shown="False" w844 {
                    tunnel: w846 -> [w847 w859]
                    tunnel: [w847 w858] -> w845
                    frame False {
                      # "we are not measuring 1st channel\non Keithley 2182 (addr. 15)"
                    }
                    frame True {
                      w850 = "15"
                      # "switching to channel 2 and then\nback to channel 1"
                      # "we are measuring 2nd channel\non Keithley 2182 (addr. 15)"
                      n431 = GPIB Write(0:w850, 1:":SENSe:CHAN 2") -> (6:w851:errorcluster)  [unwired: 3 in, 1 out]
                      n432 = GPIB Write(0:w850, 1:":SENSe:DATA:FRES?", 3:w851) -> (6:w857:errorcluster)  [unwired: 2 in, 1 out]
                      n433 = GPIB Read(0:w850, 1:200, 3:w857) -> (5:w853:string, 7:w849:errorcluster)  [unwired: 2 in, 1 out]
                      n434 = GPIB Write(0:w850, 1:":SENSe:CHAN 1", 3:w849) -> ()  [unwired: 2 in, 2 out]
                      n435 = Fract/Exp String To Number(string=w853) -> (number=w855:dbl)  [unwired: 3 in, 1 out]
                      n436 = Build Array (concatenate)(w859, w855) -> (w858:dbl[])
                    }
                  }
                  n437 = property on="array for data" class="Arr (strict)"("Value"=w845) -> ()  [unwired: 2 in, 2 out]
                }
                frame #19 {
                  # "check if 1st channel\non Keithley 2182 \n(addr. 16) is to\nbe measured"
                  n438 = property on="Channel 1 (Vnano2)" class="Bool (strict)"() -> ("Value"=w860:bool)  [unwired: 2 in, 2 out]
                  n439 = property on="array for data" class="Arr (strict)"() -> ("Value"=w862:dbl[])  [unwired: 2 in, 2 out]
                  n440 = case shown="True" w860 {
                    tunnel: w862 -> [w863 w871]
                    tunnel: [w863 w870] -> w861
                    frame False {
                      # "we are not measuring 1st channel\non Keithley 2182 (addr. 16)"
                    }
                    frame True {
                      w868 = "16"
                      # "we are measuring 1st channel\non Keithley 2182 (addr. 16)"
                      n441 = GPIB Write(0:w868, 1:":SENSe:DATA:FRES?") -> (6:w869:errorcluster)  [unwired: 3 in, 1 out]
                      n442 = GPIB Read(0:w868, 1:200, 3:w869) -> (5:w864:string)  [unwired: 2 in, 2 out]
                      n443 = Fract/Exp String To Number(string=w864) -> (number=w866:dbl)  [unwired: 3 in, 1 out]
                      n444 = Build Array (concatenate)(w871, w866) -> (w870:dbl[])
                    }
                  }
                  n445 = property on="array for data" class="Arr (strict)"("Value"=w861) -> ()  [unwired: 2 in, 2 out]
                }
                frame #20 {
                  # "check if 2nd channel\non Keithley 2182 \n(addr. 16) is to\nbe measured"
                  n446 = property on="Channel 2 (Vnano2b)" class="Bool (strict)"() -> ("Value"=w872:bool)  [unwired: 2 in, 2 out]
                  n447 = property on="array for data" class="Arr (strict)"() -> ("Value"=w874:dbl[])  [unwired: 2 in, 2 out]
                  n448 = case shown="False" w872 {
                    tunnel: w874 -> [w875 w887]
                    tunnel: [w875 w886] -> w873
                    frame False {
                      # "we are not measuring 1st channel\non Keithley 2182 (addr. 16)"
                    }
                    frame True {
                      w878 = "16"
                      # "switching to channel 2 and then\nback to channel 1"
                      # "we are measuring 2nd channel\non Keithley 2182 (addr. 16)"
                      n449 = GPIB Write(0:w878, 1:":SENSe:CHAN 2") -> (6:w879:errorcluster)  [unwired: 3 in, 1 out]
                      n450 = GPIB Write(0:w878, 1:":SENSe:DATA:FRES?", 3:w879) -> (6:w885:errorcluster)  [unwired: 2 in, 1 out]
                      n451 = GPIB Read(0:w878, 1:200, 3:w885) -> (5:w881:string, 7:w877:errorcluster)  [unwired: 2 in, 1 out]
                      n452 = GPIB Write(0:w878, 1:":SENSe:CHAN 1", 3:w877) -> ()  [unwired: 2 in, 2 out]
                      n453 = Fract/Exp String To Number(string=w881) -> (number=w883:dbl)  [unwired: 3 in, 1 out]
                      n454 = Build Array (concatenate)(w887, w883) -> (w886:dbl[])
                    }
                  }
                  n455 = property on="array for data" class="Arr (strict)"("Value"=w873) -> ()  [unwired: 2 in, 2 out]
                }
                frame #21 {
                  # "check if 1st channel\non Keithley 2182 \n(addr. 17) is to\nbe measured"
                  n456 = property on="Channel 1 (Vnano3)" class="Bool (strict)"() -> ("Value"=w888:bool)  [unwired: 2 in, 2 out]
                  n457 = property on="array for data" class="Arr (strict)"() -> ("Value"=w890:dbl[])  [unwired: 2 in, 2 out]
                  n458 = case shown="True" w888 {
                    tunnel: w890 -> [w891 w899]
                    tunnel: [w891 w898] -> w889
                    frame False {
                      # "we are not measuring 1st channel\non Keithley 2182 (addr. 17)"
                    }
                    frame True {
                      w896 = "17"
                      # "we are measuring 1st channel\non Keithley 2182 (addr. 17)"
                      n459 = GPIB Write(0:w896, 1:":SENSe:DATA:FRES?") -> (6:w897:errorcluster)  [unwired: 3 in, 1 out]
                      n460 = GPIB Read(0:w896, 1:200, 3:w897) -> (5:w892:string)  [unwired: 2 in, 2 out]
                      n461 = Fract/Exp String To Number(string=w892) -> (number=w894:dbl)  [unwired: 3 in, 1 out]
                      n462 = Build Array (concatenate)(w899, w894) -> (w898:dbl[])
                    }
                  }
                  n463 = property on="array for data" class="Arr (strict)"("Value"=w889) -> ()  [unwired: 2 in, 2 out]
                }
                frame #22 {
                  # "check if 2nd channel\non Keithley 2182 \n(addr. 17) is to\nbe measured"
                  n464 = property on="Channel 2 (Vnano3b)" class="Bool (strict)"() -> ("Value"=w900:bool)  [unwired: 2 in, 2 out]
                  n465 = property on="array for data" class="Arr (strict)"() -> ("Value"=w902:dbl[])  [unwired: 2 in, 2 out]
                  n466 = case shown="False" w900 {
                    tunnel: w902 -> [w903 w915]
                    tunnel: [w903 w914] -> w901
                    frame False {
                      # "we are not measuring 1st channel\non Keithley 2182 (addr. 17)"
                    }
                    frame True {
                      w906 = "17"
                      # "switching to channel 2 and then\nback to channel 1"
                      # "we are measuring 2nd channel\non Keithley 2182 (addr. 17)"
                      n467 = GPIB Write(0:w906, 1:":SENSe:CHAN 2") -> (6:w907:errorcluster)  [unwired: 3 in, 1 out]
                      n468 = GPIB Write(0:w906, 1:":SENSe:DATA:FRES?", 3:w907) -> (6:w913:errorcluster)  [unwired: 2 in, 1 out]
                      n469 = GPIB Read(0:w906, 1:200, 3:w913) -> (5:w909:string, 7:w905:errorcluster)  [unwired: 2 in, 1 out]
                      n470 = GPIB Write(0:w906, 1:":SENSe:CHAN 1", 3:w905) -> ()  [unwired: 2 in, 2 out]
                      n471 = Fract/Exp String To Number(string=w909) -> (number=w911:dbl)  [unwired: 3 in, 1 out]
                      n472 = Build Array (concatenate)(w915, w911) -> (w914:dbl[])
                    }
                  }
                  n473 = property on="array for data" class="Arr (strict)"("Value"=w901) -> ()  [unwired: 2 in, 2 out]
                }
                frame #23 {
                  # "check if 1st \nthermometer on \nOxford ITC \n(address 24) \nis measured"
                  n474 = property on="Thermometer 1 (T1)" class="Bool (strict)"() -> ("Value"=w916:bool)  [unwired: 2 in, 2 out]
                  n475 = property on="array for data" class="Arr (strict)"() -> ("Value"=w918:dbl[])  [unwired: 2 in, 2 out]
                  n476 = case shown="True" w916 {
                    tunnel: w918 -> [w919 w928]
                    tunnel: [w919 w927] -> w917
                    frame False {
                      # "we are not measuring temperature on\nthermometer 1 (addr. 24)"
                    }
                    frame True {
                      w920 = 1
                      w925 = "24"
                      # "we are measuring temperature,\nthermometer 1 (addr. 24)"
                      n477 = GPIB Write(0:w925, 1:"R 1", 2:w920) -> (6:w926:errorcluster)  [unwired: 2 in, 1 out]
                      n478 = GPIB Read(0:w925, 1:200, 2:w920, 3:w926) -> (5:w921:string)  [unwired: 1 in, 2 out]
                      n479 = Fract/Exp String To Number(string=w921, offset=w920) -> (number=w923:dbl)  [unwired: 2 in, 1 out]
                      n480 = Build Array (concatenate)(w928, w923) -> (w927:dbl[])
                    }
                  }
                  n481 = property on="array for data" class="Arr (strict)"("Value"=w917) -> ()  [unwired: 2 in, 2 out]
                }
                frame #24 {
                  # "check if 1st \nthermometer on \nOxford ITC \n(address 24) \nis measured"
                  n482 = property on="Magnetic Field (B)" class="Bool (strict)"() -> ("Value"=w929:bool)  [unwired: 2 in, 2 out]
                  n483 = property on="array for data" class="Arr (strict)"() -> ("Value"=w931:dbl[])  [unwired: 2 in, 2 out]
                  n484 = case shown="True" w929 {
                    tunnel: w931 -> [w932 w941]
                    tunnel: [w932 w940] -> w930
                    frame False {
                      # "we are not measuringmagnetic field (addr. 25)"
                    }
                    frame True {
                      w933 = 1
                      w938 = "25"
                      # "we are measuring magnetic field  (addr. 25)"
                      n485 = GPIB Write(0:w938, 1:"R 7", 2:w933) -> (6:w939:errorcluster)  [unwired: 2 in, 1 out]
                      n486 = GPIB Read(0:w938, 1:200, 2:w933, 3:w939) -> (5:w934:string)  [unwired: 1 in, 2 out]
                      n487 = Fract/Exp String To Number(string=w934, offset=w933) -> (number=w936:dbl)  [unwired: 2 in, 1 out]
                      n488 = Build Array (concatenate)(w941, w936) -> (w940:dbl[])
                    }
                  }
                  n489 = property on="array for data" class="Arr (strict)"("Value"=w930) -> ()  [unwired: 2 in, 2 out]
                }
                frame #25 {
                  # "check if capacitance\nand loss (address 28)\nare measured"
                  n490 = property on="Capacitance (C) and Loss (L)" class="Bool (strict)"() -> ("Value"=w942:bool)  [unwired: 2 in, 2 out]
                  n491 = property on="array for data" class="Arr (strict)"() -> ("Value"=w944:dbl[])  [unwired: 2 in, 2 out]
                  n492 = case shown="False" w942 {
                    tunnel: w944 -> [w945 w951]
                    tunnel: [w945 w947] -> w943
                    frame False {
                      # "we are not measuringmagnetic capacitance (addr. 28)"
                    }
                    frame True {
                      # "we are measuring capacitance and loss  (addr. 28)"
                      n493 = stacked-sequence {
                        seq-local: [w953 _ _] -> [_ _ w976]
                        tunnel: [_ _ w970] -> w946
                        tunnel: [_ _ w971] -> w949
                        tunnel: "28" ("data") -> [w952 w956 w965]
                        frame #0 {
                          n494 = GPIB Write(0:w952, 1:"SINGLE" ("data"), 2:i16 0 ("mode (0)")) -> (6:w953:errorcluster)  [unwired: 2 in, 1 out]
                        }
                        frame #1 {
                          n495 = while {
                            tunnel: w956 -> [w957]
                            i -> [w958]
                            stop <- w960 continue-if-true
                            n496 = GPIB Serial Poll(0:w957) -> (2:w962:i16)  [unwired: 1 in, 2 out]
                            n497 = Less?(x=w962, y=i16 128) -> (x < y?=w960:bool)
                            n498 = Wait (ms)(milliseconds to wait=u32 50) -> ()  [unwired: 1 out]
                            "Numeric" <- w958
                          }
                        }
                        frame #2 {
                          w963 = i16 2 ("mode (0)")
                          n499 = GPIB Read(0:w965, 1:200 ("byte count"), 2:i16 2 ("mode (0)"), 3:w976) -> (5:w969:string)  [unwired: 1 in, 2 out]
                          n500 = Match Pattern(string=w969, regular expression="C=") -> (after substring=w968:string)  [unwired: 1 in, 3 out]
                          n501 = Match Pattern(string=w968, regular expression="PF L=") -> (after substring=w966:string)  [unwired: 1 in, 3 out]
                          n502 = Search/Split String(string=w968, search string/char (-)=" ", offset (0)=w963) -> (substring before match=w973:string)  [unwired: 2 out]
                          n503 = Search/Split String(string=w966, search string/char (-)=" ", offset (0)=w963) -> (substring before match=w972:string)  [unwired: 2 out]
                          n504 = Fract/Exp String To Number(string=w972) -> (number=w970:dbl)  [unwired: 3 in, 1 out]
                          n505 = Fract/Exp String To Number(string=w973) -> (number=w971:dbl)  [unwired: 3 in, 1 out]
                        }
                      }
                      n506 = Build Array (concatenate)(w951, w949) -> (w948:dbl[])
                      n507 = Build Array (concatenate)(w948, w946) -> (w947:dbl[])
                    }
                  }
                  n508 = property on="array for data" class="Arr (strict)"("Value"=w943) -> ()  [unwired: 2 in, 2 out]
                }
              }
              n509 = flat-sequence {
                tunnel: w591 -> [_]
                frame #0 {
                  n510 = property on="Delib Time delay" class="DigNum (strict)"() -> ("Value"=w607:i32)  [unwired: 2 in, 2 out]
                  n511 = Wait (ms)(milliseconds to wait=w607) -> ()  [unwired: 1 out]
                }
              }
              n512 = case shown="\"Radio Selection 2\"" "Commute SorceMeter" {
                tunnel: ["13" "14"] -> w592
                frame "Radio Selection 1", Default {
                }
                frame "Radio Selection 2" {
                }
              }
              n513 = GPIB Write(0:w592, 1:":READ?", 3:w590) -> (6:w593:errorcluster)  [unwired: 2 in, 1 out]
              n514 = GPIB Read(0:w592, 1:3200, 3:w593) -> (5:w596:string)  [unwired: 2 in, 2 out]
              n515 = String Subset(string=w596, length (rest)=13) -> (substring=w597:string)  [unwired: 1 in]
              n516 = Fract/Exp String To Number(string=w597) -> (number=w599:dbl)  [unwired: 3 in, 1 out]
              n517 = Multiply(x=w599, y=-1.0) -> (x*y=w604:dbl)
              n518 = Number To Fractional String(number=w604) -> (F-format string=w601:string)  [unwired: 3 in]
              n519 = Concatenate Strings(":INIT:IMM; :SOUR:VOLT:LEV:IMM:AMPL " ("data"), w601) -> (w602:string)
              n520 = GPIB Write(0:w592, 1:w602) -> (6:w591:errorcluster)  [unwired: 3 in, 1 out]
            }
            frame #1 {
              n521 = stacked-sequence {
                tunnel: w995 -> [w998 _ _ _ _ _ _ _ _ _ _ _ _ _ _ _ _ _ _ _ _ _ _ _ _ _]
                tunnel: [w998 _ _ _ _ _ _ _ _ _ _ _ _ _ _ _ _ _ _ _ _ _ _ _ _ _] -> w981
                frame #0 {
                  # "check if oscillator on \nlock-in (address 1)\nis to be measured"
                  n522 = property on="Current is:" class="RadioBtnsControl (strict)"() -> ("Value"=w1001:T1)  [unwired: 2 in, 2 out]
                  n523 = property on="array for data" class="Arr (strict)"() -> ("Value"=w1000:dbl[])  [unwired: 2 in, 2 out]
                  n524 = Equal?(x=w1001, y=1) -> (x = y?=w1002:bool)
                  n525 = case shown="False" w1002 {
                    tunnel: w1000 -> [w1004 w1012]
                    tunnel: [w1004 w1011] -> w999
                    frame False {
                      # "we are not measuring oscillator from\nlock-in (address 1)"
                    }
                    frame True {
                      w1008 = "1"
                      # "we are  measuring oscillator"
                      n526 = GPIB Write(0:w1008, 1:"SLVL?") -> (6:w1009:errorcluster)  [unwired: 3 in, 1 out]
                      n527 = GPIB Read(0:w1008, 1:3200, 3:w1009) -> (5:w1006:string)  [unwired: 2 in, 2 out]
                      n528 = Fract/Exp String To Number(string=w1006) -> (number=w1005:dbl)  [unwired: 3 in, 1 out]
                      n529 = Build Array (concatenate)(w1012, w1005) -> (w1011:dbl[])
                    }
                  }
                  n530 = property on="array for data" class="Arr (strict)"("Value"=w999) -> ()  [unwired: 2 in, 2 out]
                }
                frame #1 {
                  # "check if in-phase\nsignal on lock-in \n(address 1) is to\nbe measured"
                  n531 = property on="array for data" class="Arr (strict)"() -> ("Value"=w1015:dbl[])  [unwired: 2 in, 2 out]
                  n532 = property on="Addr 1 lock-in" class="Bool (strict)"() -> ("Value"=w1013:bool)  [unwired: 2 in, 2 out]
                  n533 = case shown="True" w1013 {
                    tunnel: w1015 -> [w1016 w1024]
                    tunnel: [w1016 w1023] -> w1014
                    frame False {
                      # "we are not measuring in phase signal on lock-in (address 1)"
                    }
                    frame True {
                      w1021 = "1"
                      # "we are  measuring lock-in (address 1), in phase"
                      n534 = GPIB Write(0:w1021, 1:"OUTP?1") -> (6:w1022:errorcluster)  [unwired: 3 in, 1 out]
                      n535 = GPIB Read(0:w1021, 1:3200, 3:w1022) -> (5:w1019:string)  [unwired: 2 in, 2 out]
                      n536 = Fract/Exp String To Number(string=w1019) -> (number=w1018:dbl)  [unwired: 3 in, 1 out]
                      n537 = Build Array (concatenate)(w1024, w1018) -> (w1023:dbl[])
                    }
                  }
                  n538 = property on="array for data" class="Arr (strict)"("Value"=w1014) -> ()  [unwired: 2 in, 2 out]
                }
                frame #2 {
                  # "check if out-of-phase\nsignal on lock-in \n(address 1) is to\nbe measured"
                  n539 = property on="Addr 1 lock-in oop" class="Bool (strict)"() -> ("Value"=w1025:bool)  [unwired: 2 in, 2 out]
                  n540 = property on="array for data" class="Arr (strict)"() -> ("Value"=w1027:dbl[])  [unwired: 2 in, 2 out]
                  n541 = case shown="True" w1025 {
                    tunnel: w1027 -> [w1028 w1036]
                    tunnel: [w1028 w1035] -> w1026
                    frame False {
                      # "we are not measuring out-of-phase signal on lock-in (address 1)"
                    }
                    frame True {
                      w1033 = "1"
                      # "we are  measuring lock-in (address 1), out-of-phase signal"
                      n542 = GPIB Write(0:w1033, 1:"OUTP?2") -> (6:w1034:errorcluster)  [unwired: 3 in, 1 out]
                      n543 = GPIB Read(0:w1033, 1:3200, 3:w1034) -> (5:w1031:string)  [unwired: 2 in, 2 out]
                      n544 = Fract/Exp String To Number(string=w1031) -> (number=w1030:dbl)  [unwired: 3 in, 1 out]
                      n545 = Build Array (concatenate)(w1036, w1030) -> (w1035:dbl[])
                    }
                  }
                  n546 = property on="array for data" class="Arr (strict)"("Value"=w1026) -> ()  [unwired: 2 in, 2 out]
                }
                frame #3 {
                  # "check if in-phase\nsignal on lock-in \n(address 2) is to\nbe measured"
                  n547 = property on="Addr 2 lock-in" class="Bool (strict)"() -> ("Value"=w1037:bool)  [unwired: 2 in, 2 out]
                  n548 = property on="array for data" class="Arr (strict)"() -> ("Value"=w1039:dbl[])  [unwired: 2 in, 2 out]
                  n549 = case shown="False" w1037 {
                    tunnel: w1039 -> [w1040 w1048]
                    tunnel: [w1040 w1047] -> w1038
                    frame False {
                      # "we are not measuring in phase signal on lock-in (address 2)"
                    }
                    frame True {
                      w1045 = "2"
                      # "we are  measuring lock-in (address 2), in phase"
                      n550 = GPIB Write(0:w1045, 1:"OUTP?1") -> (6:w1046:errorcluster)  [unwired: 3 in, 1 out]
                      n551 = GPIB Read(0:w1045, 1:3200, 3:w1046) -> (5:w1043:string)  [unwired: 2 in, 2 out]
                      n552 = Fract/Exp String To Number(string=w1043) -> (number=w1042:dbl)  [unwired: 3 in, 1 out]
                      n553 = Build Array (concatenate)(w1048, w1042) -> (w1047:dbl[])
                    }
                  }
                  n554 = property on="array for data" class="Arr (strict)"("Value"=w1038) -> ()  [unwired: 2 in, 2 out]
                }
                frame #4 {
                  # "check if out-of-phase\nsignal on lock-in \n(address 2) is to\nbe measured"
                  n555 = property on="Addr 2 lock-in oop" class="Bool (strict)"() -> ("Value"=w1049:bool)  [unwired: 2 in, 2 out]
                  n556 = property on="array for data" class="Arr (strict)"() -> ("Value"=w1051:dbl[])  [unwired: 2 in, 2 out]
                  n557 = case shown="False" w1049 {
                    tunnel: w1051 -> [w1052 w1060]
                    tunnel: [w1052 w1059] -> w1050
                    tunnel: w1049 -> [_ _]
                    frame False {
                      # "we are not measuring out-of-phase signal on lock-in (address 2)"
                    }
                    frame True {
                      w1057 = "2"
                      # "we are  measuring lock-in (address 2), out-of-phase"
                      n558 = GPIB Write(0:w1057, 1:"OUTP?2") -> (6:w1058:errorcluster)  [unwired: 3 in, 1 out]
                      n559 = GPIB Read(0:w1057, 1:3200, 3:w1058) -> (5:w1055:string)  [unwired: 2 in, 2 out]
                      n560 = Fract/Exp String To Number(string=w1055) -> (number=w1054:dbl)  [unwired: 3 in, 1 out]
                      n561 = Build Array (concatenate)(w1060, w1054) -> (w1059:dbl[])
                    }
                  }
                  n562 = property on="array for data" class="Arr (strict)"("Value"=w1050) -> ()  [unwired: 2 in, 2 out]
                }
                frame #5 {
                  # "check if in-phase\nsignal on lock-in \n(address 3) is to\nbe measured"
                  n563 = property on="Addr 3 lock-in" class="Bool (strict)"() -> ("Value"=w1061:bool)  [unwired: 2 in, 2 out]
                  n564 = property on="array for data" class="Arr (strict)"() -> ("Value"=w1063:dbl[])  [unwired: 2 in, 2 out]
                  n565 = case shown="True" w1061 {
                    tunnel: w1063 -> [w1064 w1072]
                    tunnel: [w1064 w1071] -> w1062
                    frame False {
                      # "we are not measuring in phase signal on lock-in (address 3)"
                    }
                    frame True {
                      w1069 = "3"
                      # "we are  measuring lock-in (address 3), in phase"
                      n566 = GPIB Write(0:w1069, 1:"OUTP?1") -> (6:w1070:errorcluster)  [unwired: 3 in, 1 out]
                      n567 = GPIB Read(0:w1069, 1:3200, 3:w1070) -> (5:w1067:string)  [unwired: 2 in, 2 out]
                      n568 = Fract/Exp String To Number(string=w1067) -> (number=w1066:dbl)  [unwired: 3 in, 1 out]
                      n569 = Build Array (concatenate)(w1072, w1066) -> (w1071:dbl[])
                    }
                  }
                  n570 = property on="array for data" class="Arr (strict)"("Value"=w1062) -> ()  [unwired: 2 in, 2 out]
                }
                frame #6 {
                  # "check if out-of-phase\nsignal on lock-in \n(address 3) is to\nbe measured"
                  n571 = property on="Addr 3 lock-in oop" class="Bool (strict)"() -> ("Value"=w1073:bool)  [unwired: 2 in, 2 out]
                  n572 = property on="array for data" class="Arr (strict)"() -> ("Value"=w1075:dbl[])  [unwired: 2 in, 2 out]
                  n573 = case shown="True" w1073 {
                    tunnel: w1075 -> [w1076 w1084]
                    tunnel: [w1076 w1083] -> w1074
                    frame False {
                      # "we are not measuring out-of-phase signal on lock-in (address 3)"
                    }
                    frame True {
                      w1081 = "3"
                      # "we are  measuring lock-in (address 3), out-of-phase"
                      n574 = GPIB Write(0:w1081, 1:"OUTP?2") -> (6:w1082:errorcluster)  [unwired: 3 in, 1 out]
                      n575 = GPIB Read(0:w1081, 1:3200, 3:w1082) -> (5:w1079:string)  [unwired: 2 in, 2 out]
                      n576 = Fract/Exp String To Number(string=w1079) -> (number=w1078:dbl)  [unwired: 3 in, 1 out]
                      n577 = Build Array (concatenate)(w1084, w1078) -> (w1083:dbl[])
                    }
                  }
                  n578 = property on="array for data" class="Arr (strict)"("Value"=w1074) -> ()  [unwired: 2 in, 2 out]
                }
                frame #7 {
                  # "check if in-phase\nsignal on lock-in \n(address 4) is to\nbe measured"
                  n579 = property on="Addr 4 lock-in" class="Bool (strict)"() -> ("Value"=w1085:bool)  [unwired: 2 in, 2 out]
                  n580 = property on="array for data" class="Arr (strict)"() -> ("Value"=w1087:dbl[])  [unwired: 2 in, 2 out]
                  n581 = case shown="True" w1085 {
                    tunnel: w1087 -> [w1088 w1096]
                    tunnel: [w1088 w1095] -> w1086
                    frame False {
                      # "we are not measuring in phase signal on lock-in (address 4)"
                    }
                    frame True {
                      w1093 = "4"
                      # "we are  measuring lock-in (address 4), in phase"
                      n582 = GPIB Write(0:w1093, 1:"OUTP?1") -> (6:w1094:errorcluster)  [unwired: 3 in, 1 out]
                      n583 = GPIB Read(0:w1093, 1:3200, 3:w1094) -> (5:w1091:string)  [unwired: 2 in, 2 out]
                      n584 = Fract/Exp String To Number(string=w1091) -> (number=w1090:dbl)  [unwired: 3 in, 1 out]
                      n585 = Build Array (concatenate)(w1096, w1090) -> (w1095:dbl[])
                    }
                  }
                  n586 = property on="array for data" class="Arr (strict)"("Value"=w1086) -> ()  [unwired: 2 in, 2 out]
                }
                frame #8 {
                  # "check if out-of-phase\nsignal on lock-in \n(address 4) is to\nbe measured"
                  n587 = property on="Addr 4 lock-in oop" class="Bool (strict)"() -> ("Value"=w1097:bool)  [unwired: 2 in, 2 out]
                  n588 = property on="array for data" class="Arr (strict)"() -> ("Value"=w1099:dbl[])  [unwired: 2 in, 2 out]
                  n589 = case shown="True" w1097 {
                    tunnel: w1099 -> [w1100 w1108]
                    tunnel: [w1100 w1107] -> w1098
                    frame False {
                      # "we are not measuring out-of-phase signal on lock-in (address 4)"
                    }
                    frame True {
                      w1105 = "4"
                      # "we are  measuring lock-in (address 4), out-of-phase"
                      n590 = GPIB Write(0:w1105, 1:"OUTP?2") -> (6:w1106:errorcluster)  [unwired: 3 in, 1 out]
                      n591 = GPIB Read(0:w1105, 1:3200, 3:w1106) -> (5:w1103:string)  [unwired: 2 in, 2 out]
                      n592 = Fract/Exp String To Number(string=w1103) -> (number=w1102:dbl)  [unwired: 3 in, 1 out]
                      n593 = Build Array (concatenate)(w1108, w1102) -> (w1107:dbl[])
                    }
                  }
                  n594 = property on="array for data" class="Arr (strict)"("Value"=w1098) -> ()  [unwired: 2 in, 2 out]
                }
                frame #9 {
                  # "check if in-phase\nsignal on lock-in \n(address 5) is to\nbe measured"
                  n595 = property on="Addr 5 lock-in" class="Bool (strict)"() -> ("Value"=w1109:bool)  [unwired: 2 in, 2 out]
                  n596 = property on="array for data" class="Arr (strict)"() -> ("Value"=w1111:dbl[])  [unwired: 2 in, 2 out]
                  n597 = case shown="False" w1109 {
                    tunnel: w1111 -> [w1112 w1120]
                    tunnel: [w1112 w1119] -> w1110
                    frame False {
                      # "we are not measuring in phase signal on lock-in (address 5)"
                    }
                    frame True {
                      w1117 = "5"
                      # "we are  measuring lock-in (address 5), in phase"
                      n598 = GPIB Write(0:w1117, 1:"OUTP?1") -> (6:w1118:errorcluster)  [unwired: 3 in, 1 out]
                      n599 = GPIB Read(0:w1117, 1:3200, 3:w1118) -> (5:w1115:string)  [unwired: 2 in, 2 out]
                      n600 = Fract/Exp String To Number(string=w1115) -> (number=w1114:dbl)  [unwired: 3 in, 1 out]
                      n601 = Build Array (concatenate)(w1120, w1114) -> (w1119:dbl[])
                    }
                  }
                  n602 = property on="array for data" class="Arr (strict)"("Value"=w1110) -> ()  [unwired: 2 in, 2 out]
                }
                frame #10 {
                  # "check if out-of-phase\nsignal on lock-in \n(address 5) is to\nbe measured"
                  n603 = property on="Addr 5 lock-in oop" class="Bool (strict)"() -> ("Value"=w1121:bool)  [unwired: 2 in, 2 out]
                  n604 = property on="array for data" class="Arr (strict)"() -> ("Value"=w1123:dbl[])  [unwired: 2 in, 2 out]
                  n605 = case shown="False" w1121 {
                    tunnel: w1123 -> [w1124 w1132]
                    tunnel: [w1124 w1131] -> w1122
                    frame False {
                      # "we are not measuring out-of-phase signal on lock-in (address 5)"
                    }
                    frame True {
                      w1129 = "5"
                      # "we are  measuring lock-in (address 5), out-of-phase"
                      n606 = GPIB Write(0:w1129, 1:"OUTP?2") -> (6:w1130:errorcluster)  [unwired: 3 in, 1 out]
                      n607 = GPIB Read(0:w1129, 1:3200, 3:w1130) -> (5:w1127:string)  [unwired: 2 in, 2 out]
                      n608 = Fract/Exp String To Number(string=w1127) -> (number=w1126:dbl)  [unwired: 3 in, 1 out]
                      n609 = Build Array (concatenate)(w1132, w1126) -> (w1131:dbl[])
                    }
                  }
                  n610 = property on="array for data" class="Arr (strict)"("Value"=w1122) -> ()  [unwired: 2 in, 2 out]
                }
                frame #11 {
                  # "check if voltage on \nmain Keithley 2400 \n(addr. 12) is to\nbe measured"
                  n611 = property on="Voltage (Vk1)" class="Bool (strict)"() -> ("Value"=w1133:bool)  [unwired: 2 in, 2 out]
                  n612 = property on="array for data" class="Arr (strict)"() -> ("Value"=w1135:dbl[])  [unwired: 2 in, 2 out]
                  n613 = case shown="False" w1133 {
                    tunnel: w1135 -> [w1136 w1146]
                    tunnel: [w1136 w1145] -> w1134
                    frame False {
                      # "we aren't measuring voltage \non main Keithley 2400 (addr. 12)"
                    }
                    frame True {
                      w1143 = "12"
                      # "we are measuring voltage \non main Keithley 2400 (addr. 12)"
                      n614 = GPIB Write(0:w1143, 1:":READ?") -> (6:w1144:errorcluster)  [unwired: 3 in, 1 out]
                      n615 = GPIB Read(0:w1143, 1:3200, 3:w1144) -> (5:w1139:string)  [unwired: 2 in, 2 out]
                      n616 = String Subset(string=w1139, length (rest)=13) -> (substring=w1138:string)  [unwired: 1 in]
                      n617 = Fract/Exp String To Number(string=w1138) -> (number=w1141:dbl)  [unwired: 3 in, 1 out]
                      n618 = Build Array (concatenate)(w1146, w1141) -> (w1145:dbl[])
                    }
                  }
                  n619 = property on="array for data" class="Arr (strict)"("Value"=w1134) -> ()  [unwired: 2 in, 2 out]
                }
                frame #12 {
                  # "check if  current on \nmain Keithley 2400 \n(addr. 12) is to\nbe measured"
                  n620 = property on="Current (Ik1)" class="Bool (strict)"() -> ("Value"=w1147:bool)  [unwired: 2 in, 2 out]
                  n621 = property on="array for data" class="Arr (strict)"() -> ("Value"=w1149:dbl[])  [unwired: 2 in, 2 out]
                  n622 = case shown="True" w1147 {
                    tunnel: w1149 -> [w1150 w1161]
                    tunnel: [w1150 w1160] -> w1148
                    frame False {
                      # "we aren't measuring current \non main Keithley 2400 (addr. 12)"
                    }
                    frame True {
                      w1158 = "12"
                      # "we are measuring current\non main Keithley 2400 (addr. 12)"
                      n623 = GPIB Write(0:w1158, 1:":READ?") -> (6:w1159:errorcluster)  [unwired: 3 in, 1 out]
                      n624 = GPIB Read(0:w1158, 1:3200, 3:w1159) -> (5:w1154:string)  [unwired: 2 in, 2 out]
                      n625 = String Subset(string=w1154, offset (0)=14, length (rest)=13) -> (substring=w1153:string)
                      n626 = Fract/Exp String To Number(string=w1153) -> (number=w1156:dbl)  [unwired: 3 in, 1 out]
                      n627 = Build Array (concatenate)(w1161, w1156) -> (w1160:dbl[])
                    }
                  }
                  n628 = property on="array for data" class="Arr (strict)"("Value"=w1148) -> ()  [unwired: 2 in, 2 out]
                }
                frame #13 {
                  # "check if voltage on \nadd. Keithley 2400 \n(addr. 13) is to\nbe measured"
                  n629 = property on="Voltage (Vk2)" class="Bool (strict)"() -> ("Value"=w1162:bool)  [unwired: 2 in, 2 out]
                  n630 = property on="array for data" class="Arr (strict)"() -> ("Value"=w1164:dbl[])  [unwired: 2 in, 2 out]
                  n631 = case shown="True" w1162 {
                    tunnel: w1164 -> [w1165 w1175]
                    tunnel: [w1165 w1174] -> w1163
                    frame False {
                      # "we aren't measuring voltage \non additional Keithley 2400 (addr. 13)"
                    }
                    frame True {
                      w1172 = "13"
                      # "we are measuring voltage \non additional Keithley 2400 (addr. 13)"
                      n632 = GPIB Write(0:w1172, 1:":READ?") -> (6:w1173:errorcluster)  [unwired: 3 in, 1 out]
                      n633 = GPIB Read(0:w1172, 1:3200, 3:w1173) -> (5:w1168:string)  [unwired: 2 in, 2 out]
                      n634 = String Subset(string=w1168, length (rest)=13) -> (substring=w1167:string)  [unwired: 1 in]
                      n635 = Fract/Exp String To Number(string=w1167) -> (number=w1170:dbl)  [unwired: 3 in, 1 out]
                      n636 = Build Array (concatenate)(w1175, w1170) -> (w1174:dbl[])
                    }
                  }
                  n637 = property on="array for data" class="Arr (strict)"("Value"=w1163) -> ()  [unwired: 2 in, 2 out]
                }
                frame #14 {
                  # "check if  current on \nadd. Keithley 2400 \n(addr. 13) is to\nbe measured"
                  n638 = property on="Current (Ik2)" class="Bool (strict)"() -> ("Value"=w1176:bool)  [unwired: 2 in, 2 out]
                  n639 = property on="array for data" class="Arr (strict)"() -> ("Value"=w1178:dbl[])  [unwired: 2 in, 2 out]
                  n640 = case shown="True" w1176 {
                    tunnel: w1178 -> [w1179 w1190]
                    tunnel: [w1179 w1189] -> w1177
                    frame False {
                      # "we aren't measuring current \non additional Keithley 2400 (addr. 13)"
                    }
                    frame True {
                      w1187 = "13"
                      # "we are measuring current\non additional Keithley 2400 (addr. 13)"
                      n641 = GPIB Write(0:w1187, 1:":READ?") -> (6:w1188:errorcluster)  [unwired: 3 in, 1 out]
                      n642 = GPIB Read(0:w1187, 1:3200, 3:w1188) -> (5:w1183:string)  [unwired: 2 in, 2 out]
                      n643 = String Subset(string=w1183, offset (0)=14, length (rest)=13) -> (substring=w1182:string)
                      n644 = Fract/Exp String To Number(string=w1182) -> (number=w1185:dbl)  [unwired: 3 in, 1 out]
                      n645 = Build Array (concatenate)(w1190, w1185) -> (w1189:dbl[])
                    }
                  }
                  n646 = property on="array for data" class="Arr (strict)"("Value"=w1177) -> ()  [unwired: 2 in, 2 out]
                }
                frame #15 {
                  # "check if voltage on \nadd. Keithley 2400 \n(addr. 14) is to\nbe measured"
                  n647 = property on="Voltage (Vk3)" class="Bool (strict)"() -> ("Value"=w1191:bool)  [unwired: 2 in, 2 out]
                  n648 = property on="array for data" class="Arr (strict)"() -> ("Value"=w1193:dbl[])  [unwired: 2 in, 2 out]
                  n649 = case shown="False" w1191 {
                    tunnel: w1193 -> [w1194 w1204]
                    tunnel: [w1194 w1203] -> w1192
                    frame False {
                      # "we aren't measuring voltage \non additional Keithley 2400 (addr. 14)"
                    }
                    frame True {
                      w1201 = "14"
                      # "we are measuring voltage \non additional Keithley 2400 (addr. 14)"
                      n650 = GPIB Write(0:w1201, 1:":READ?") -> (6:w1202:errorcluster)  [unwired: 3 in, 1 out]
                      n651 = GPIB Read(0:w1201, 1:3200, 3:w1202) -> (5:w1197:string)  [unwired: 2 in, 2 out]
                      n652 = String Subset(string=w1197, length (rest)=13) -> (substring=w1196:string)  [unwired: 1 in]
                      n653 = Fract/Exp String To Number(string=w1196) -> (number=w1199:dbl)  [unwired: 3 in, 1 out]
                      n654 = Build Array (concatenate)(w1204, w1199) -> (w1203:dbl[])
                    }
                  }
                  n655 = property on="array for data" class="Arr (strict)"("Value"=w1192) -> ()  [unwired: 2 in, 2 out]
                }
                frame #16 {
                  # "check if  current on \nadd. Keithley 2400 \n(addr. 14) is to\nbe measured"
                  n656 = property on="Current (Ik3)" class="Bool (strict)"() -> ("Value"=w1205:bool)  [unwired: 2 in, 2 out]
                  n657 = property on="array for data" class="Arr (strict)"() -> ("Value"=w1207:dbl[])  [unwired: 2 in, 2 out]
                  n658 = case shown="True" w1205 {
                    tunnel: w1207 -> [w1208 w1219]
                    tunnel: [w1208 w1218] -> w1206
                    frame False {
                      # "we aren't measuring current \non additional Keithley 2400 (addr. 14)"
                    }
                    frame True {
                      w1216 = "14"
                      # "we are measuring current\non additional Keithley 2400 (addr. 14)"
                      n659 = GPIB Write(0:w1216, 1:":READ?") -> (6:w1217:errorcluster)  [unwired: 3 in, 1 out]
                      n660 = GPIB Read(0:w1216, 1:3200, 3:w1217) -> (5:w1212:string)  [unwired: 2 in, 2 out]
                      n661 = String Subset(string=w1212, offset (0)=14, length (rest)=13) -> (substring=w1211:string)
                      n662 = Fract/Exp String To Number(string=w1211) -> (number=w1214:dbl)  [unwired: 3 in, 1 out]
                      n663 = Build Array (concatenate)(w1219, w1214) -> (w1218:dbl[])
                    }
                  }
                  n664 = property on="array for data" class="Arr (strict)"("Value"=w1206) -> ()  [unwired: 2 in, 2 out]
                }
                frame #17 {
                  # "check if 1st channel\non Keithley 2182 \n(addr. 15) is to\nbe measured"
                  n665 = property on="Channel 1 (Vnano1)" class="Bool (strict)"() -> ("Value"=w1220:bool)  [unwired: 2 in, 2 out]
                  n666 = property on="array for data" class="Arr (strict)"() -> ("Value"=w1222:dbl[])  [unwired: 2 in, 2 out]
                  n667 = case shown="True" w1220 {
                    tunnel: w1222 -> [w1223 w1231]
                    tunnel: [w1223 w1230] -> w1221
                    frame False {
                      # "we are not measuring 1st channel\non Keithley 2182 (addr. 15)"
                    }
                    frame True {
                      w1228 = "15"
                      # "we are measuring 1st channel\non Keithley 2182 (addr. 15)"
                      n668 = GPIB Write(0:w1228, 1:":SENSe:DATA:FRES?") -> (6:w1229:errorcluster)  [unwired: 3 in, 1 out]
                      n669 = GPIB Read(0:w1228, 1:200, 3:w1229) -> (5:w1224:string)  [unwired: 2 in, 2 out]
                      n670 = Fract/Exp String To Number(string=w1224) -> (number=w1226:dbl)  [unwired: 3 in, 1 out]
                      n671 = Build Array (concatenate)(w1231, w1226) -> (w1230:dbl[])
                    }
                  }
                  n672 = property on="array for data" class="Arr (strict)"("Value"=w1221) -> ()  [unwired: 2 in, 2 out]
                }
                frame #18 {
                  # "check if 2nd channel\non Keithley 2182 \n(addr. 15) is to\nbe measured"
                  n673 = property on="Channel 2 (Vnano1b)" class="Bool (strict)"() -> ("Value"=w1232:bool)  [unwired: 2 in, 2 out]
                  n674 = property on="array for data" class="Arr (strict)"() -> ("Value"=w1234:dbl[])  [unwired: 2 in, 2 out]
                  n675 = case shown="False" w1232 {
                    tunnel: w1234 -> [w1235 w1247]
                    tunnel: [w1235 w1246] -> w1233
                    frame False {
                      # "we are not measuring 1st channel\non Keithley 2182 (addr. 15)"
                    }
                    frame True {
                      w1238 = "15"
                      # "switching to channel 2 and then\nback to channel 1"
                      # "we are measuring 2nd channel\non Keithley 2182 (addr. 15)"
                      n676 = GPIB Write(0:w1238, 1:":SENSe:CHAN 2") -> (6:w1239:errorcluster)  [unwired: 3 in, 1 out]
                      n677 = GPIB Write(0:w1238, 1:":SENSe:DATA:FRES?", 3:w1239) -> (6:w1245:errorcluster)  [unwired: 2 in, 1 out]
                      n678 = GPIB Read(0:w1238, 1:200, 3:w1245) -> (5:w1241:string, 7:w1237:errorcluster)  [unwired: 2 in, 1 out]
                      n679 = GPIB Write(0:w1238, 1:":SENSe:CHAN 1", 3:w1237) -> ()  [unwired: 2 in, 2 out]
                      n680 = Fract/Exp String To Number(string=w1241) -> (number=w1243:dbl)  [unwired: 3 in, 1 out]
                      n681 = Build Array (concatenate)(w1247, w1243) -> (w1246:dbl[])
                    }
                  }
                  n682 = property on="array for data" class="Arr (strict)"("Value"=w1233) -> ()  [unwired: 2 in, 2 out]
                }
                frame #19 {
                  # "check if 1st channel\non Keithley 2182 \n(addr. 16) is to\nbe measured"
                  n683 = property on="Channel 1 (Vnano2)" class="Bool (strict)"() -> ("Value"=w1248:bool)  [unwired: 2 in, 2 out]
                  n684 = property on="array for data" class="Arr (strict)"() -> ("Value"=w1250:dbl[])  [unwired: 2 in, 2 out]
                  n685 = case shown="True" w1248 {
                    tunnel: w1250 -> [w1251 w1259]
                    tunnel: [w1251 w1258] -> w1249
                    frame False {
                      # "we are not measuring 1st channel\non Keithley 2182 (addr. 16)"
                    }
                    frame True {
                      w1256 = "16"
                      # "we are measuring 1st channel\non Keithley 2182 (addr. 16)"
                      n686 = GPIB Write(0:w1256, 1:":SENSe:DATA:FRES?") -> (6:w1257:errorcluster)  [unwired: 3 in, 1 out]
                      n687 = GPIB Read(0:w1256, 1:200, 3:w1257) -> (5:w1252:string)  [unwired: 2 in, 2 out]
                      n688 = Fract/Exp String To Number(string=w1252) -> (number=w1254:dbl)  [unwired: 3 in, 1 out]
                      n689 = Build Array (concatenate)(w1259, w1254) -> (w1258:dbl[])
                    }
                  }
                  n690 = property on="array for data" class="Arr (strict)"("Value"=w1249) -> ()  [unwired: 2 in, 2 out]
                }
                frame #20 {
                  # "check if 2nd channel\non Keithley 2182 \n(addr. 16) is to\nbe measured"
                  n691 = property on="Channel 2 (Vnano2b)" class="Bool (strict)"() -> ("Value"=w1260:bool)  [unwired: 2 in, 2 out]
                  n692 = property on="array for data" class="Arr (strict)"() -> ("Value"=w1262:dbl[])  [unwired: 2 in, 2 out]
                  n693 = case shown="True" w1260 {
                    tunnel: w1262 -> [w1263 w1275]
                    tunnel: [w1263 w1274] -> w1261
                    frame False {
                      # "we are not measuring 1st channel\non Keithley 2182 (addr. 16)"
                    }
                    frame True {
                      w1266 = "16"
                      # "switching to channel 2 and then\nback to channel 1"
                      # "we are measuring 2nd channel\non Keithley 2182 (addr. 16)"
                      n694 = GPIB Write(0:w1266, 1:":SENSe:CHAN 2") -> (6:w1267:errorcluster)  [unwired: 3 in, 1 out]
                      n695 = GPIB Write(0:w1266, 1:":SENSe:DATA:FRES?", 3:w1267) -> (6:w1273:errorcluster)  [unwired: 2 in, 1 out]
                      n696 = GPIB Read(0:w1266, 1:200, 3:w1273) -> (5:w1269:string, 7:w1265:errorcluster)  [unwired: 2 in, 1 out]
                      n697 = GPIB Write(0:w1266, 1:":SENSe:CHAN 1", 3:w1265) -> ()  [unwired: 2 in, 2 out]
                      n698 = Fract/Exp String To Number(string=w1269) -> (number=w1271:dbl)  [unwired: 3 in, 1 out]
                      n699 = Build Array (concatenate)(w1275, w1271) -> (w1274:dbl[])
                    }
                  }
                  n700 = property on="array for data" class="Arr (strict)"("Value"=w1261) -> ()  [unwired: 2 in, 2 out]
                }
                frame #21 {
                  # "check if 1st channel\non Keithley 2182 \n(addr. 17) is to\nbe measured"
                  n701 = property on="Channel 1 (Vnano3)" class="Bool (strict)"() -> ("Value"=w1276:bool)  [unwired: 2 in, 2 out]
                  n702 = property on="array for data" class="Arr (strict)"() -> ("Value"=w1278:dbl[])  [unwired: 2 in, 2 out]
                  n703 = case shown="True" w1276 {
                    tunnel: w1278 -> [w1279 w1287]
                    tunnel: [w1279 w1286] -> w1277
                    frame False {
                      # "we are not measuring 1st channel\non Keithley 2182 (addr. 17)"
                    }
                    frame True {
                      w1284 = "17"
                      # "we are measuring 1st channel\non Keithley 2182 (addr. 17)"
                      n704 = GPIB Write(0:w1284, 1:":SENSe:DATA:FRES?") -> (6:w1285:errorcluster)  [unwired: 3 in, 1 out]
                      n705 = GPIB Read(0:w1284, 1:200, 3:w1285) -> (5:w1280:string)  [unwired: 2 in, 2 out]
                      n706 = Fract/Exp String To Number(string=w1280) -> (number=w1282:dbl)  [unwired: 3 in, 1 out]
                      n707 = Build Array (concatenate)(w1287, w1282) -> (w1286:dbl[])
                    }
                  }
                  n708 = property on="array for data" class="Arr (strict)"("Value"=w1277) -> ()  [unwired: 2 in, 2 out]
                }
                frame #22 {
                  # "check if 2nd channel\non Keithley 2182 \n(addr. 17) is to\nbe measured"
                  n709 = property on="Channel 2 (Vnano3b)" class="Bool (strict)"() -> ("Value"=w1288:bool)  [unwired: 2 in, 2 out]
                  n710 = property on="array for data" class="Arr (strict)"() -> ("Value"=w1290:dbl[])  [unwired: 2 in, 2 out]
                  n711 = case shown="True" w1288 {
                    tunnel: w1290 -> [w1291 w1303]
                    tunnel: [w1291 w1302] -> w1289
                    frame False {
                      # "we are not measuring 1st channel\non Keithley 2182 (addr. 17)"
                    }
                    frame True {
                      w1294 = "17"
                      # "switching to channel 2 and then\nback to channel 1"
                      # "we are measuring 2nd channel\non Keithley 2182 (addr. 17)"
                      n712 = GPIB Write(0:w1294, 1:":SENSe:CHAN 2") -> (6:w1295:errorcluster)  [unwired: 3 in, 1 out]
                      n713 = GPIB Write(0:w1294, 1:":SENSe:DATA:FRES?", 3:w1295) -> (6:w1301:errorcluster)  [unwired: 2 in, 1 out]
                      n714 = GPIB Read(0:w1294, 1:200, 3:w1301) -> (5:w1297:string, 7:w1293:errorcluster)  [unwired: 2 in, 1 out]
                      n715 = GPIB Write(0:w1294, 1:":SENSe:CHAN 1", 3:w1293) -> ()  [unwired: 2 in, 2 out]
                      n716 = Fract/Exp String To Number(string=w1297) -> (number=w1299:dbl)  [unwired: 3 in, 1 out]
                      n717 = Build Array (concatenate)(w1303, w1299) -> (w1302:dbl[])
                    }
                  }
                  n718 = property on="array for data" class="Arr (strict)"("Value"=w1289) -> ()  [unwired: 2 in, 2 out]
                }
                frame #23 {
                  # "check if 1st \nthermometer on \nOxford ITC \n(address 24) \nis measured"
                  n719 = property on="Thermometer 1 (T1)" class="Bool (strict)"() -> ("Value"=w1304:bool)  [unwired: 2 in, 2 out]
                  n720 = property on="array for data" class="Arr (strict)"() -> ("Value"=w1306:dbl[])  [unwired: 2 in, 2 out]
                  n721 = case shown="True" w1304 {
                    tunnel: w1306 -> [w1307 w1316]
                    tunnel: [w1307 w1315] -> w1305
                    frame False {
                      # "we are not measuring temperature on\nthermometer 1 (addr. 24)"
                    }
                    frame True {
                      w1308 = 1
                      w1313 = "24"
                      # "we are measuring temperature,\nthermometer 1 (addr. 24)"
                      n722 = GPIB Write(0:w1313, 1:"R 1", 2:w1308) -> (6:w1314:errorcluster)  [unwired: 2 in, 1 out]
                      n723 = GPIB Read(0:w1313, 1:200, 2:w1308, 3:w1314) -> (5:w1309:string)  [unwired: 1 in, 2 out]
                      n724 = Fract/Exp String To Number(string=w1309, offset=w1308) -> (number=w1311:dbl)  [unwired: 2 in, 1 out]
                      n725 = Build Array (concatenate)(w1316, w1311) -> (w1315:dbl[])
                    }
                  }
                  n726 = property on="array for data" class="Arr (strict)"("Value"=w1305) -> ()  [unwired: 2 in, 2 out]
                }
                frame #24 {
                  # "check if 1st \nthermometer on \nOxford ITC \n(address 24) \nis measured"
                  n727 = property on="Magnetic Field (B)" class="Bool (strict)"() -> ("Value"=w1317:bool)  [unwired: 2 in, 2 out]
                  n728 = property on="array for data" class="Arr (strict)"() -> ("Value"=w1319:dbl[])  [unwired: 2 in, 2 out]
                  n729 = case shown="True" w1317 {
                    tunnel: w1319 -> [w1320 w1329]
                    tunnel: [w1320 w1328] -> w1318
                    frame False {
                      # "we are not measuringmagnetic field (addr. 25)"
                    }
                    frame True {
                      w1321 = 1
                      w1326 = "25"
                      # "we are measuring magnetic field  (addr. 25)"
                      n730 = GPIB Write(0:w1326, 1:"R 8", 2:w1321) -> (6:w1327:errorcluster)  [unwired: 2 in, 1 out]
                      n731 = GPIB Read(0:w1326, 1:200, 2:w1321, 3:w1327) -> (5:w1322:string)  [unwired: 1 in, 2 out]
                      n732 = Fract/Exp String To Number(string=w1322, offset=w1321) -> (number=w1324:dbl)  [unwired: 2 in, 1 out]
                      n733 = Build Array (concatenate)(w1329, w1324) -> (w1328:dbl[])
                    }
                  }
                  n734 = property on="array for data" class="Arr (strict)"("Value"=w1318) -> ()  [unwired: 2 in, 2 out]
                }
                frame #25 {
                  # "check if capacitance\nand loss (address 28)\nare measured"
                  n735 = property on="Capacitance (C) and Loss (L)" class="Bool (strict)"() -> ("Value"=w1330:bool)  [unwired: 2 in, 2 out]
                  n736 = property on="array for data" class="Arr (strict)"() -> ("Value"=w1332:dbl[])  [unwired: 2 in, 2 out]
                  n737 = case shown="True" w1330 {
                    tunnel: w1332 -> [w1333 w1339]
                    tunnel: [w1333 w1335] -> w1331
                    frame False {
                      # "we are not measuringmagnetic capacitance (addr. 28)"
                    }
                    frame True {
                      # "we are measuring capacitance and loss  (addr. 28)"
                      n738 = stacked-sequence {
                        seq-local: [w1341 _ _] -> [_ _ w1364]
                        tunnel: [_ _ w1358] -> w1334
                        tunnel: [_ _ w1359] -> w1337
                        tunnel: "28" ("data") -> [w1340 w1344 w1353]
                        frame #0 {
                          n739 = GPIB Write(0:w1340, 1:"SINGLE" ("data"), 2:i16 0 ("mode (0)")) -> (6:w1341:errorcluster)  [unwired: 2 in, 1 out]
                        }
                        frame #1 {
                          n740 = while {
                            tunnel: w1344 -> [w1345]
                            i -> [w1346]
                            stop <- w1348 continue-if-true
                            n741 = GPIB Serial Poll(0:w1345) -> (2:w1350:i16)  [unwired: 1 in, 2 out]
                            n742 = Less?(x=w1350, y=i16 128) -> (x < y?=w1348:bool)
                            n743 = Wait (ms)(milliseconds to wait=u32 50) -> ()  [unwired: 1 out]
                            "Numeric 4" <- w1346
                          }
                        }
                        frame #2 {
                          w1351 = i16 2 ("mode (0)")
                          n744 = GPIB Read(0:w1353, 1:200 ("byte count"), 2:i16 2 ("mode (0)"), 3:w1364) -> (5:w1357:string)  [unwired: 1 in, 2 out]
                          n745 = Match Pattern(string=w1357, regular expression="C=") -> (after substring=w1356:string)  [unwired: 1 in, 3 out]
                          n746 = Match Pattern(string=w1356, regular expression="PF L=") -> (after substring=w1354:string)  [unwired: 1 in, 3 out]
                          n747 = Search/Split String(string=w1356, search string/char (-)=" ", offset (0)=w1351) -> (substring before match=w1361:string)  [unwired: 2 out]
                          n748 = Search/Split String(string=w1354, search string/char (-)=" ", offset (0)=w1351) -> (substring before match=w1360:string)  [unwired: 2 out]
                          n749 = Fract/Exp String To Number(string=w1360) -> (number=w1358:dbl)  [unwired: 3 in, 1 out]
                          n750 = Fract/Exp String To Number(string=w1361) -> (number=w1359:dbl)  [unwired: 3 in, 1 out]
                        }
                      }
                      n751 = Build Array (concatenate)(w1339, w1337) -> (w1336:dbl[])
                      n752 = Build Array (concatenate)(w1336, w1334) -> (w1335:dbl[])
                    }
                  }
                  n753 = property on="array for data" class="Arr (strict)"("Value"=w1331) -> ()  [unwired: 2 in, 2 out]
                }
              }
              n754 = property on="Commute SorceMeter" class="RadioBtnsControl (strict)"() -> ("Value"=w979:enum32{"Radio Selection 1", "Radio Selection 2"})  [unwired: 2 in, 2 out]
              n755 = case shown="\"Radio Selection 1\", Default" w979 {
                tunnel: ["13" "14"] -> w982
                frame "Radio Selection 1", Default {
                }
                frame "Radio Selection 2" {
                }
              }
              n756 = GPIB Write(0:w982, 1:":READ?", 3:w981) -> (6:w983:errorcluster)  [unwired: 2 in, 1 out]
              n757 = GPIB Read(0:w982, 1:3200, 3:w983) -> (5:w986:string)  [unwired: 2 in, 2 out]
              n758 = String Subset(string=w986, length (rest)=13) -> (substring=w987:string)  [unwired: 1 in]
              n759 = Fract/Exp String To Number(string=w987) -> (number=w989:dbl)  [unwired: 3 in, 1 out]
              n760 = Multiply(x=w989, y=-1.0) -> (x*y=w994:dbl)
              n761 = Number To Fractional String(number=w994) -> (F-format string=w991:string)  [unwired: 3 in]
              n762 = Concatenate Strings(":INIT:IMM; :SOUR:VOLT:LEV:IMM:AMPL " ("data"), w991) -> (w992:string)
              n763 = GPIB Write(0:w982, 1:w992) -> (6:w980:errorcluster)  [unwired: 3 in, 1 out]
            }
          }
        }
        frame False {
          # "all measurements are done in this stacked sequence; reading from each device is recorded to \"array for data\""
          n764 = stacked-sequence {
            tunnel: w1367 -> [w1369 _ _ _ _ _ _ _ _ _ _ _ _ _ _ _ _ _ _ _ _ _ _ _ _ _]
            tunnel: [w1369 _ _ _ _ _ _ _ _ _ _ _ _ _ _ _ _ _ _ _ _ _ _ _ _ _] -> w1368
            frame #0 {
              # "check if oscillator on \nlock-in (address 1)\nis to be measured"
              n765 = property on="Current is:" class="RadioBtnsControl (strict)"() -> ("Value"=w1372:T1)  [unwired: 2 in, 2 out]
              n766 = property on="array for data" class="Arr (strict)"() -> ("Value"=w1371:dbl[])  [unwired: 2 in, 2 out]
              n767 = Equal?(x=w1372, y=1) -> (x = y?=w1373:bool)
              n768 = case shown="False" w1373 {
                tunnel: w1371 -> [w1375 w1383]
                tunnel: [w1375 w1382] -> w1370
                frame False {
                  # "we are not measuring oscillator from\nlock-in (address 1)"
                }
                frame True {
                  w1379 = "1"
                  # "we are  measuring oscillator"
                  n769 = GPIB Write(0:w1379, 1:"SLVL?") -> (6:w1380:errorcluster)  [unwired: 3 in, 1 out]
                  n770 = GPIB Read(0:w1379, 1:3200, 3:w1380) -> (5:w1377:string)  [unwired: 2 in, 2 out]
                  n771 = Fract/Exp String To Number(string=w1377) -> (number=w1376:dbl)  [unwired: 3 in, 1 out]
                  n772 = Build Array (concatenate)(w1383, w1376) -> (w1382:dbl[])
                }
              }
              n773 = property on="array for data" class="Arr (strict)"("Value"=w1370) -> ()  [unwired: 2 in, 2 out]
            }
            frame #1 {
              # "check if in-phase\nsignal on lock-in \n(address 1) is to\nbe measured"
              n774 = property on="array for data" class="Arr (strict)"() -> ("Value"=w1386:dbl[])  [unwired: 2 in, 2 out]
              n775 = property on="Addr 1 lock-in" class="Bool (strict)"() -> ("Value"=w1384:bool)  [unwired: 2 in, 2 out]
              n776 = case shown="False" w1384 {
                tunnel: w1386 -> [w1387 w1395]
                tunnel: [w1387 w1394] -> w1385
                frame False {
                  # "we are not measuring in phase signal on lock-in (address 1)"
                }
                frame True {
                  w1392 = "1"
                  # "we are  measuring lock-in (address 1), in phase"
                  n777 = GPIB Write(0:w1392, 1:"OUTP?1") -> (6:w1393:errorcluster)  [unwired: 3 in, 1 out]
                  n778 = GPIB Read(0:w1392, 1:3200, 3:w1393) -> (5:w1390:string)  [unwired: 2 in, 2 out]
                  n779 = Fract/Exp String To Number(string=w1390) -> (number=w1389:dbl)  [unwired: 3 in, 1 out]
                  n780 = Build Array (concatenate)(w1395, w1389) -> (w1394:dbl[])
                }
              }
              n781 = property on="array for data" class="Arr (strict)"("Value"=w1385) -> ()  [unwired: 2 in, 2 out]
            }
            frame #2 {
              # "check if out-of-phase\nsignal on lock-in \n(address 1) is to\nbe measured"
              n782 = property on="Addr 1 lock-in oop" class="Bool (strict)"() -> ("Value"=w1396:bool)  [unwired: 2 in, 2 out]
              n783 = property on="array for data" class="Arr (strict)"() -> ("Value"=w1398:dbl[])  [unwired: 2 in, 2 out]
              n784 = case shown="False" w1396 {
                tunnel: w1398 -> [w1399 w1407]
                tunnel: [w1399 w1406] -> w1397
                frame False {
                  # "we are not measuring out-of-phase signal on lock-in (address 1)"
                }
                frame True {
                  w1404 = "1"
                  # "we are  measuring lock-in (address 1), out-of-phase signal"
                  n785 = GPIB Write(0:w1404, 1:"OUTP?2") -> (6:w1405:errorcluster)  [unwired: 3 in, 1 out]
                  n786 = GPIB Read(0:w1404, 1:3200, 3:w1405) -> (5:w1402:string)  [unwired: 2 in, 2 out]
                  n787 = Fract/Exp String To Number(string=w1402) -> (number=w1401:dbl)  [unwired: 3 in, 1 out]
                  n788 = Build Array (concatenate)(w1407, w1401) -> (w1406:dbl[])
                }
              }
              n789 = property on="array for data" class="Arr (strict)"("Value"=w1397) -> ()  [unwired: 2 in, 2 out]
            }
            frame #3 {
              # "check if in-phase\nsignal on lock-in \n(address 2) is to\nbe measured"
              n790 = property on="Addr 2 lock-in" class="Bool (strict)"() -> ("Value"=w1408:bool)  [unwired: 2 in, 2 out]
              n791 = property on="array for data" class="Arr (strict)"() -> ("Value"=w1410:dbl[])  [unwired: 2 in, 2 out]
              n792 = case shown="False" w1408 {
                tunnel: w1410 -> [w1411 w1419]
                tunnel: [w1411 w1418] -> w1409
                frame False {
                  # "we are not measuring in phase signal on lock-in (address 2)"
                }
                frame True {
                  w1416 = "2"
                  # "we are  measuring lock-in (address 2), in phase"
                  n793 = GPIB Write(0:w1416, 1:"OUTP?1") -> (6:w1417:errorcluster)  [unwired: 3 in, 1 out]
                  n794 = GPIB Read(0:w1416, 1:3200, 3:w1417) -> (5:w1414:string)  [unwired: 2 in, 2 out]
                  n795 = Fract/Exp String To Number(string=w1414) -> (number=w1413:dbl)  [unwired: 3 in, 1 out]
                  n796 = Build Array (concatenate)(w1419, w1413) -> (w1418:dbl[])
                }
              }
              n797 = property on="array for data" class="Arr (strict)"("Value"=w1409) -> ()  [unwired: 2 in, 2 out]
            }
            frame #4 {
              # "check if out-of-phase\nsignal on lock-in \n(address 2) is to\nbe measured"
              n798 = property on="Addr 2 lock-in oop" class="Bool (strict)"() -> ("Value"=w1420:bool)  [unwired: 2 in, 2 out]
              n799 = property on="array for data" class="Arr (strict)"() -> ("Value"=w1422:dbl[])  [unwired: 2 in, 2 out]
              n800 = case shown="False" w1420 {
                tunnel: w1422 -> [w1423 w1431]
                tunnel: [w1423 w1430] -> w1421
                tunnel: w1420 -> [_ _]
                frame False {
                  # "we are not measuring out-of-phase signal on lock-in (address 2)"
                }
                frame True {
                  w1428 = "2"
                  # "we are  measuring lock-in (address 2), out-of-phase"
                  n801 = GPIB Write(0:w1428, 1:"OUTP?2") -> (6:w1429:errorcluster)  [unwired: 3 in, 1 out]
                  n802 = GPIB Read(0:w1428, 1:3200, 3:w1429) -> (5:w1426:string)  [unwired: 2 in, 2 out]
                  n803 = Fract/Exp String To Number(string=w1426) -> (number=w1425:dbl)  [unwired: 3 in, 1 out]
                  n804 = Build Array (concatenate)(w1431, w1425) -> (w1430:dbl[])
                }
              }
              n805 = property on="array for data" class="Arr (strict)"("Value"=w1421) -> ()  [unwired: 2 in, 2 out]
            }
            frame #5 {
              # "check if in-phase\nsignal on lock-in \n(address 3) is to\nbe measured"
              n806 = property on="Addr 3 lock-in" class="Bool (strict)"() -> ("Value"=w1432:bool)  [unwired: 2 in, 2 out]
              n807 = property on="array for data" class="Arr (strict)"() -> ("Value"=w1434:dbl[])  [unwired: 2 in, 2 out]
              n808 = case shown="False" w1432 {
                tunnel: w1434 -> [w1435 w1443]
                tunnel: [w1435 w1442] -> w1433
                frame False {
                  # "we are not measuring in phase signal on lock-in (address 3)"
                }
                frame True {
                  w1440 = "3"
                  # "we are  measuring lock-in (address 3), in phase"
                  n809 = GPIB Write(0:w1440, 1:"OUTP?1") -> (6:w1441:errorcluster)  [unwired: 3 in, 1 out]
                  n810 = GPIB Read(0:w1440, 1:3200, 3:w1441) -> (5:w1438:string)  [unwired: 2 in, 2 out]
                  n811 = Fract/Exp String To Number(string=w1438) -> (number=w1437:dbl)  [unwired: 3 in, 1 out]
                  n812 = Build Array (concatenate)(w1443, w1437) -> (w1442:dbl[])
                }
              }
              n813 = property on="array for data" class="Arr (strict)"("Value"=w1433) -> ()  [unwired: 2 in, 2 out]
            }
            frame #6 {
              # "check if out-of-phase\nsignal on lock-in \n(address 3) is to\nbe measured"
              n814 = property on="Addr 3 lock-in oop" class="Bool (strict)"() -> ("Value"=w1444:bool)  [unwired: 2 in, 2 out]
              n815 = property on="array for data" class="Arr (strict)"() -> ("Value"=w1446:dbl[])  [unwired: 2 in, 2 out]
              n816 = case shown="False" w1444 {
                tunnel: w1446 -> [w1447 w1455]
                tunnel: [w1447 w1454] -> w1445
                frame False {
                  # "we are not measuring out-of-phase signal on lock-in (address 3)"
                }
                frame True {
                  w1452 = "3"
                  # "we are  measuring lock-in (address 3), out-of-phase"
                  n817 = GPIB Write(0:w1452, 1:"OUTP?2") -> (6:w1453:errorcluster)  [unwired: 3 in, 1 out]
                  n818 = GPIB Read(0:w1452, 1:3200, 3:w1453) -> (5:w1450:string)  [unwired: 2 in, 2 out]
                  n819 = Fract/Exp String To Number(string=w1450) -> (number=w1449:dbl)  [unwired: 3 in, 1 out]
                  n820 = Build Array (concatenate)(w1455, w1449) -> (w1454:dbl[])
                }
              }
              n821 = property on="array for data" class="Arr (strict)"("Value"=w1445) -> ()  [unwired: 2 in, 2 out]
            }
            frame #7 {
              # "check if in-phase\nsignal on lock-in \n(address 4) is to\nbe measured"
              n822 = property on="Addr 4 lock-in" class="Bool (strict)"() -> ("Value"=w1456:bool)  [unwired: 2 in, 2 out]
              n823 = property on="array for data" class="Arr (strict)"() -> ("Value"=w1458:dbl[])  [unwired: 2 in, 2 out]
              n824 = case shown="False" w1456 {
                tunnel: w1458 -> [w1459 w1467]
                tunnel: [w1459 w1466] -> w1457
                frame False {
                  # "we are not measuring in phase signal on lock-in (address 4)"
                }
                frame True {
                  w1464 = "4"
                  # "we are  measuring lock-in (address 4), in phase"
                  n825 = GPIB Write(0:w1464, 1:"OUTP?1") -> (6:w1465:errorcluster)  [unwired: 3 in, 1 out]
                  n826 = GPIB Read(0:w1464, 1:3200, 3:w1465) -> (5:w1462:string)  [unwired: 2 in, 2 out]
                  n827 = Fract/Exp String To Number(string=w1462) -> (number=w1461:dbl)  [unwired: 3 in, 1 out]
                  n828 = Build Array (concatenate)(w1467, w1461) -> (w1466:dbl[])
                }
              }
              n829 = property on="array for data" class="Arr (strict)"("Value"=w1457) -> ()  [unwired: 2 in, 2 out]
            }
            frame #8 {
              # "check if out-of-phase\nsignal on lock-in \n(address 4) is to\nbe measured"
              n830 = property on="Addr 4 lock-in oop" class="Bool (strict)"() -> ("Value"=w1468:bool)  [unwired: 2 in, 2 out]
              n831 = property on="array for data" class="Arr (strict)"() -> ("Value"=w1470:dbl[])  [unwired: 2 in, 2 out]
              n832 = case shown="False" w1468 {
                tunnel: w1470 -> [w1471 w1479]
                tunnel: [w1471 w1478] -> w1469
                frame False {
                  # "we are not measuring out-of-phase signal on lock-in (address 4)"
                }
                frame True {
                  w1476 = "4"
                  # "we are  measuring lock-in (address 4), out-of-phase"
                  n833 = GPIB Write(0:w1476, 1:"OUTP?2") -> (6:w1477:errorcluster)  [unwired: 3 in, 1 out]
                  n834 = GPIB Read(0:w1476, 1:3200, 3:w1477) -> (5:w1474:string)  [unwired: 2 in, 2 out]
                  n835 = Fract/Exp String To Number(string=w1474) -> (number=w1473:dbl)  [unwired: 3 in, 1 out]
                  n836 = Build Array (concatenate)(w1479, w1473) -> (w1478:dbl[])
                }
              }
              n837 = property on="array for data" class="Arr (strict)"("Value"=w1469) -> ()  [unwired: 2 in, 2 out]
            }
            frame #9 {
              # "check if in-phase\nsignal on lock-in \n(address 5) is to\nbe measured"
              n838 = property on="Addr 5 lock-in" class="Bool (strict)"() -> ("Value"=w1480:bool)  [unwired: 2 in, 2 out]
              n839 = property on="array for data" class="Arr (strict)"() -> ("Value"=w1482:dbl[])  [unwired: 2 in, 2 out]
              n840 = case shown="False" w1480 {
                tunnel: w1482 -> [w1483 w1491]
                tunnel: [w1483 w1490] -> w1481
                frame False {
                  # "we are not measuring in phase signal on lock-in (address 5)"
                }
                frame True {
                  w1488 = "5"
                  # "we are  measuring lock-in (address 5), in phase"
                  n841 = GPIB Write(0:w1488, 1:"OUTP?1") -> (6:w1489:errorcluster)  [unwired: 3 in, 1 out]
                  n842 = GPIB Read(0:w1488, 1:3200, 3:w1489) -> (5:w1486:string)  [unwired: 2 in, 2 out]
                  n843 = Fract/Exp String To Number(string=w1486) -> (number=w1485:dbl)  [unwired: 3 in, 1 out]
                  n844 = Build Array (concatenate)(w1491, w1485) -> (w1490:dbl[])
                }
              }
              n845 = property on="array for data" class="Arr (strict)"("Value"=w1481) -> ()  [unwired: 2 in, 2 out]
            }
            frame #10 {
              # "check if out-of-phase\nsignal on lock-in \n(address 5) is to\nbe measured"
              n846 = property on="Addr 5 lock-in oop" class="Bool (strict)"() -> ("Value"=w1492:bool)  [unwired: 2 in, 2 out]
              n847 = property on="array for data" class="Arr (strict)"() -> ("Value"=w1494:dbl[])  [unwired: 2 in, 2 out]
              n848 = case shown="False" w1492 {
                tunnel: w1494 -> [w1495 w1503]
                tunnel: [w1495 w1502] -> w1493
                frame False {
                  # "we are not measuring out-of-phase signal on lock-in (address 5)"
                }
                frame True {
                  w1500 = "5"
                  # "we are  measuring lock-in (address 5), out-of-phase"
                  n849 = GPIB Write(0:w1500, 1:"OUTP?2") -> (6:w1501:errorcluster)  [unwired: 3 in, 1 out]
                  n850 = GPIB Read(0:w1500, 1:3200, 3:w1501) -> (5:w1498:string)  [unwired: 2 in, 2 out]
                  n851 = Fract/Exp String To Number(string=w1498) -> (number=w1497:dbl)  [unwired: 3 in, 1 out]
                  n852 = Build Array (concatenate)(w1503, w1497) -> (w1502:dbl[])
                }
              }
              n853 = property on="array for data" class="Arr (strict)"("Value"=w1493) -> ()  [unwired: 2 in, 2 out]
            }
            frame #11 {
              # "check if voltage on \nmain Keithley 2400 \n(addr. 12) is to\nbe measured"
              n854 = property on="Voltage (Vk1)" class="Bool (strict)"() -> ("Value"=w1504:bool)  [unwired: 2 in, 2 out]
              n855 = property on="array for data" class="Arr (strict)"() -> ("Value"=w1506:dbl[])  [unwired: 2 in, 2 out]
              n856 = case shown="False" w1504 {
                tunnel: w1506 -> [w1507 w1517]
                tunnel: [w1507 w1516] -> w1505
                frame False {
                  # "we aren't measuring voltage \non main Keithley 2400 (addr. 12)"
                }
                frame True {
                  w1514 = "12"
                  # "we are measuring voltage \non main Keithley 2400 (addr. 12)"
                  n857 = GPIB Write(0:w1514, 1:":READ?") -> (6:w1515:errorcluster)  [unwired: 3 in, 1 out]
                  n858 = GPIB Read(0:w1514, 1:3200, 3:w1515) -> (5:w1510:string)  [unwired: 2 in, 2 out]
                  n859 = String Subset(string=w1510, length (rest)=13) -> (substring=w1509:string)  [unwired: 1 in]
                  n860 = Fract/Exp String To Number(string=w1509) -> (number=w1512:dbl)  [unwired: 3 in, 1 out]
                  n861 = Build Array (concatenate)(w1517, w1512) -> (w1516:dbl[])
                }
              }
              n862 = property on="array for data" class="Arr (strict)"("Value"=w1505) -> ()  [unwired: 2 in, 2 out]
            }
            frame #12 {
              # "check if  current on \nmain Keithley 2400 \n(addr. 12) is to\nbe measured"
              n863 = property on="Current (Ik1)" class="Bool (strict)"() -> ("Value"=w1518:bool)  [unwired: 2 in, 2 out]
              n864 = property on="array for data" class="Arr (strict)"() -> ("Value"=w1520:dbl[])  [unwired: 2 in, 2 out]
              n865 = case shown="True" w1518 {
                tunnel: w1520 -> [w1521 w1532]
                tunnel: [w1521 w1531] -> w1519
                frame False {
                  # "we aren't measuring current \non main Keithley 2400 (addr. 12)"
                }
                frame True {
                  w1529 = "12"
                  # "we are measuring current\non main Keithley 2400 (addr. 12)"
                  n866 = GPIB Write(0:w1529, 1:":READ?") -> (6:w1530:errorcluster)  [unwired: 3 in, 1 out]
                  n867 = GPIB Read(0:w1529, 1:3200, 3:w1530) -> (5:w1525:string)  [unwired: 2 in, 2 out]
                  n868 = String Subset(string=w1525, offset (0)=14, length (rest)=13) -> (substring=w1524:string)
                  n869 = Fract/Exp String To Number(string=w1524) -> (number=w1527:dbl)  [unwired: 3 in, 1 out]
                  n870 = Build Array (concatenate)(w1532, w1527) -> (w1531:dbl[])
                }
              }
              n871 = property on="array for data" class="Arr (strict)"("Value"=w1519) -> ()  [unwired: 2 in, 2 out]
            }
            frame #13 {
              # "check if voltage on \nadd. Keithley 2400 \n(addr. 13) is to\nbe measured"
              n872 = property on="Voltage (Vk2)" class="Bool (strict)"() -> ("Value"=w1533:bool)  [unwired: 2 in, 2 out]
              n873 = property on="array for data" class="Arr (strict)"() -> ("Value"=w1535:dbl[])  [unwired: 2 in, 2 out]
              n874 = case shown="True" w1533 {
                tunnel: w1535 -> [w1536 w1546]
                tunnel: [w1536 w1545] -> w1534
                frame False {
                  # "we aren't measuring voltage \non additional Keithley 2400 (addr. 13)"
                }
                frame True {
                  w1543 = "13"
                  # "we are measuring voltage \non additional Keithley 2400 (addr. 13)"
                  n875 = GPIB Write(0:w1543, 1:":READ?") -> (6:w1544:errorcluster)  [unwired: 3 in, 1 out]
                  n876 = GPIB Read(0:w1543, 1:3200, 3:w1544) -> (5:w1539:string)  [unwired: 2 in, 2 out]
                  n877 = String Subset(string=w1539, length (rest)=13) -> (substring=w1538:string)  [unwired: 1 in]
                  n878 = Fract/Exp String To Number(string=w1538) -> (number=w1541:dbl)  [unwired: 3 in, 1 out]
                  n879 = Build Array (concatenate)(w1546, w1541) -> (w1545:dbl[])
                }
              }
              n880 = property on="array for data" class="Arr (strict)"("Value"=w1534) -> ()  [unwired: 2 in, 2 out]
            }
            frame #14 {
              # "check if  current on \nadd. Keithley 2400 \n(addr. 13) is to\nbe measured"
              n881 = property on="Current (Ik2)" class="Bool (strict)"() -> ("Value"=w1547:bool)  [unwired: 2 in, 2 out]
              n882 = property on="array for data" class="Arr (strict)"() -> ("Value"=w1549:dbl[])  [unwired: 2 in, 2 out]
              n883 = case shown="False" w1547 {
                tunnel: w1549 -> [w1550 w1561]
                tunnel: [w1550 w1560] -> w1548
                frame False {
                  # "we aren't measuring current \non additional Keithley 2400 (addr. 13)"
                }
                frame True {
                  w1558 = "13"
                  # "we are measuring current\non additional Keithley 2400 (addr. 13)"
                  n884 = GPIB Write(0:w1558, 1:":READ?") -> (6:w1559:errorcluster)  [unwired: 3 in, 1 out]
                  n885 = GPIB Read(0:w1558, 1:3200, 3:w1559) -> (5:w1554:string)  [unwired: 2 in, 2 out]
                  n886 = String Subset(string=w1554, offset (0)=14, length (rest)=13) -> (substring=w1553:string)
                  n887 = Fract/Exp String To Number(string=w1553) -> (number=w1556:dbl)  [unwired: 3 in, 1 out]
                  n888 = Build Array (concatenate)(w1561, w1556) -> (w1560:dbl[])
                }
              }
              n889 = property on="array for data" class="Arr (strict)"("Value"=w1548) -> ()  [unwired: 2 in, 2 out]
            }
            frame #15 {
              # "check if voltage on \nadd. Keithley 2400 \n(addr. 14) is to\nbe measured"
              n890 = property on="Voltage (Vk3)" class="Bool (strict)"() -> ("Value"=w1562:bool)  [unwired: 2 in, 2 out]
              n891 = property on="array for data" class="Arr (strict)"() -> ("Value"=w1564:dbl[])  [unwired: 2 in, 2 out]
              n892 = case shown="False" w1562 {
                tunnel: w1564 -> [w1565 w1575]
                tunnel: [w1565 w1574] -> w1563
                frame False {
                  # "we aren't measuring voltage \non additional Keithley 2400 (addr. 14)"
                }
                frame True {
                  w1572 = "14"
                  # "we are measuring voltage \non additional Keithley 2400 (addr. 14)"
                  n893 = GPIB Write(0:w1572, 1:":READ?") -> (6:w1573:errorcluster)  [unwired: 3 in, 1 out]
                  n894 = GPIB Read(0:w1572, 1:3200, 3:w1573) -> (5:w1568:string)  [unwired: 2 in, 2 out]
                  n895 = String Subset(string=w1568, length (rest)=13) -> (substring=w1567:string)  [unwired: 1 in]
                  n896 = Fract/Exp String To Number(string=w1567) -> (number=w1570:dbl)  [unwired: 3 in, 1 out]
                  n897 = Build Array (concatenate)(w1575, w1570) -> (w1574:dbl[])
                }
              }
              n898 = property on="array for data" class="Arr (strict)"("Value"=w1563) -> ()  [unwired: 2 in, 2 out]
            }
            frame #16 {
              # "check if  current on \nadd. Keithley 2400 \n(addr. 14) is to\nbe measured"
              n899 = property on="Current (Ik3)" class="Bool (strict)"() -> ("Value"=w1576:bool)  [unwired: 2 in, 2 out]
              n900 = property on="array for data" class="Arr (strict)"() -> ("Value"=w1578:dbl[])  [unwired: 2 in, 2 out]
              n901 = case shown="True" w1576 {
                tunnel: w1578 -> [w1579 w1590]
                tunnel: [w1579 w1589] -> w1577
                frame False {
                  # "we aren't measuring current \non additional Keithley 2400 (addr. 14)"
                }
                frame True {
                  w1587 = "14"
                  # "we are measuring current\non additional Keithley 2400 (addr. 14)"
                  n902 = GPIB Write(0:w1587, 1:":READ?") -> (6:w1588:errorcluster)  [unwired: 3 in, 1 out]
                  n903 = GPIB Read(0:w1587, 1:3200, 3:w1588) -> (5:w1583:string)  [unwired: 2 in, 2 out]
                  n904 = String Subset(string=w1583, offset (0)=14, length (rest)=13) -> (substring=w1582:string)
                  n905 = Fract/Exp String To Number(string=w1582) -> (number=w1585:dbl)  [unwired: 3 in, 1 out]
                  n906 = Build Array (concatenate)(w1590, w1585) -> (w1589:dbl[])
                }
              }
              n907 = property on="array for data" class="Arr (strict)"("Value"=w1577) -> ()  [unwired: 2 in, 2 out]
            }
            frame #17 {
              # "check if 1st channel\non Keithley 2182 \n(addr. 15) is to\nbe measured"
              n908 = property on="Channel 1 (Vnano1)" class="Bool (strict)"() -> ("Value"=w1591:bool)  [unwired: 2 in, 2 out]
              n909 = property on="array for data" class="Arr (strict)"() -> ("Value"=w1593:dbl[])  [unwired: 2 in, 2 out]
              n910 = case shown="True" w1591 {
                tunnel: w1593 -> [w1594 w1602]
                tunnel: [w1594 w1601] -> w1592
                frame False {
                  # "we are not measuring 1st channel\non Keithley 2182 (addr. 15)"
                }
                frame True {
                  w1599 = "15"
                  # "we are measuring 1st channel\non Keithley 2182 (addr. 15)"
                  n911 = GPIB Write(0:w1599, 1:":SENSe:DATA:FRES?") -> (6:w1600:errorcluster)  [unwired: 3 in, 1 out]
                  n912 = GPIB Read(0:w1599, 1:200, 3:w1600) -> (5:w1595:string)  [unwired: 2 in, 2 out]
                  n913 = Fract/Exp String To Number(string=w1595) -> (number=w1597:dbl)  [unwired: 3 in, 1 out]
                  n914 = Build Array (concatenate)(w1602, w1597) -> (w1601:dbl[])
                }
              }
              n915 = property on="array for data" class="Arr (strict)"("Value"=w1592) -> ()  [unwired: 2 in, 2 out]
            }
            frame #18 {
              # "check if 2nd channel\non Keithley 2182 \n(addr. 15) is to\nbe measured"
              n916 = property on="Channel 2 (Vnano1b)" class="Bool (strict)"() -> ("Value"=w1603:bool)  [unwired: 2 in, 2 out]
              n917 = property on="array for data" class="Arr (strict)"() -> ("Value"=w1605:dbl[])  [unwired: 2 in, 2 out]
              n918 = case shown="False" w1603 {
                tunnel: w1605 -> [w1606 w1618]
                tunnel: [w1606 w1617] -> w1604
                frame False {
                  # "we are not measuring 1st channel\non Keithley 2182 (addr. 15)"
                }
                frame True {
                  w1609 = "15"
                  # "switching to channel 2 and then\nback to channel 1"
                  # "we are measuring 2nd channel\non Keithley 2182 (addr. 15)"
                  n919 = GPIB Write(0:w1609, 1:":SENSe:CHAN 2") -> (6:w1610:errorcluster)  [unwired: 3 in, 1 out]
                  n920 = GPIB Write(0:w1609, 1:":SENSe:DATA:FRES?", 3:w1610) -> (6:w1616:errorcluster)  [unwired: 2 in, 1 out]
                  n921 = GPIB Read(0:w1609, 1:200, 3:w1616) -> (5:w1612:string, 7:w1608:errorcluster)  [unwired: 2 in, 1 out]
                  n922 = GPIB Write(0:w1609, 1:":SENSe:CHAN 1", 3:w1608) -> ()  [unwired: 2 in, 2 out]
                  n923 = Fract/Exp String To Number(string=w1612) -> (number=w1614:dbl)  [unwired: 3 in, 1 out]
                  n924 = Build Array (concatenate)(w1618, w1614) -> (w1617:dbl[])
                }
              }
              n925 = property on="array for data" class="Arr (strict)"("Value"=w1604) -> ()  [unwired: 2 in, 2 out]
            }
            frame #19 {
              # "check if 1st channel\non Keithley 2182 \n(addr. 16) is to\nbe measured"
              n926 = property on="Channel 1 (Vnano2)" class="Bool (strict)"() -> ("Value"=w1619:bool)  [unwired: 2 in, 2 out]
              n927 = property on="array for data" class="Arr (strict)"() -> ("Value"=w1621:dbl[])  [unwired: 2 in, 2 out]
              n928 = case shown="True" w1619 {
                tunnel: w1621 -> [w1622 w1630]
                tunnel: [w1622 w1629] -> w1620
                frame False {
                  # "we are not measuring 1st channel\non Keithley 2182 (addr. 16)"
                }
                frame True {
                  w1627 = "16"
                  # "we are measuring 1st channel\non Keithley 2182 (addr. 16)"
                  n929 = GPIB Write(0:w1627, 1:":SENSe:DATA:FRES?") -> (6:w1628:errorcluster)  [unwired: 3 in, 1 out]
                  n930 = GPIB Read(0:w1627, 1:200, 3:w1628) -> (5:w1623:string)  [unwired: 2 in, 2 out]
                  n931 = Fract/Exp String To Number(string=w1623) -> (number=w1625:dbl)  [unwired: 3 in, 1 out]
                  n932 = Build Array (concatenate)(w1630, w1625) -> (w1629:dbl[])
                }
              }
              n933 = property on="array for data" class="Arr (strict)"("Value"=w1620) -> ()  [unwired: 2 in, 2 out]
            }
            frame #20 {
              # "check if 2nd channel\non Keithley 2182 \n(addr. 16) is to\nbe measured"
              n934 = property on="Channel 2 (Vnano2b)" class="Bool (strict)"() -> ("Value"=w1631:bool)  [unwired: 2 in, 2 out]
              n935 = property on="array for data" class="Arr (strict)"() -> ("Value"=w1633:dbl[])  [unwired: 2 in, 2 out]
              n936 = case shown="False" w1631 {
                tunnel: w1633 -> [w1634 w1646]
                tunnel: [w1634 w1645] -> w1632
                frame False {
                  # "we are not measuring 1st channel\non Keithley 2182 (addr. 16)"
                }
                frame True {
                  w1637 = "16"
                  # "switching to channel 2 and then\nback to channel 1"
                  # "we are measuring 2nd channel\non Keithley 2182 (addr. 16)"
                  n937 = GPIB Write(0:w1637, 1:":SENSe:CHAN 2") -> (6:w1638:errorcluster)  [unwired: 3 in, 1 out]
                  n938 = GPIB Write(0:w1637, 1:":SENSe:DATA:FRES?", 3:w1638) -> (6:w1644:errorcluster)  [unwired: 2 in, 1 out]
                  n939 = GPIB Read(0:w1637, 1:200, 3:w1644) -> (5:w1640:string, 7:w1636:errorcluster)  [unwired: 2 in, 1 out]
                  n940 = GPIB Write(0:w1637, 1:":SENSe:CHAN 1", 3:w1636) -> ()  [unwired: 2 in, 2 out]
                  n941 = Fract/Exp String To Number(string=w1640) -> (number=w1642:dbl)  [unwired: 3 in, 1 out]
                  n942 = Build Array (concatenate)(w1646, w1642) -> (w1645:dbl[])
                }
              }
              n943 = property on="array for data" class="Arr (strict)"("Value"=w1632) -> ()  [unwired: 2 in, 2 out]
            }
            frame #21 {
              # "check if 1st channel\non Keithley 2182 \n(addr. 17) is to\nbe measured"
              n944 = property on="Channel 1 (Vnano3)" class="Bool (strict)"() -> ("Value"=w1647:bool)  [unwired: 2 in, 2 out]
              n945 = property on="array for data" class="Arr (strict)"() -> ("Value"=w1649:dbl[])  [unwired: 2 in, 2 out]
              n946 = case shown="False" w1647 {
                tunnel: w1649 -> [w1650 w1658]
                tunnel: [w1650 w1657] -> w1648
                frame False {
                  # "we are not measuring 1st channel\non Keithley 2182 (addr. 17)"
                }
                frame True {
                  w1655 = "17"
                  # "we are measuring 1st channel\non Keithley 2182 (addr. 17)"
                  n947 = GPIB Write(0:w1655, 1:":SENSe:DATA:FRES?") -> (6:w1656:errorcluster)  [unwired: 3 in, 1 out]
                  n948 = GPIB Read(0:w1655, 1:200, 3:w1656) -> (5:w1651:string)  [unwired: 2 in, 2 out]
                  n949 = Fract/Exp String To Number(string=w1651) -> (number=w1653:dbl)  [unwired: 3 in, 1 out]
                  n950 = Build Array (concatenate)(w1658, w1653) -> (w1657:dbl[])
                }
              }
              n951 = property on="array for data" class="Arr (strict)"("Value"=w1648) -> ()  [unwired: 2 in, 2 out]
            }
            frame #22 {
              # "check if 2nd channel\non Keithley 2182 \n(addr. 17) is to\nbe measured"
              n952 = property on="Channel 2 (Vnano3b)" class="Bool (strict)"() -> ("Value"=w1659:bool)  [unwired: 2 in, 2 out]
              n953 = property on="array for data" class="Arr (strict)"() -> ("Value"=w1661:dbl[])  [unwired: 2 in, 2 out]
              n954 = case shown="False" w1659 {
                tunnel: w1661 -> [w1662 w1674]
                tunnel: [w1662 w1673] -> w1660
                frame False {
                  # "we are not measuring 1st channel\non Keithley 2182 (addr. 17)"
                }
                frame True {
                  w1665 = "17"
                  # "switching to channel 2 and then\nback to channel 1"
                  # "we are measuring 2nd channel\non Keithley 2182 (addr. 17)"
                  n955 = GPIB Write(0:w1665, 1:":SENSe:CHAN 2") -> (6:w1666:errorcluster)  [unwired: 3 in, 1 out]
                  n956 = GPIB Write(0:w1665, 1:":SENSe:DATA:FRES?", 3:w1666) -> (6:w1672:errorcluster)  [unwired: 2 in, 1 out]
                  n957 = GPIB Read(0:w1665, 1:200, 3:w1672) -> (5:w1668:string, 7:w1664:errorcluster)  [unwired: 2 in, 1 out]
                  n958 = GPIB Write(0:w1665, 1:":SENSe:CHAN 1", 3:w1664) -> ()  [unwired: 2 in, 2 out]
                  n959 = Fract/Exp String To Number(string=w1668) -> (number=w1670:dbl)  [unwired: 3 in, 1 out]
                  n960 = Build Array (concatenate)(w1674, w1670) -> (w1673:dbl[])
                }
              }
              n961 = property on="array for data" class="Arr (strict)"("Value"=w1660) -> ()  [unwired: 2 in, 2 out]
            }
            frame #23 {
              # "check if 1st \nthermometer on \nOxford ITC \n(address 24) \nis measured"
              n962 = property on="Thermometer 1 (T1)" class="Bool (strict)"() -> ("Value"=w1675:bool)  [unwired: 2 in, 2 out]
              n963 = property on="array for data" class="Arr (strict)"() -> ("Value"=w1677:dbl[])  [unwired: 2 in, 2 out]
              n964 = case shown="True" w1675 {
                tunnel: w1677 -> [w1678 w1687]
                tunnel: [w1678 w1686] -> w1676
                frame False {
                  # "we are not measuring temperature on\nthermometer 1 (addr. 24)"
                }
                frame True {
                  w1679 = 1
                  w1684 = "24"
                  # "we are measuring temperature,\nthermometer 1 (addr. 24)"
                  n965 = GPIB Write(0:w1684, 1:"R 1", 2:w1679) -> (6:w1685:errorcluster)  [unwired: 2 in, 1 out]
                  n966 = GPIB Read(0:w1684, 1:200, 2:w1679, 3:w1685) -> (5:w1680:string)  [unwired: 1 in, 2 out]
                  n967 = Fract/Exp String To Number(string=w1680, offset=w1679) -> (number=w1682:dbl)  [unwired: 2 in, 1 out]
                  n968 = Build Array (concatenate)(w1687, w1682) -> (w1686:dbl[])
                }
              }
              n969 = property on="array for data" class="Arr (strict)"("Value"=w1676) -> ()  [unwired: 2 in, 2 out]
            }
            frame #24 {
              # "check if 1st \nthermometer on \nOxford ITC \n(address 24) \nis measured"
              n970 = property on="Magnetic Field (B)" class="Bool (strict)"() -> ("Value"=w1688:bool)  [unwired: 2 in, 2 out]
              n971 = property on="array for data" class="Arr (strict)"() -> ("Value"=w1690:dbl[])  [unwired: 2 in, 2 out]
              n972 = case shown="True" w1688 {
                tunnel: w1690 -> [w1691 w1700]
                tunnel: [w1691 w1699] -> w1689
                frame False {
                  # "we are not measuringmagnetic field (addr. 25)"
                }
                frame True {
                  w1692 = 1
                  w1697 = "25"
                  # "we are measuring magnetic field  (addr. 25)"
                  n973 = GPIB Write(0:w1697, 1:"R 7", 2:w1692) -> (6:w1698:errorcluster)  [unwired: 2 in, 1 out]
                  n974 = GPIB Read(0:w1697, 1:200, 2:w1692, 3:w1698) -> (5:w1693:string)  [unwired: 1 in, 2 out]
                  n975 = Fract/Exp String To Number(string=w1693, offset=w1692) -> (number=w1695:dbl)  [unwired: 2 in, 1 out]
                  n976 = Build Array (concatenate)(w1700, w1695) -> (w1699:dbl[])
                }
              }
              n977 = property on="array for data" class="Arr (strict)"("Value"=w1689) -> ()  [unwired: 2 in, 2 out]
            }
            frame #25 {
              # "check if capacitance\nand loss (address 28)\nare measured"
              n978 = property on="Capacitance (C) and Loss (L)" class="Bool (strict)"() -> ("Value"=w1701:bool)  [unwired: 2 in, 2 out]
              n979 = property on="array for data" class="Arr (strict)"() -> ("Value"=w1703:dbl[])  [unwired: 2 in, 2 out]
              n980 = case shown="True" w1701 {
                tunnel: w1703 -> [w1704 w1710]
                tunnel: [w1704 w1706] -> w1702
                frame False {
                  # "we are not measuringmagnetic capacitance (addr. 28)"
                }
                frame True {
                  # "we are measuring capacitance and loss  (addr. 28)"
                  n981 = stacked-sequence {
                    seq-local: [w1712 _ _] -> [_ _ w1735]
                    tunnel: [_ _ w1729] -> w1705
                    tunnel: [_ _ w1730] -> w1708
                    tunnel: "28" ("data") -> [w1711 w1715 w1724]
                    frame #0 {
                      n982 = GPIB Write(0:w1711, 1:"SINGLE" ("data"), 2:i16 0 ("mode (0)")) -> (6:w1712:errorcluster)  [unwired: 2 in, 1 out]
                    }
                    frame #1 {
                      n983 = while {
                        tunnel: w1715 -> [w1716]
                        i -> [w1717]
                        stop <- w1719 continue-if-true
                        n984 = GPIB Serial Poll(0:w1716) -> (2:w1721:i16)  [unwired: 1 in, 2 out]
                        n985 = Less?(x=w1721, y=i16 128) -> (x < y?=w1719:bool)
                        n986 = Wait (ms)(milliseconds to wait=u32 50) -> ()  [unwired: 1 out]
                        "Numeric 3" <- w1717
                      }
                    }
                    frame #2 {
                      w1722 = i16 2 ("mode (0)")
                      n987 = GPIB Read(0:w1724, 1:200 ("byte count"), 2:i16 2 ("mode (0)"), 3:w1735) -> (5:w1728:string)  [unwired: 1 in, 2 out]
                      n988 = Match Pattern(string=w1728, regular expression="C=") -> (after substring=w1727:string)  [unwired: 1 in, 3 out]
                      n989 = Match Pattern(string=w1727, regular expression="PF L=") -> (after substring=w1725:string)  [unwired: 1 in, 3 out]
                      n990 = Search/Split String(string=w1727, search string/char (-)=" ", offset (0)=w1722) -> (substring before match=w1732:string)  [unwired: 2 out]
                      n991 = Search/Split String(string=w1725, search string/char (-)=" ", offset (0)=w1722) -> (substring before match=w1731:string)  [unwired: 2 out]
                      n992 = Fract/Exp String To Number(string=w1731) -> (number=w1729:dbl)  [unwired: 3 in, 1 out]
                      n993 = Fract/Exp String To Number(string=w1732) -> (number=w1730:dbl)  [unwired: 3 in, 1 out]
                    }
                  }
                  n994 = Build Array (concatenate)(w1710, w1708) -> (w1707:dbl[])
                  n995 = Build Array (concatenate)(w1707, w1705) -> (w1706:dbl[])
                }
              }
              n996 = property on="array for data" class="Arr (strict)"("Value"=w1702) -> ()  [unwired: 2 in, 2 out]
            }
          }
        }
      }
      n997 = property on="array for data" class="Arr (strict)"(error in=w562) -> ("Value"=w540:dbl[])  [unwired: 1 in, 2 out]
      n998 = while {
        shift-right: [w1749] -> w536
        shift-left: w540 -> [w1751]
        i -> [w1750]
        stop <- w1754 stop-if-true
        # "loop goes through the list of all measured parameters\nif some columns are identified as current or resistance\nthey are recalculated according to selected or entered parameters"
        n999 = Increment(x=w1750) -> (x+1=w1755:i32)
        n1000 = property on="Ring" class="Ring (strict)"() -> ("Strings []"=w1753:string[])  [unwired: 2 in, 2 out]
        n1001 = Index Array(array=w1753, index=w1750) -> (element=w1752:string)
        n1002 = property on="Ring" class="Ring (strict)"() -> ("NumItems"=w1756:u32)  [unwired: 2 in, 2 out]
        n1003 = case shown="\"False\", Default" w1752 {
          tunnel: w1751 -> [w1762 w1772 w1782 w1789]
          tunnel: w1750 -> [w1760 w1769 w1780 _]
          tunnel: [w1761 w1770 w1781 w1789] -> w1749
          frame "I" {
            n1004 = property on="Current is:" class="RadioBtnsControl (strict)"() -> ("Value"=w1758:T1)  [unwired: 2 in, 2 out]
            n1005 = case shown="\"Radio Selection 2\"" w1758 {
              tunnel: ["Ring 3" "Ring 2"] -> w1757
              frame "Radio Selection 3", Default {
              }
              frame "Radio Selection 2" {
              }
            }
            n1006 = Index Array(array=w1762, index=w1760) -> (element=w1763:dbl)
            n1007 = Power Of 10(x=w1757) -> (10^x=w1766:dbl)
            n1008 = Multiply(x=1000.0, y=w1766) -> (x*y=w1764:dbl)
            n1009 = Divide(x=w1763, y=w1764) -> (x/y=w1759:dbl)
            "Numeric Current" <- w1759
            n1010 = Replace Array Subset(array=w1762, new element=w1759, index=w1760) -> (w1761:dbl[])
          }
          frame "Ioop" {
            n1011 = property on="Ring 3" class="Ring (strict)"() -> ("Value"=w1771:u16)  [unwired: 2 in, 2 out]
            n1012 = Index Array(array=w1772, index=w1769) -> (element=w1774:dbl)
            n1013 = Power Of 10(x=w1771) -> (10^x=w1777:dbl)
            n1014 = Multiply(x=1000.0, y=w1777) -> (x*y=w1775:dbl)
            n1015 = Divide(x=w1774, y=w1775) -> (x/y=w1773:dbl)
            n1016 = Replace Array Subset(array=w1772, new element=w1773, index=w1769) -> (w1770:dbl[])
          }
          frame "R1", "R1oop", "R2", "R2oop", "R3", "R3oop", "R4", "R4oop", "R5", "R5oop" {
            n1017 = property on="Current is:" class="RadioBtnsControl (strict)"() -> ("Value"=w1779:T1)  [unwired: 2 in, 2 out]
            n1018 = case shown="\"Radio Selection 2\", Default" w1779 {
              tunnel: [w1785 w1788] -> w1778
              frame "Radio Selection 1" {
                n1019 = Divide(x="Fixed Current mkA", y=1000000.0) -> (x/y=w1785:dbl)
              }
              frame "Radio Selection 2", Default {
                n1020 = property on="Numeric Current" class="DigNum (strict)"() -> ("Value"=w1788:dbl)  [unwired: 2 in, 2 out]
              }
            }
            n1021 = Index Array(array=w1782, index=w1780) -> (element=w1784:dbl)
            n1022 = Divide(x=w1784, y=w1778) -> (x/y=w1783:dbl)
            n1023 = Replace Array Subset(array=w1782, new element=w1783, index=w1780) -> (w1781:dbl[])
          }
          frame "False", Default {
          }
        }
        n1024 = Less?(x=w1756, y=w1755) -> (x < y?=w1754:bool)
      }
      n1025 = Subtract(x="Target Voltage, V", y=w546) -> (x-y=w549:dbl)
      n1026 = Divide(x="Sweep rate, V/min", y=60.0) -> (x/y=w558:dbl)
      n1027 = Multiply(x=w558, y="Time btw \npoints, sec") -> (x*y=w541:dbl)
      n1028 = Sign(1:w549) -> (0:w542:dbl)
      n1029 = Multiply(x=w542, y=w541) -> (x*y=w534:dbl)
      n1030 = property on="points at each Vg" class="DigNum (strict)"() -> ("Value"=w533:i32)  [unwired: 2 in, 2 out]
      n1031 = To Double Precision Float(number=w533) -> (double precision float=w532:dbl)
      n1032 = Multiply(x=w532, y=w534) -> (x*y=w531:dbl)
      n1033 = property on="Commutator" class="Bool (strict)"() -> ("Value"=w525:bool)  [unwired: 2 in, 2 out]
      n1034 = property on="Data file:" class="Path"() -> ("Value"=w538:path)  [unwired: 2 in, 2 out]
      n1035 = Divide(x=w549, y=w531) -> (x/y=w556:dbl)
      n1036 = case shown="False" w525 {
        tunnel: w543 -> [w576 w587]
        tunnel: w527 -> [w571 w581]
        tunnel: [w563 w580] -> w524
        frame True {
          # "calculate deliberate time delay for the next step"
          n1037 = Subtract(x=w576, y=w571) -> (x-y=w569:u32)
          n1038 = property on="Delib Time delay" class="DigNum (strict)"() -> ("Value"=w570:i32)  [unwired: 2 in, 2 out]
          n1039 = property on="Time btw \npoints, sec" class="DigNum (strict)"() -> ("Value"=w575:dbl)  [unwired: 2 in, 2 out]
          n1040 = Subtract(x=w569, y=w570) -> (x-y=w568:u32)
          n1041 = Multiply(x=w575, y=1000.0) -> (x*y=w573:dbl)
          n1042 = To Long Integer(number=w573) -> (32bit integer=w572:i32)
          n1043 = Greater?(x=w572, y=w568) -> (0:w565:bool)
          n1044 = Subtract(x=w572, y=w568) -> (x-y=w567:u32)
          n1045 = Divide(x=w567, y=2) -> (x/y=w564:dbl)
          n1046 = case shown="False" w565 {
            tunnel: w564 -> [_ w579]
            tunnel: [0 w578] -> w563
            frame False {
            }
            frame True {
              n1047 = To Long Integer(number=w579) -> (32bit integer=w578:i32)
            }
          }
        }
        frame False {
          # "calculate deliberate time delay for the next step"
          n1048 = Subtract(x=w587, y=w581) -> (x-y=w584:u32)
          n1049 = property on="Time btw \npoints, sec" class="DigNum (strict)"() -> ("Value"=w586:dbl)  [unwired: 2 in, 2 out]
          n1050 = Multiply(x=w586, y=1000.0) -> (x*y=w583:dbl)
          n1051 = To Long Integer(number=w583) -> (32bit integer=w582:i32)
          n1052 = Greater?(x=w582, y=w584) -> ()  [unwired: 1 out]
          n1053 = Subtract(x=w582, y=w584) -> (x-y=w580:u32)
        }
      }
      "Delib Time delay" <- w524
      n1054 = Decrement(x=w556) -> (x-1=w555:dbl)
      n1055 = Absolute Value(x=w549) -> (abs(x)=w551:dbl)
      n1056 = Build Array (concatenate)(w561, w536) -> (w535:dbl[][])
      n1057 = Greater Than 0?(x=w555) -> (x > 0?=w554:bool)
      n1058 = property on="array for data" class="Arr (strict)"("Value"=w536) -> ()  [unwired: 2 in, 2 out]
      n1059 = call-poly <vilib>:"Write To Spreadsheet File.vi"("format (%.3f)"="%#g", "append to file? (new file:F)"=TRUE, "1D data"=w536, "file path (dialog if empty)"=w538) -> ()  [unwired: 4 in, 1 out]
      n1060 = Less?(x=w551, y=1e-06) -> (x < y?=w548:bool)
      n1061 = flat-sequence {
        tunnel: [w1748] -> w543
        tunnel: w535 -> [w1742]
        frame #0 {
          # "time is mesured at the end of the cycle\nto adjust a delay time"
          # "this part plots selected measurements"
          n1062 = Tick Count (ms)() -> (millisecond timer value=w1748:u32)
          n1063 = Index Array(array=w1742, index (col)="Ring") -> (element=w1747:dbl[])  [unwired: 1 in]
          n1064 = Index Array(array=w1742, index (col)=0) -> (element=w1745:dbl[])  [unwired: 1 in]
          n1065 = Bundle(w1745, w1747) -> (→"XY Graph":cluster{dbl[], dbl[]})  [unwired: 1 in]
        }
      }
      n1066 = case shown="True" w554 {
        tunnel: w546 -> [_ w1793]
        tunnel: w531 -> [_ w1792]
        tunnel: [w1790 w1791] -> w553
        frame False {
          # "if next step is too long\nuse target voltage"
          n1067 = property on="Target Voltage, V" class="DigNum (strict)"() -> ("Value"=w1790:dbl)  [unwired: 2 in, 2 out]
        }
        frame True {
          # "add increment to\nthe current Vg"
          n1068 = Add(x=w1792, y=w1793) -> (x+y=w1791:dbl)
        }
      }
    }
    n1069 = Number To Fractional String(number=w503) -> (F-format string=w508:string)  [unwired: 3 in]
    n1070 = property on="Main Keithly2400 address" class="Str"() -> ("Value"=w506:string)  [unwired: 2 in, 2 out]
    n1071 = Concatenate Strings(":INIT:IMM; :SOUR:VOLT:LEV:IMM:AMPL " ("data"), w508) -> (w507:string)
    n1072 = Equal?(x=w501, y="optional Bias (V)") -> (x = y?=w504:bool)
    n1073 = case shown="False" w504 {
      tunnel: "optional Bias (V)" -> [w516 _]
      tunnel: w503 -> [w515 _]
      frame False {
        n1074 = Multiply(x=w515, y=22.62) -> (x*y=w517:dbl)
        n1075 = Number To Fractional String(number=w515) -> (F-format string=w523:string)  [unwired: 3 in]
        n1076 = Add(x=w516, y=w517) -> ()  [unwired: 1 out]
        n1077 = Concatenate Strings(":INIT:IMM; :SOUR:VOLT:LEV:IMM:AMPL " ("data"), w523) -> (w522:string)
        n1078 = property on="optional Bias (V)" class="DigNum (strict)"("Visible"=TRUE) -> ()  [unwired: 2 in, 2 out]
        n1079 = GPIB Write(0:"13", 1:w522) -> ()  [unwired: 3 in, 2 out]
      }
      frame True {
      }
    }
    n1080 = GPIB Write(0:w506, 1:w507) -> ()  [unwired: 3 in, 2 out]
  }
  "Array 2" <- w13
  n1081 = Write to Text File(file (use dialog)=w16, text=w15) -> ()  [unwired: 2 in, 3 out]
  n1082 = Array Size(array=w5) -> (size(s)=→"Numeric 2":i32)
  n1083 = property on="optional Bias (V)" class="DigNum (strict)"("Value"=w11, "Visible"=FALSE) -> ()  [unwired: 2 in, 2 out]
